vi "myRIO_BRig_RT_v0,70.vi"() -> ()   [LabVIEW 2014]
uses:
  <vilib>/Platform/TimedLoop/XDataNode/XDataNode.xnode
  <vilib>/Platform/TimedLoop/XDataNode/nitl_modes.ctl
  <vilib>/Platform/TimedLoop/XDataNode/XDNodeRunTimeDep.lvlib
  <vilib>/Platform/TimedLoop/XDataNode/wakeup.ctl
  <vilib>/Platform/TimedLoop/XDataNode/timing_clust.ctl
  <vilib>/rvi/interface/nirviReadWriteControl/nirviReadWriteControl.xnode
  <vilib>/rvi/interface/Simulation/niFpgaSimulationCallBeginRW.vi
  <vilib>/rvi/errors/niLvFpgaAdjustHostInterfaceError.vi
  <vilib>/rvi/interface/nirviCloseFPGA/nirviCloseFPGA.xnode
  <vilib>/myRIO/Instrument Drivers/Utilities/Utilities.lvlib
  <vilib>/rvi/interface/nirviOpenFPGA/nirviOpenFPGA.xnode
  myRIO_BRig_RT__Case_Exp_stateList.ctl
  <vilib>/WebDAVClient/Advanced/SessionHandle.ctl
  <vilib>/WebDAVClient/NI_WebDAV.lvlib
  myRIO_BRig_RT__Case_NonExp_stateList.ctl
  NiFpgaLv.dll
  <vilib>/Utility/error.llb/Error Cluster From Error Code.vi
  <vilib>/FPGAPlugInAG/Dynamic/niLvFpga_Close_Dynamic.vi
  myRIO_BRig_FPGA_v3,60__build.lvbitx
  myRIO_BRig_FPGA_v3,60.vi
  <vilib>/FPGAPlugInAG/myRIO-1900/niLvFpga_Open_myRIO-1900.vi
  <vilib>/rvi/interface/common/dynamic/niFpgaDynamicAddResources.vi
panel:
  out "tempAI0":u16
  out "error out 5":errorcluster
  in  "get_countPerMS":bool
  in  "count_warmup_R_reset":bool
  in  "count_warmup_L_reset":bool
  out "count_warmup_R":u16
  out "count_warmup_L":u16
  out "SolenoidReward":bool
  in  "SolenoidProbability_L":u16=50 caption="Reward Time [ms]" min=1 max=1000 step=1
  in  "SolenoidProbability_R":u16=50 caption="Reward Time [ms]" min=1 max=1000 step=1
  out "output_PortA":dbl caption="LaserPower"
  out "error out 4":errorcluster
  in  "laser_power_step":dbl
  in  "laser_power_max":dbl
  in  "Recording":bool
  out "error out 3":errorcluster
  out "error out 2":errorcluster
  in  "laser_power_min":dbl
  in  "f_millisec2count":dbl=159.0
  in  "laser_Tshutter":dbl=2.0
  in  "laser_Freq":dbl=10.0
  in  "laser_Tpeak":dbl=2.0
  in  "laser_duration":u16
  out "error out":errorcluster
  in  "LC_Cue1_All_Count":u16
  in  "LC_Cue1_First_Count":u16
  in  "LC_Cue1_All_delayOpt":bool
  in  "LC_ENL1_All_delayOpt":bool
  in  "LC_ENL1_All_Count":u16
  in  "LC_ENL1_First_Count":u16
  in  "LC_Cue1_First_delayOpt":bool
  in  "LC_ENL1_First_delayOpt":bool
  in  "Tcycle_Cue_max":u16=1000 caption="Max" min=5 max=5000 step=5
  in  "Tcycle_Cue_min":u16=1000 caption="Min" min=5 max=5000 step=5
  in  "SendData":bool
  out "cSpout":enum16{"Left", "Right"}(ring) caption="Left or Right Spout"
  out "A4":u32 caption="LickCounter_Right"
  out "A2":u32 caption="LickCounter_Left"
  in  "laserResponse_wrong_LED":bool
  out "error_initTrial":errorcluster
  out "error_Selection_pre":errorcluster
  out "error_Selection":errorcluster
  out "SelectWrong":bool
  out "SelectReward":bool
  in  "Left(F)_or_Right(T)":bool
  in  "ignoreWrong":bool
  in  "SelectionState":bool
  in  "laserResponse_wrong":bool
  in  "laserResponse_reward":bool
  in  "laserResponse_reward_LED":bool
  out "nRewards_Right":u16 caption="# Rewards Total (Right)"
  out "nRewards_Left":u16 caption="# Rewards Total (Left)"
  out "nRewards_cur":u16 caption="# Rewards in Current Block"
  out "TpB_target":u16 caption="Target Trials Per Block"
  out "cState_NonExp":T1 caption="WarmUp State"
  out "iBlock":u16 caption="Current Block"
  out "cState":T2 caption="Experimental State"
  out "iTrial":u16 caption="Current Trial"
  in  "warmupType":u8(slide) max=2 step=1 scale=0.0..2.0
  in  "TestConnection":bool
  in  "warmup":bool caption="WarmUp"
  in  "Data Set Prefix":string="Exp1_TM2"
  out "Connected To Host?":bool
  in  "Host Password":string="sabalab"
  in  "Host UserName":string="Test2"
  in  "sp_RightSpout":u16(slide)=2 max=2 step=1 scale=0.0..2.0
  in  "sp_LeftSpout":u16(slide)=2 max=2 step=1 scale=0.0..2.0
  in  "BUR_max":u16 caption="Count Reward Structure  (0 = off)"
  in  "LC_Wrong_Probability":u16
  in  "LC_Wrong_Trial":u16(slide) max=2 step=1 scale=0.0..2.0
  in  "LC_Wrong_Block":u16(slide) max=2 step=1 scale=0.0..2.0
  in  "LC_Wrong_OnOff":bool
  in  "LC_Reward_Probability":u16
  in  "LC_Reward_Trial":u16(slide) max=2 step=1 scale=0.0..2.0
  in  "LC_Reward_Block":u16(slide) max=2 step=1 scale=0.0..2.0
  in  "LC_Reward_OnOff":bool
  in  "LC_Cue1_All_Probability":u16
  in  "LC_Cue1_All_Block":u16(slide) max=2 step=1 scale=0.0..2.0
  in  "LC_Cue1_All_OnOff":bool
  in  "LC_Cue1_First_Probability":u16
  in  "LC_Cue1_First_Block":u16(slide) max=2 step=1 scale=0.0..2.0
  in  "LC_Cue1_First_OnOff":bool
  in  "LC_ENL1_All_Probability":u16 max=100 step=1
  in  "LC_ENL1_All_Block":u16(slide) max=2 step=1 scale=0.0..2.0
  in  "LC_ENL1_All_OnOff":bool
  in  "LC_ENL1_First_Probability":u16 max=100 step=1
  in  "LC_ENL1_First_Block":u16(slide) max=2 step=1 scale=0.0..2.0
  in  "Tcycle_Timeout":u16=1000 caption="Timeout Time [ms]" min=10 max=10000 step=1
  in  "Tcycle_Wrong":u16=1000 caption="Wrong Time [ms]" min=10 max=10000 step=1
  in  "Tcycle_Selection":u16=1000 caption="Answer Time [ms]" min=1 max=10000 step=1
  in  "Tcycle_RewardPost":u16=1000 caption="Consumption Time [ms]" min=250 max=10000 step=250
  in  "Tcycle_Reward_L":u16=500 caption="Reward Time [ms]" min=1 max=1000 step=1
  in  "Tcycle_Reward_R":u16=500 caption="Reward Time [ms]" min=1 max=1000 step=1
  in  "TpB_Max_R":u16=4 caption="Max TrialsPerBlock" min=1 max=12 step=1
  in  "TpB_Min_R":u16=4 caption="Min TrialsPerBlock" min=1 max=12 step=1
  in  "TpB_Max_L":u16=4 caption="Max TrialsPerBlock" min=1 max=12 step=1
  in  "TpB_Min_L":u16=4 caption="Min TrialsPerBlock" min=1 max=12 step=1
  in  "BUR_min":u16 caption="Count Reward Structure\n(0 = off)"
  in  "TrialUntilReward":bool caption="Ignore Wrong Selection"
  in  "CueCycles":u16=1 caption="Cue Structure" min=1 max=1 step=1
  in  "MTrig_Laser_Tcycle":u16=10 caption="Time [ms]"
  in  "MTrig_Laser_trig":bool
  in  "MTrig_Audio_trig__R":bool caption="Trigger Audio"
  in  "MTrig_Audio_trig__L":bool caption="Trigger Audio"
  in  "RewCalib_Trig_R":bool caption="Calibrate_R"
  in  "RewCalib_Trig_L":bool caption="Calibrate_L"
  in  "MTrig_Solenoid_Tcycle__R":u16=300 caption="Time [ms]"
  in  "MTrig_Solenoid_Tcycle__L":u16=300 caption="Time [ms]"
  in  "MTrig_Solenoid_trig__R":bool caption="Solenoid"
  in  "MTrig_Solenoid_trig__L":bool caption="Solenoid"
  in  "STOP_abort":bool caption="Stop LabView\n(Stops myRio and FPGA)"
  in  "STOP_endBlock":bool caption="Stop Experiment\n@ End of Block"
  in  "STOP_endTrial":bool caption="Stop Experiment\n@ End of Trial"
  in  "START":bool caption="Start Experiment"
  in  "Tcycle_CuePenalty":u16=1000 caption="Penalty" min=1 max=10000 step=1
  in  "Audio_Amp__R":u16=100 caption="Amp"
  in  "Audio_Freq__R":u8=5 caption="Freq [kHz]" max=14 step=1
  in  "Audio_Amp__L":u16=100 caption="Amp"
  in  "Audio_Freq__L":u8=5 caption="Freq [kHz]" max=14 step=1
  in  "LC_Wrong_Tdelay":u16
  in  "LC_Cue1_All_Tdelay":u16
  in  "LC_ENL1_All_Tdelay":u16
  in  "LC_Reward_Tdelay":u16
  in  "LC_Cue1_First_Tdelay":u16
  in  "LC_ENL1_First_Tdelay":u16
  in  "LC_ENL1_First_OnOff":bool
  in  "Tcycle_ENLPenalty":u16=100 caption="Penalty" min=10 max=10000 step=10
  in  "Tcycle_ENL_max":u16=1000 caption="Max" min=250 max=10000 step=250
  in  "Tcycle_ENL_min":u16=1000 caption="Min" min=250 max=10000 step=250
  # "Experimental Run"
  # "Experiment Task Structure"
  # "Current State"
  # "Timing [ms]"
  # "Global Parameters\n \n   WarmUp State                                            Lick Counter"
  # "Min            Max            Penalty"
  # "(1) = Switching\n(2) = Two Choice"
  # "Enforced\nNonLick"
  # "Left                    Right"
  # "Cue"
  # "Experimental State"
  # "Communication (Host PC)"
  # "WarmUp"
  # "Selection\n \n \nReward\n    Dispense\n    Time\n \n    Dispense\n    Probability\n \n    Consumption\n    Time\n \nWrong Choice\n \n \nTimeout Penalty"
  # "Trial Parameters\n \n   Left/Right        Give Reward?        Laser Power [V]"
  # "Left                  Right"
  # "Min"
  # "Max"
  # "Block                   Trial            Target Trials       # Rewards \n                                                            Per Block             Current"
  # "Trial Per Block Structure \n               Left                        Right"
  # "Min"
  # "# Rewards Total\n                                                                  Left                    Right"
  # "Recording Rig"
  # "FPGA Conv."
  # "Cue then reward (no lick)\n \nLeft                    Right"
  # "Max"
  # "FPGA count per ms"
  # "Laser Control\n\n                               On/Off      Block        Probability [%]   Delay [ms]                              Count"
  # "Manual Control"
  # "Enforced\nNonLick\n      1"
  # "Solenoid\n \nLeft              Right"
  # "Speaker\n \nLeft                    Right"
  # "Laser"
  # "from end"
  # "Switch\nTrial"
  # "from start"
  # "from end"
  # "NonSwitch\nTrials"
  # "Time\n[ms]"
  # "Time\n[ms]"
  # "from start"
  # "Time = Cue Min"
  # "Cue 1"
  # "Power = Min"
  # "from end"
  # "Switch\nTrial"
  # "from start"
  # "Speaker Parameters"
  # "Laser Parameters"
  # "Left                  Right"
  # "from end"
  # "Frequency\n[Hz]"
  # "NonSwitch\nTrials"
  # "Frequency\n[kHz]"
  # "from start"
  # "Timing [ms]\n Duration     Peak Width   Shutter"
  # "Selection Reward"
  # "Amp\n(0 - 32,000)"
  # "Laser Power [V]\nMin          Max              Step"
  # "Speaker\nPattern\nDuring Cue"
  # "Selection Wrong"
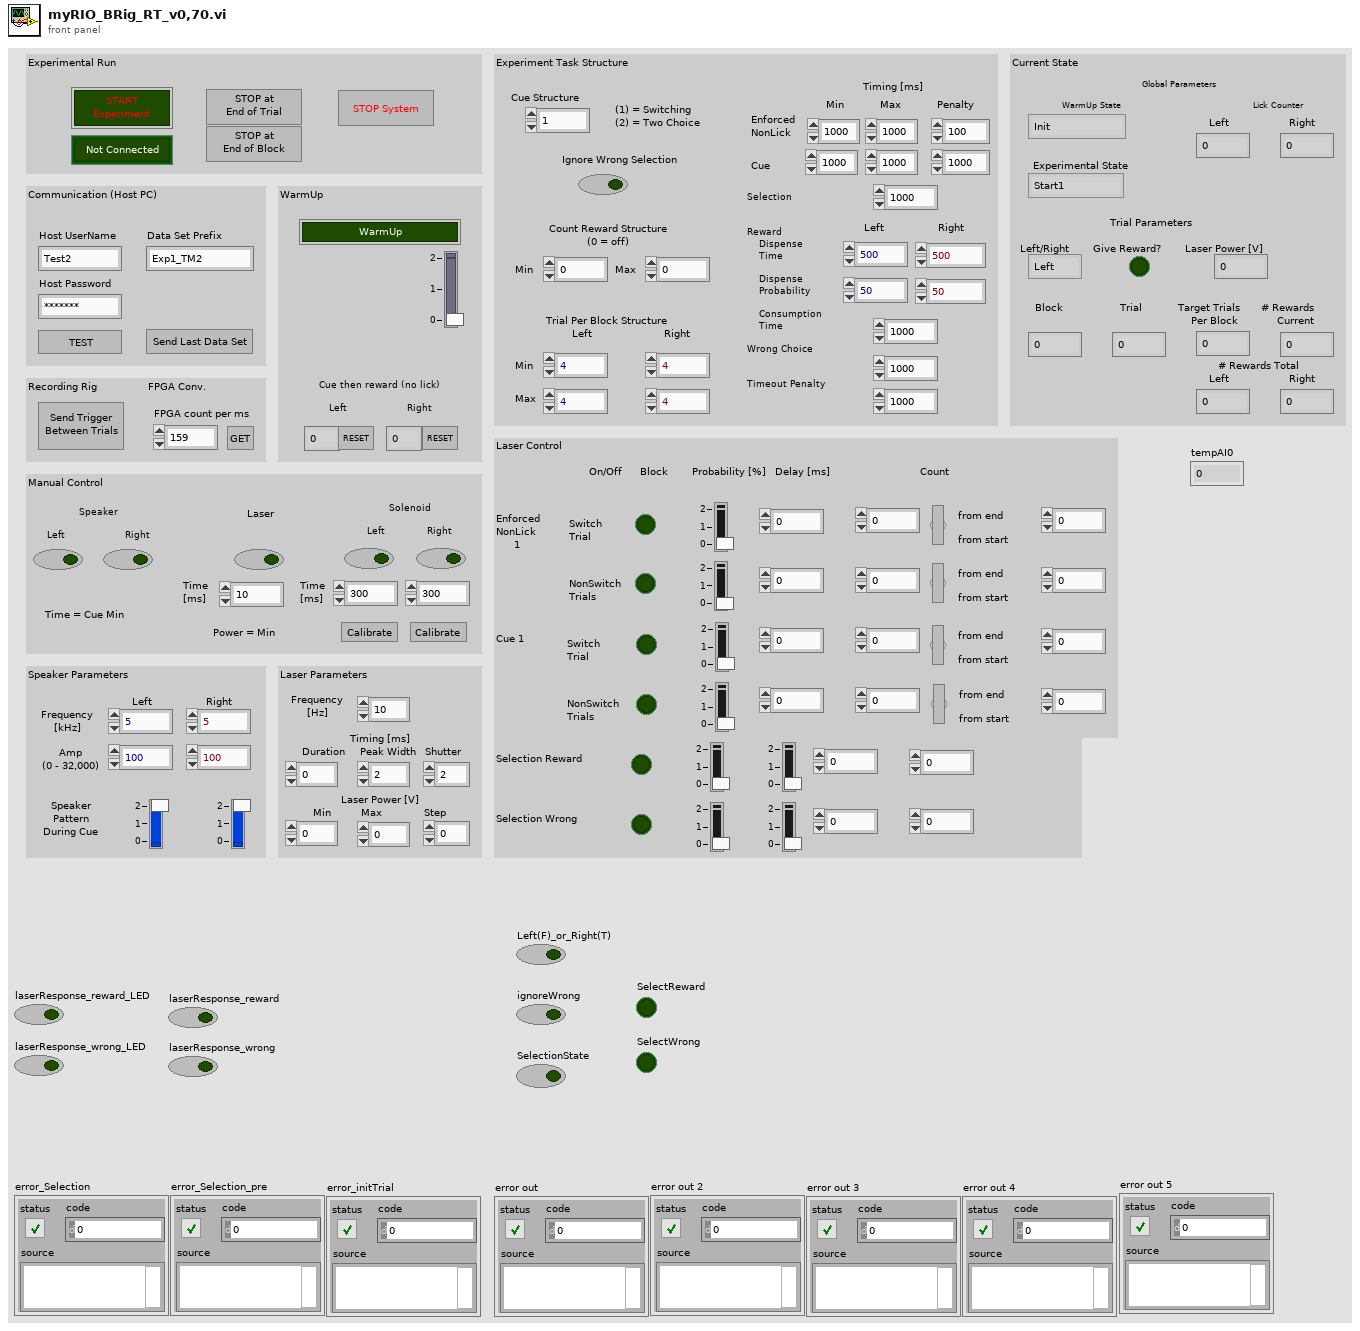
[diagram p1: front panel]
types:
  T1 = typedef "myRIO_BRig_RT__Case_NonExp_stateList.ctl" = enum16{"Init", "UploadSettings_pre", "UploadSettings_Read_dataExp", "UploadSettings_dataExp_1", "UploadSettings_Read_dataLC", "UploadSettings_dataLC_1", "UploadSettings_dataLC_2", "UploadSettings_Read_dataMTrig", "UploadSettings_dataMTrig_1", "UploadSettings_post", "Idle_pre", "IdleEmpty", "IdleEmpty2", "IdleEmpty3", "IdleEmpty4", "Idle", "Idle_2", "Idle_3", "Idle_4", "Idle_post", "Cue_pre__pre", "Cue_pre", "Cue", "Cue_post", "RewardCalibration_pre", "DispenseWater_pre__pre", "DispenseWater_pre", "DispenseWater", "DispenseWater_post", "TestConnection", "SendData", "Get_FPGA_count_per_ms", "End"}
  T2 = typedef "myRIO_BRig_RT__Case_Exp_stateList.ctl" = enum16{"Start1", "Start2", "Start3", "saveSettings1", "saveSettings2", "saveSettings3", "saveSettings4_LC_ENL", "saveSettings5_LC_Cue", "saveSettings6_LC_Other", "setSettings_Audio", "setSettings_Laser", "initBlock_pre", "initBlock", "initBlock2", "initBlock_post", "initTrial_pre", "initTrial", "initTrial2", "initTrial3", "initTrial4", "initTrial_LC_ENL1", "initTrial_LC_Cue1", "initTrial_LC_Sel", "initTrial_post", "ENL1_pre", "ENL1", "ENL1_post", "ENL1Penalty_pre", "ENL1Penalty", "ENL2_pre", "ENL2", "ENL2Penalty_pre", "ENL2Penalty", "Cue1_pre", "Cue1", "Cue1_post", "Cue1Penalty_pre", "Cue1Penalty", "Cue2_pre", "Cue2", "Cue2Penalty_pre", "Cue2Penalty", "Selection_pre", "Selection", "Select_post", "SelectReward_pre", "SelectReward", "SelectRewardPost_pre", "SelectRewardPost", "SelectWrong_pre", "SelectWrong", "SelectWrong_post", "SelectTimeout_pre", "SelectTimeout", "SelectTimeout_post", "endTrial_pre", "endTrial1", "endTrial2", "endTrial3", "endTrial_post", "endBlock_pre", "endBlock", "endBlock_post", "endExp", "commConnect", "commUpload_pre", "commUpload_dataBlock", "commUpload_dataCurrent", "commUpload_dataExp", "commUpload_dataLC", "commUpload_dataTrial", "commUpload_post", "saveData_pre", "saveData_dataBlock", "saveData_dataCurrent", "saveData_dataExp", "saveData_dataLC", "saveData_dataTrial", "saveData_post", "empty_endBlock1", "empty_endBlock2", "empty_endTrial1", "empty_endTrial2", "empty_endTrial3", "empty_endTrial4", "empty_endTrial5"}
  T3 = typedef "XDNodeRunTimeDep.lvlib/timing_clust.ctl" = cluster{"Expected End [f-1]":u64, "Actual End [f-1]":u64, "Finished Late? [f-1]":bool, "Expected End [i-1]":u64, "Actual End [i-1]":u64, "Finished Late? [i-1]":bool, "Expected Start [i]":u64, "Actual Start [i]":u64, "Expected Start [f]":u64, "Actual Start [f]":u64, "Source Name":string, "Structure Name":string, "Period":i64, "Deadline":i64, "Offset":i64, "Start":i64, "Priority":i32, "Timeout":i32, "Mode":T4, "Wakeup Reason":T5, "Error":errorcluster, "Source Type":string, "Secondary Source Type":string, "Global End Time":u64, "Global Start Time":u64, "Frame Duration":u64, "Iteration Duration":u64, "Assigned CPU":i32, "I/O Scan Engine Mode":u32}
  T4 = typedef "XDNodeRunTimeDep.lvlib/nitl_modes.ctl" = enum32{"No Change", "Process missed periods, maintain original phase", "Discard missed periods, maintain original phase", "Process missed periods, ignore original phase", "Discard missed periods, ignore original phase"}
  T5 = typedef "XDNodeRunTimeDep.lvlib/wakeup.ctl" = enum32{"Normal", "Aborted", "Asynchronous wakeup", "Timing source error", "Timed loop error", "Timeout"}
  T6 = typedef "NI_WebDAV.lvlib/SessionHandle.ctl" = refnum<k1>
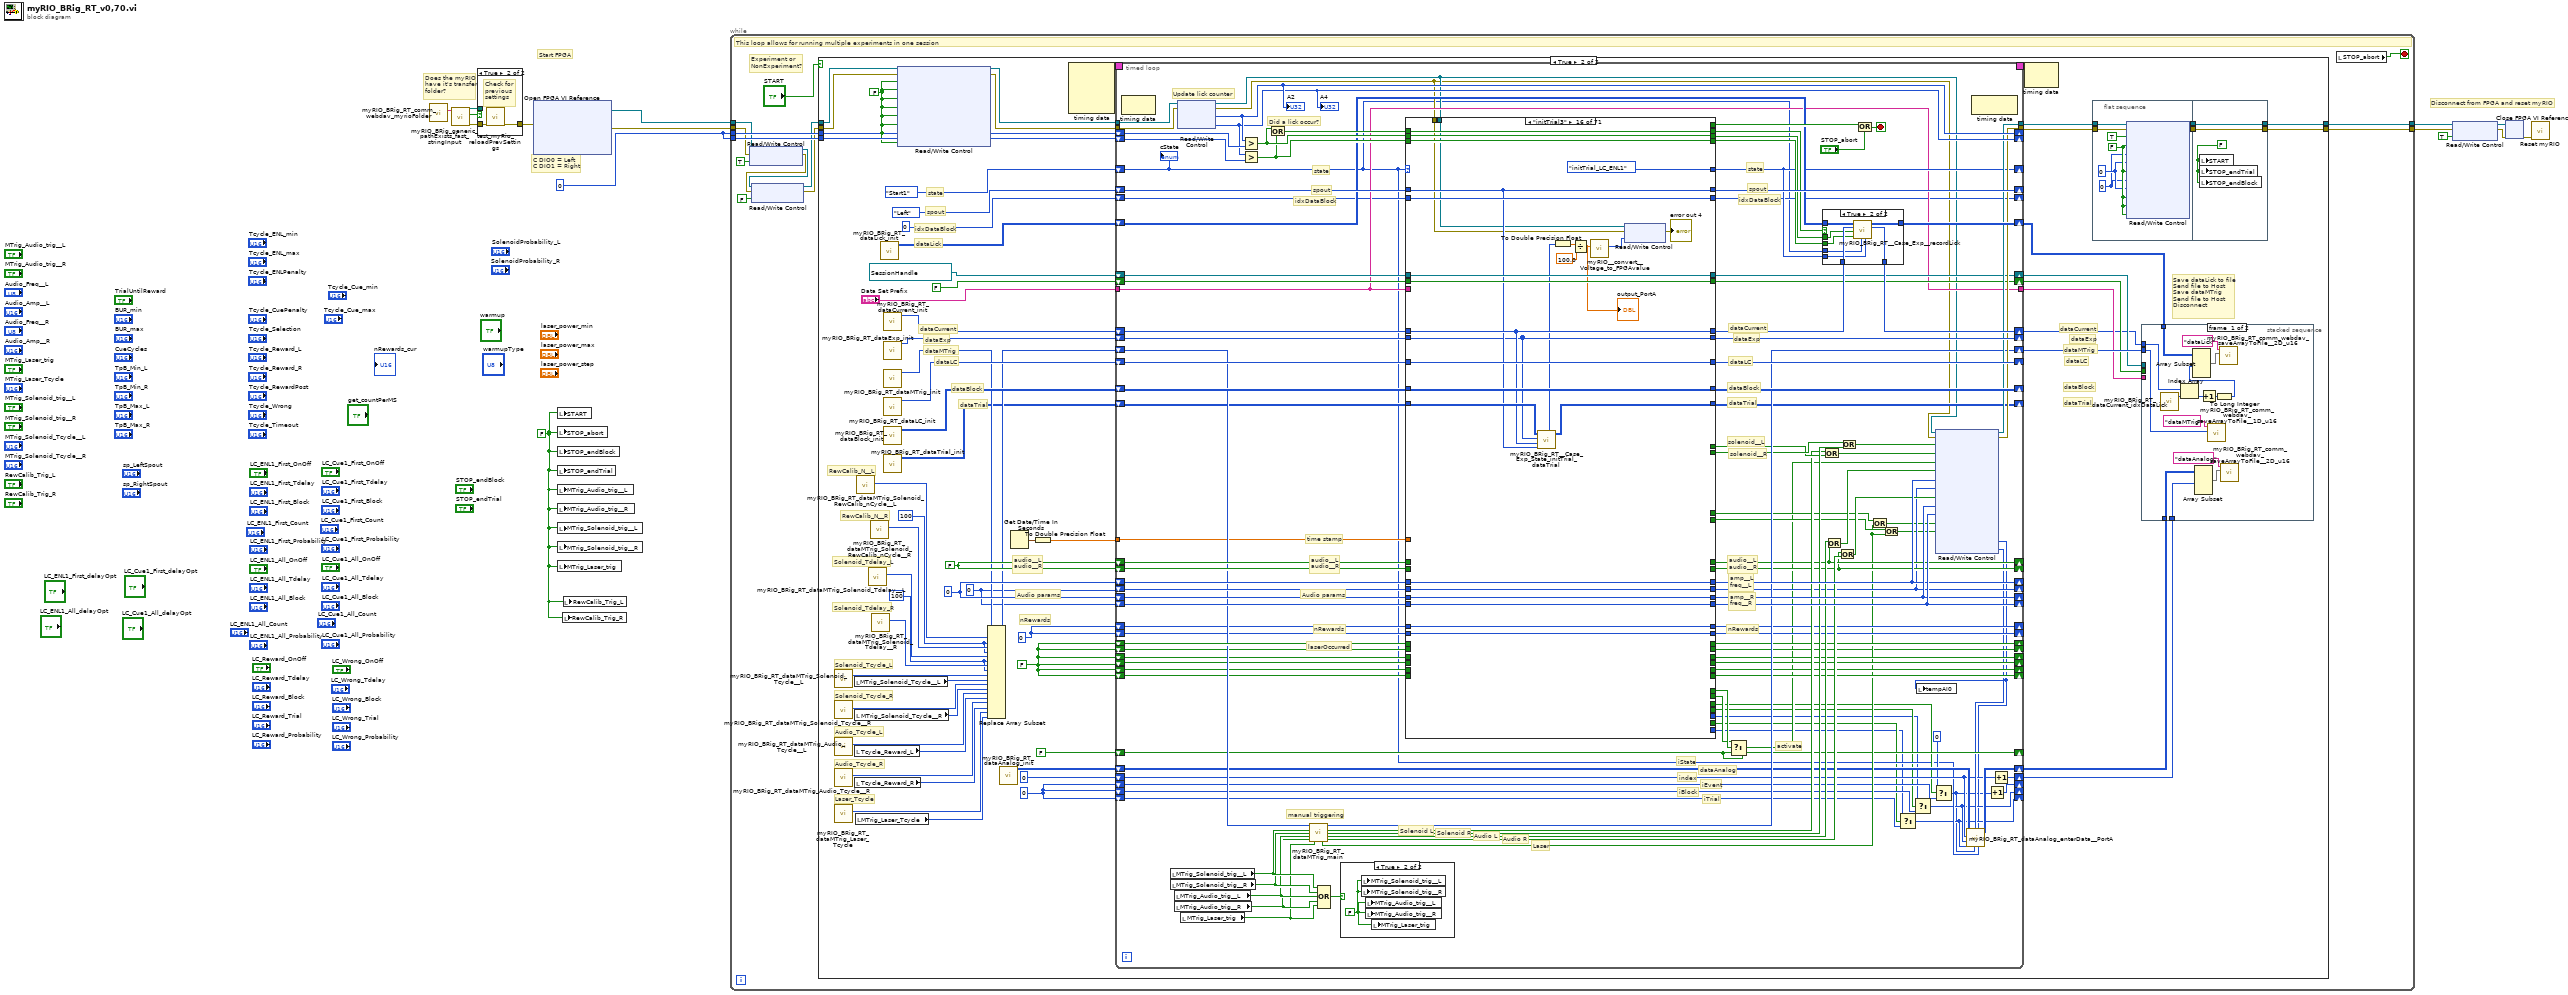
[diagram p0: block diagram]
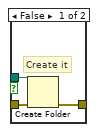
[diagram p2: hidden frame]
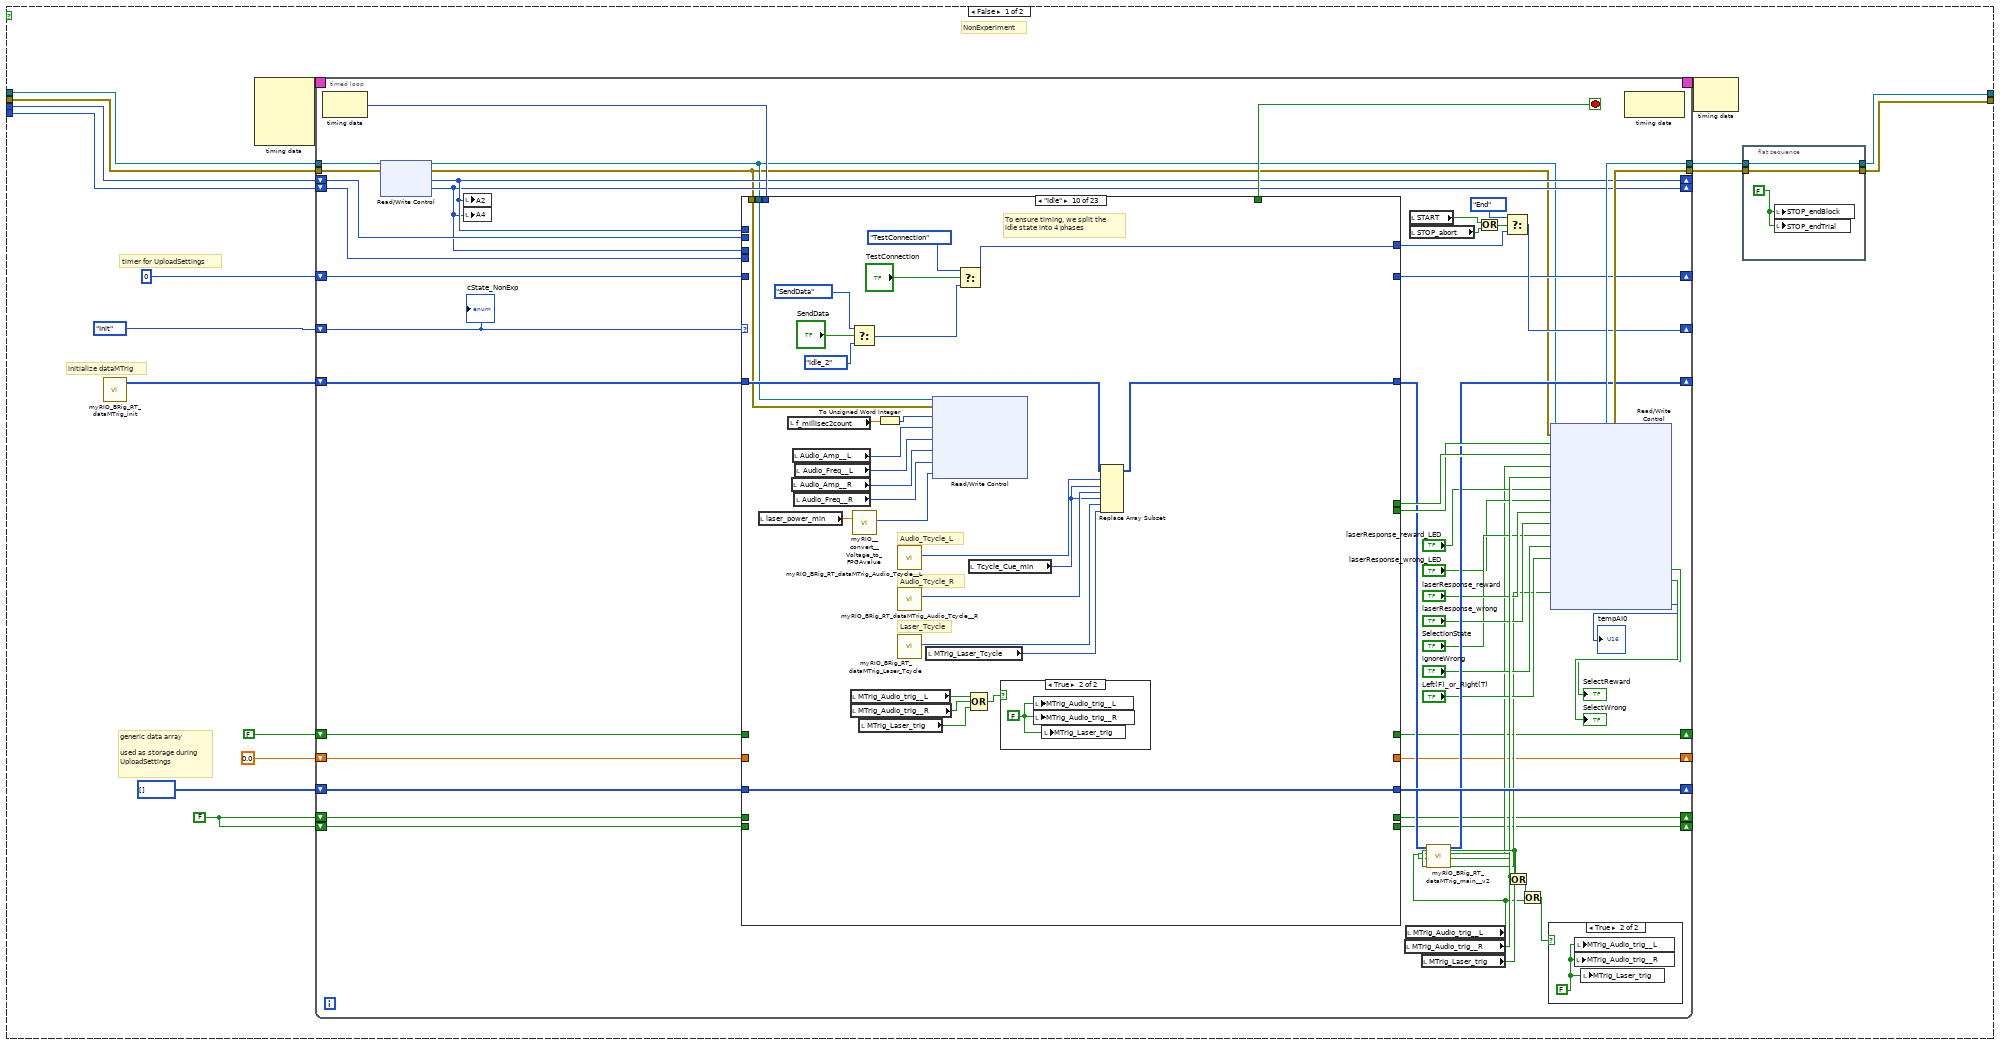
[diagram p3: hidden frame]
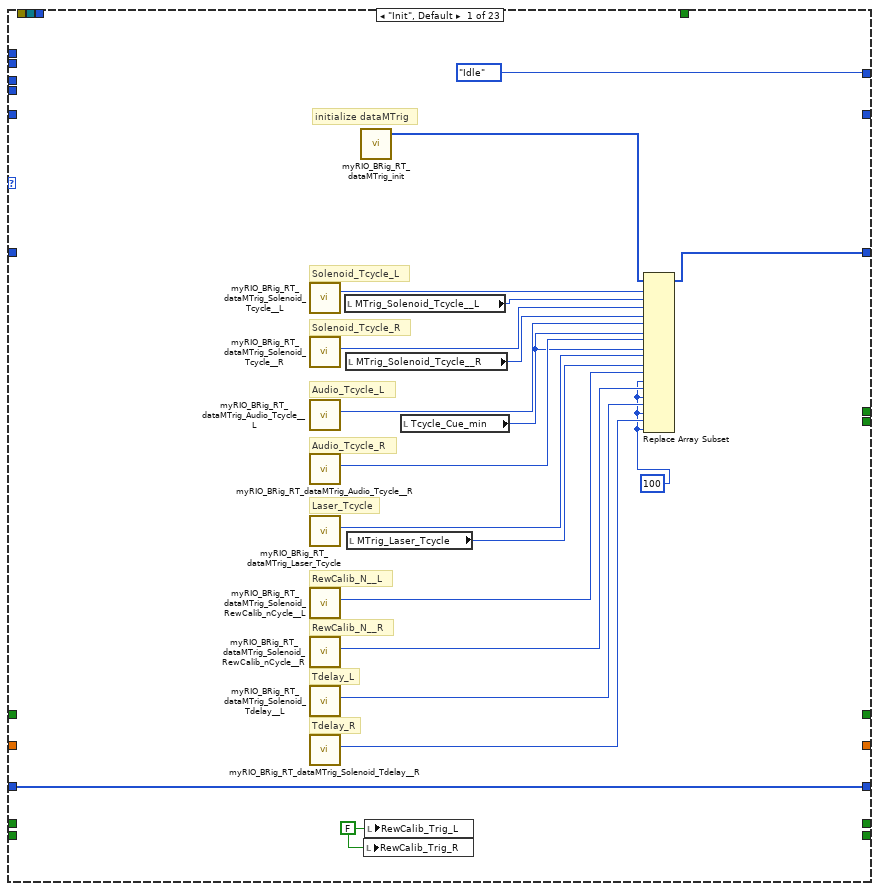
[diagram p5: hidden frame]
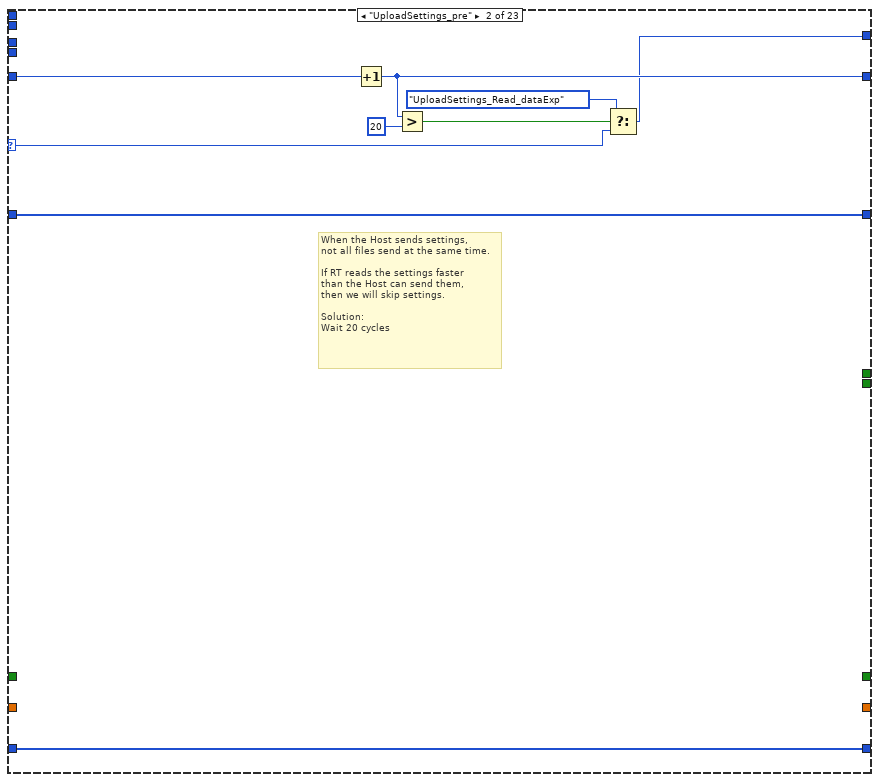
[diagram p6: hidden frame]
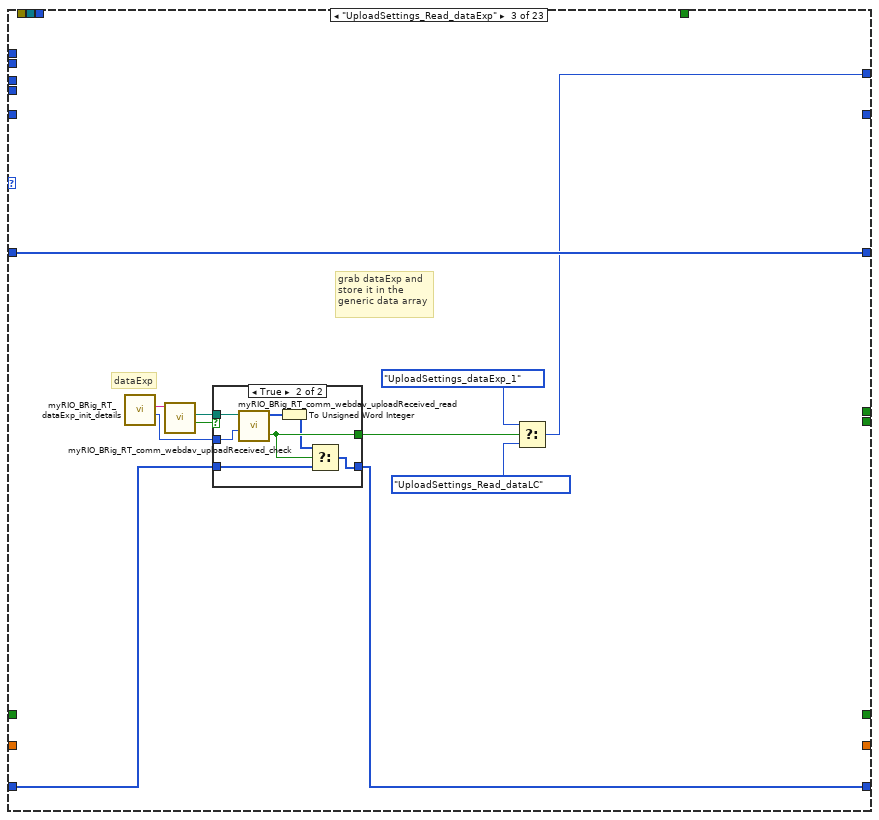
[diagram p7: hidden frame]
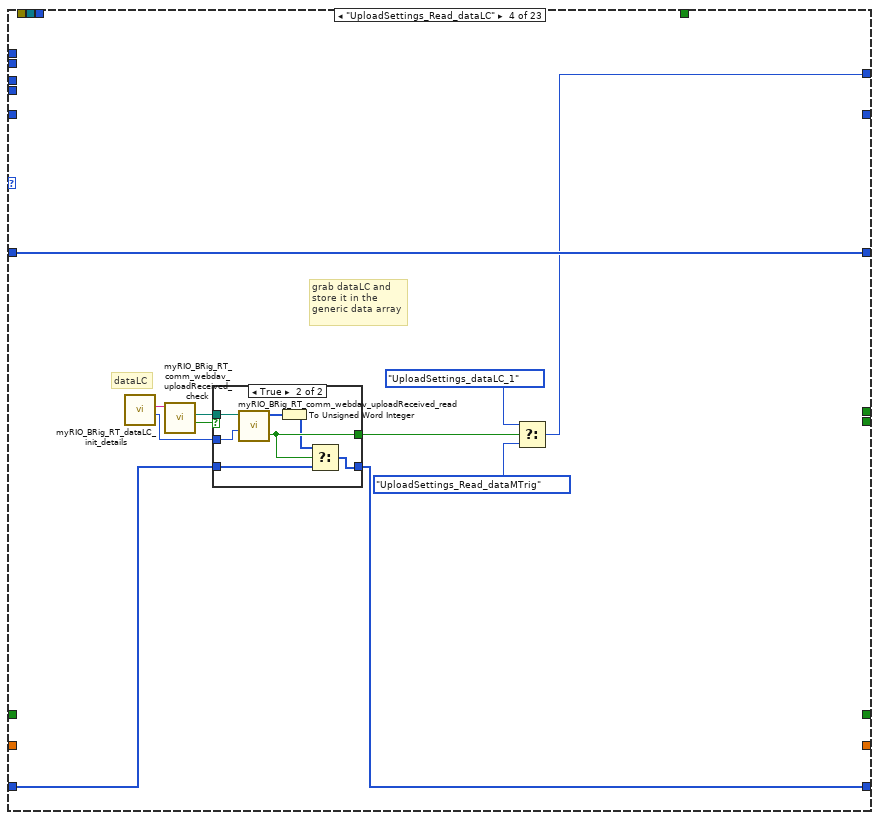
[diagram p9: hidden frame]
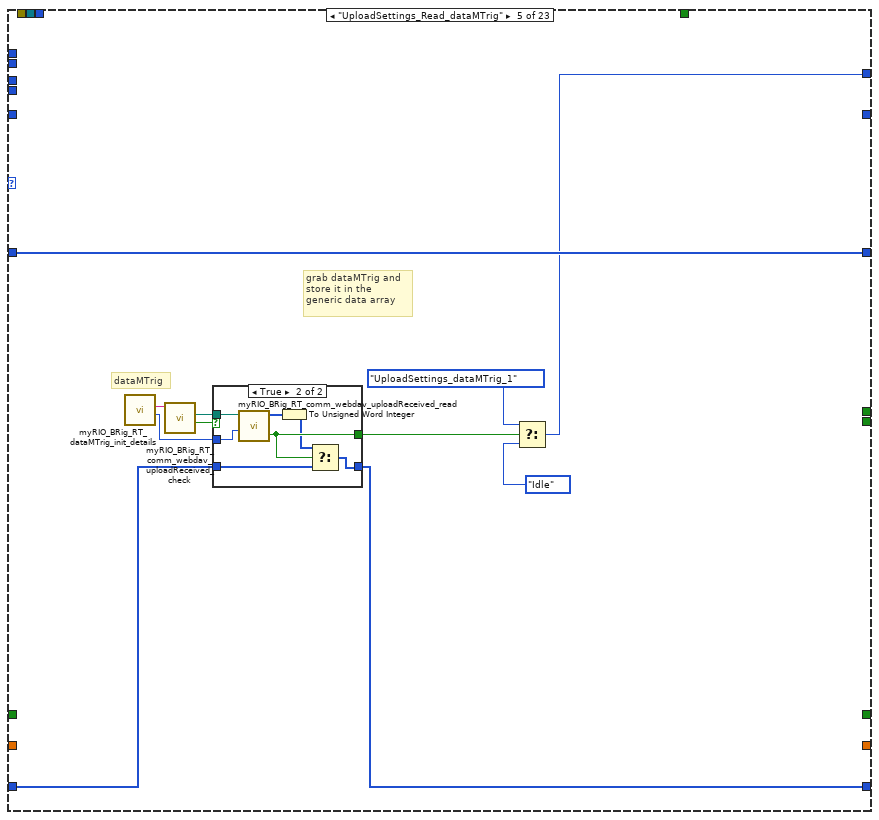
[diagram p11: hidden frame]
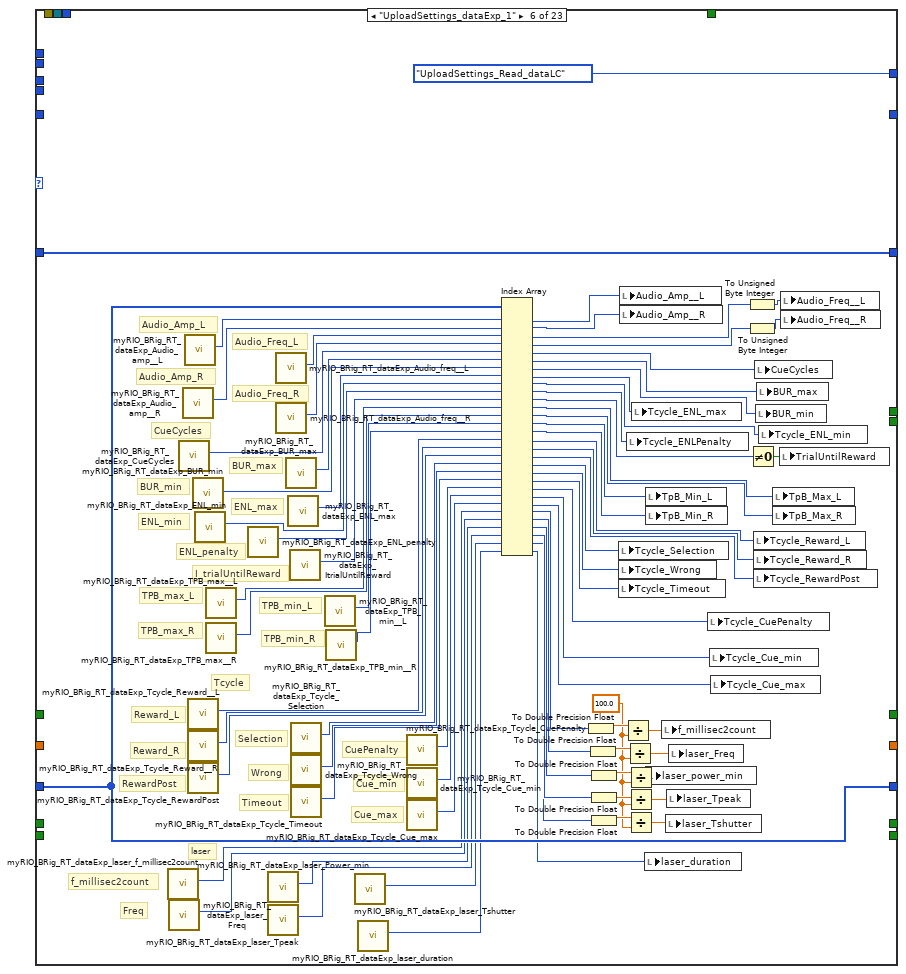
[diagram p13: hidden frame]
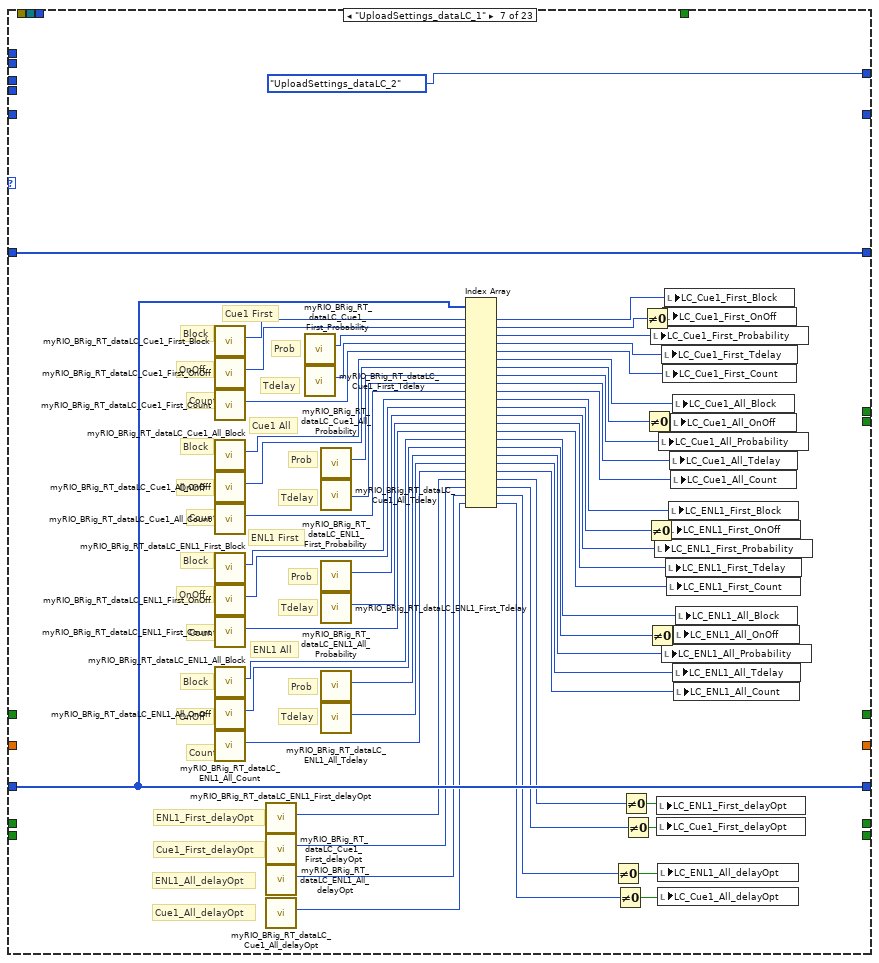
[diagram p14: hidden frame]
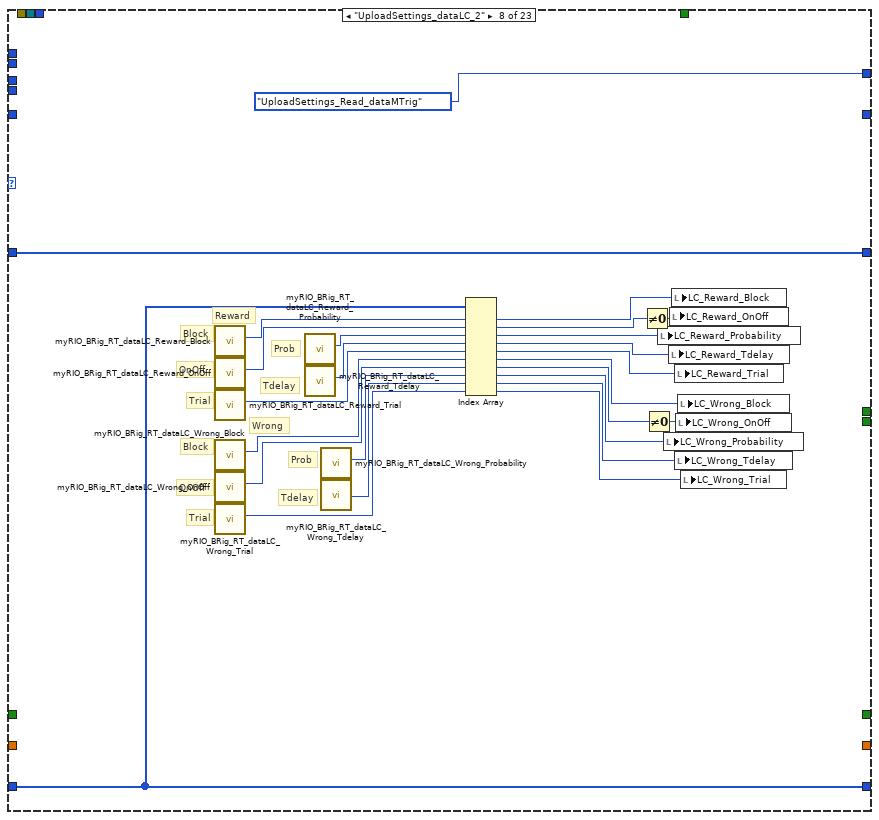
[diagram p15: hidden frame]
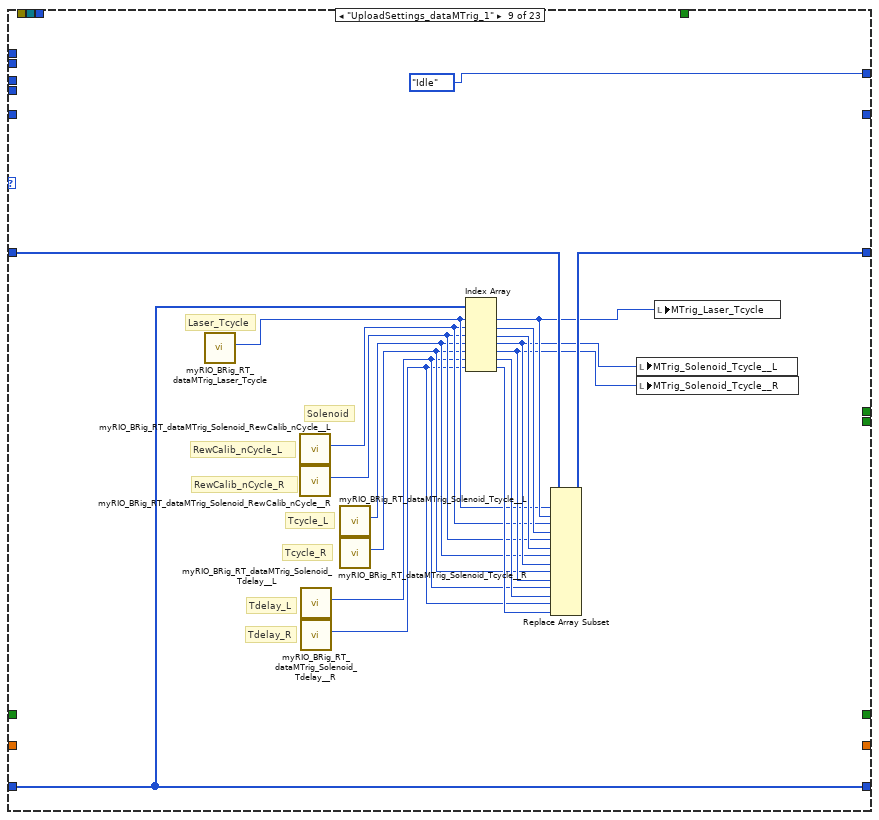
[diagram p16: hidden frame]
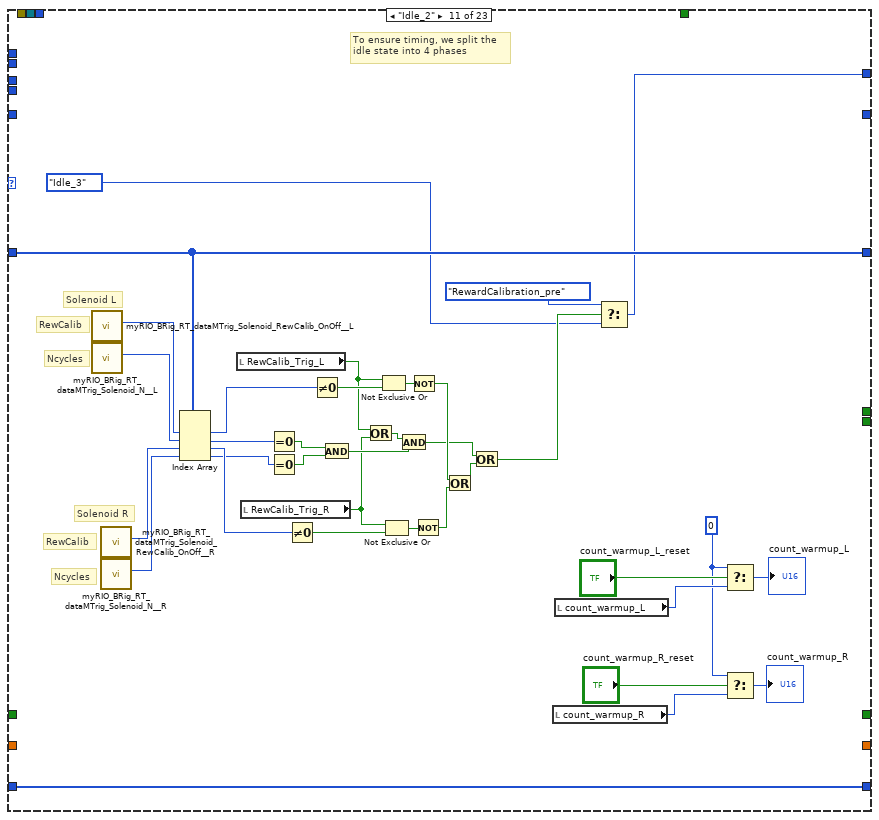
[diagram p18: hidden frame]
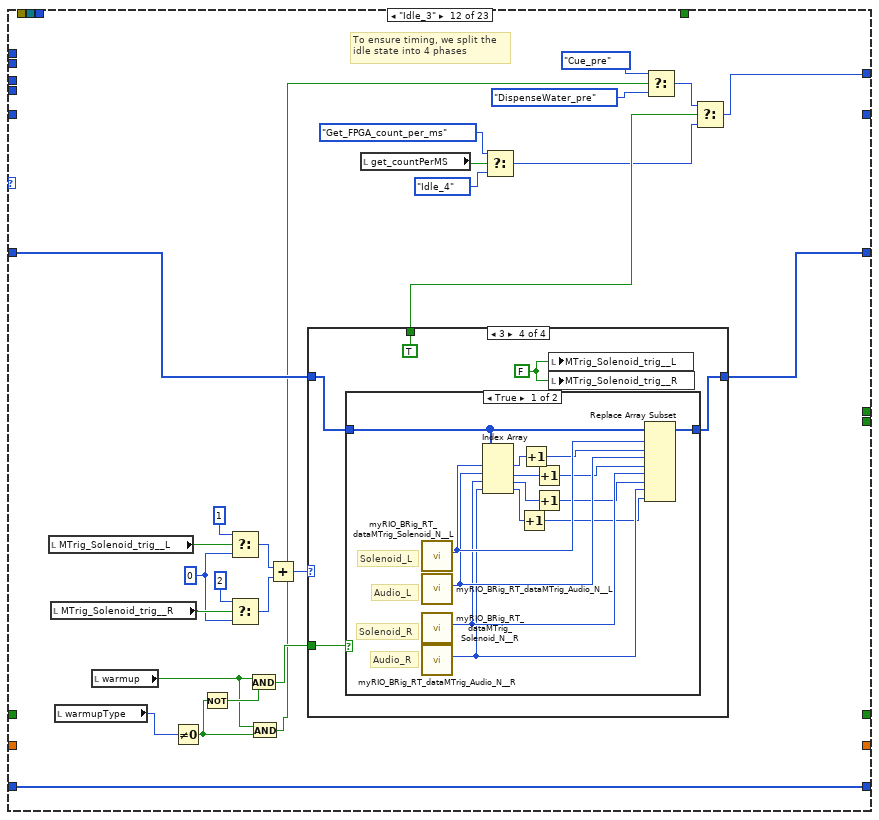
[diagram p19: hidden frame]
diagram:
  w9 = u32 0
  w6 = FALSE
  # "Does the myRIO\nhave it's transfer\nfolder?"
  # "C DIO0 = Left\nC DIO1 = Right"
  # "Start FPGA"
  # "Disconnect from FPGA and reset myRIO"
  n1 = call "myRIO_BRig_RT_comm_webdav_myrioFolder.vi"() -> ("output_myrioFolder"=w4:string)  [unwired: 11 in]
  n2 = call "myRIO_BRig_generic_pathExists_fast_stringInput.vi"("input_filePath"=w4) -> ("output_error"=w3:errorcluster, "output_Iexist"=w2:bool, "output_filePath"=w1:path)  [unwired: 8 in]
  n3 = case shown="True" w2 {
    tunnel: w1 -> [w18 _]
    tunnel: w3 -> [w17 w20]
    tunnel: [w16 w19] -> w5
    frame False {
      # "Create it"
      n4 = Create Folder(path (use dialog)=w18, error in=w17) -> (error out=w16:errorcluster)  [unwired: 1 in, 2 out]
    }
    frame True {
      # "Check for\nprevious\nsettings"
      n5 = call "test_myRio_reloadPrevSettings.vi"("input_error"=w20) -> ("output_error"=w19:errorcluster)  [unwired: 10 in]
    }
  }
  n6 = xnode "Open FPGA VI Reference"("error in"=w5) -> ("FPGA VI Reference Out"=w11:refnum<k20>, "error out"=w10:errorcluster)  [unwired: 1 in]
  n7 = local write "START"(w6) -> ()
  n8 = local write "STOP_abort"(w6) -> ()
  n9 = local write "STOP_endBlock"(w6) -> ()
  n10 = local write "STOP_endTrial"(w6) -> ()
  n11 = local write "MTrig_Audio_trig__L"(w6) -> ()
  n12 = local write "MTrig_Audio_trig__R"(w6) -> ()
  n13 = local write "MTrig_Solenoid_trig__L"(w6) -> ()
  n14 = local write "MTrig_Solenoid_trig__R"(w6) -> ()
  n15 = local write "MTrig_Laser_trig"(w6) -> ()
  n16 = local write "RewCalib_Trig_R"(w6) -> ()
  n17 = local write "RewCalib_Trig_L"(w6) -> ()
  n18 = while {
    tunnel: w11 -> [w24]
    tunnel: w10 -> [w29]
    tunnel: w9 -> [w32]
    tunnel: w9 -> [w31]
    tunnel: [w22] -> w8
    tunnel: [w21] -> w7
    stop <- w30 stop-if-true
    # "Experiment or\nNonExperiment?"
    # "This loop allows for running multiple experiments in one session"
    n19 = xnode "Read/Write Control"("FPGA VI Reference In"=w24, "error in"=w29, "Counts_Reset"=TRUE) -> ("FPGA VI Reference Out"=w26:refnum<k20>, "error out"=w27:errorcluster)
    n20 = xnode "Read/Write Control"("FPGA VI Reference In"=w26, "error in"=w27, "Counts_Reset"=FALSE) -> ("FPGA VI Reference Out"=w23:refnum<k20>, "error out"=w25:errorcluster)
    n21 = case shown="True" "START" {
      tunnel: w32 -> [w47 w957]
      tunnel: w31 -> [w46 w956]
      tunnel: w25 -> [w44 w907]
      tunnel: w23 -> [w45 w906]
      tunnel: [w42 w953] -> w22
      tunnel: [w40 w948] -> w21
      frame False {
        w37 = FALSE
        # "generic data array\n\nused as storage during\nUploadSettings"
        # "timer for UploadSettings"
        # "initialize dataMTrig"
        # "NonExperiment"
        n22 = call "myRIO_BRig_RT_dataMTrig_init.vi"() -> ("output_dataMTrig"=w48:u16[])  [unwired: 5 in]
        n23 = node-c288() -> (w51:T3)  [unwired: 4 in]
        n24 = timed-loop {
          timing: w51 -> [_]
          timing-out: [_] -> w50
          shift-right: [w95] -> _
          shift-left: w48 -> [w107]
          shift-right: [w84] -> _
          shift-left: myRIO_BRig_RT__Case_NonExp_stateList."Init" ("Enum") -> [w101]
          shift-right: [w68] -> _
          shift-left: w47 -> [w69]
          shift-right: [w66] -> _
          shift-left: w46 -> [w67]
          tunnel: [w103] -> w43
          tunnel: [w102] -> w41
          tunnel: w44 -> [w105]
          tunnel: w45 -> [w104]
          shift-right: [w100] -> _
          shift-left: u16[] [] ("output_data") -> [w99]
          shift-right: [w70] -> _
          shift-left: u16 0 ("Audio_Amp__L") -> [w71]
          shift-right: [w63] -> _
          shift-left: w37 -> [w65]
          shift-right: [w62] -> _
          shift-left: w37 -> [w64]
          shift-right: [w58] -> _
          shift-left: FALSE -> [w59]
          shift-right: [w56] -> _
          shift-left: 0.0 -> [w57]
          stop <- w108 stop-if-true
          n25 = node-c288() -> (w106:i64)  [unwired: 1 in]
          n26 = xnode "Read/Write Control"("FPGA VI Reference In"=w104, "error in"=w105) -> ("FPGA VI Reference Out"=w61:refnum<k20>, "error out"=w60:errorcluster, "A2_LickL"=w68:u32, "A4_LickR"=w66:u32)
          n27 = local write "A2"(w68) -> ()
          n28 = local write "A4"(w66) -> ()
          n29 = case shown="\"Idle\"" w101 {
            selector: w101 -> [_ w133 _ _ _ _ _ _ _ _ _ _ _ _ w564 _ _ w772 _ _ _ w847 w891]
            tunnel: [myRIO_BRig_RT__Case_NonExp_stateList."Idle" ("Enum") w131 w138 w157 w176 myRIO_BRig_RT__Case_NonExp_stateList."UploadSettings_Read_dataLC" ("Enum") myRIO_BRig_RT__Case_NonExp_stateList."UploadSettings_dataLC_2" ("Enum") myRIO_BRig_RT__Case_NonExp_stateList."UploadSettings_Read_dataMTrig" ("f") myRIO_BRig_RT__Case_NonExp_stateList."Idle" ("Enum") w395 w412 w451 w532 myRIO_BRig_RT__Case_NonExp_stateList."Cue" ("t") w559 myRIO_BRig_RT__Case_NonExp_stateList."DispenseWater_pre" ("Enum") w717 w770 w793 myRIO_BRig_RT__Case_NonExp_stateList."Idle" ("Enum") myRIO_BRig_RT__Case_NonExp_stateList."Idle" ("Enum") w846 w891] -> w85
            tunnel: [w120 w130 w148 w167 w186 w271 w330 w355 w371 w399 w427 w456 w530 w548 w565 w627 w754 w777 w804 w839 w845 w858 w889] -> w96
            tunnel: [_ _ _ _ _ _ _ _ _ _ _ _ _ _ _ _ _ _ _ _ _ _ TRUE] -> w108
            tunnel: w107 -> [_ w130 w148 w167 w186 w271 w330 w355 w372 w398 w427 w457 w530 w549 w566 w613 w750 w778 w805 w839 w845 w858 w889]
            tunnel: w106 -> [_ _ _ _ _ _ _ _ _ _ _ _ _ _ _ _ _ w782 _ _ _ _ _]
            tunnel: [w113 w129 w139 w158 w177 w220 w286 w331 w356 w390 w411 w445 w529 w538 w573 w608 w702 w755 w786 w831 w843 w857 w888] -> w100
            tunnel: w99 -> [w113 w129 w140 w159 w178 w220 w286 w331 w356 w390 w411 w445 w529 w538 w573 w608 w702 w755 w786 w831 w843 w857 w888]
            tunnel: [_ _ _ _ _ _ _ _ _ _ _ _ _ _ _ _ _ w779 _ _ _ _ _] -> w98
            tunnel: [_ _ _ _ _ _ _ _ _ _ _ _ _ _ _ _ _ w761 _ _ _ _ _] -> w97
            tunnel: w71 -> [_ w137 _ _ _ _ _ _ _ _ _ _ _ _ _ _ _ _ _ _ _ _ _]
            tunnel: [_ w136 _ _ _ _ _ _ _ _ _ _ _ _ _ _ _ _ _ _ _ _ _] -> w70
            tunnel: w69 -> [_ _ _ _ _ _ _ _ _ _ _ _ _ _ w570 _ _ _ _ _ _ _ _]
            tunnel: w68 -> [_ _ _ _ _ _ _ _ _ _ _ _ _ _ w571 _ _ _ _ _ _ _ _]
            tunnel: w67 -> [_ _ _ _ _ _ _ _ _ _ _ _ _ _ w568 _ _ _ _ _ _ _ _]
            tunnel: w66 -> [_ _ _ _ _ _ _ _ _ _ _ _ _ _ w569 _ _ _ _ _ _ _ _]
            tunnel: w65 -> [_ _ _ _ _ _ _ _ _ _ _ _ _ _ w556 _ _ _ _ _ _ _ _]
            tunnel: w64 -> [_ _ _ _ _ _ _ _ _ _ _ _ _ _ w555 _ _ _ _ _ _ _ _]
            tunnel: [_ _ _ _ _ _ _ _ _ _ _ _ _ w537 w556 _ _ _ _ _ _ _ _] -> w63
            tunnel: [_ _ _ _ _ _ _ _ _ _ _ _ _ w536 w555 _ _ _ _ _ _ _ _] -> w62
            tunnel: w61 -> [_ _ _ _ _ _ _ _ _ w381 _ _ _ _ _ _ _ _ _ _ _ w852 _]
            tunnel: w60 -> [_ _ _ _ _ _ _ _ _ w380 _ _ _ _ _ _ _ _ _ _ _ w851 _]
            tunnel: w59 -> [_ _ _ _ _ _ _ _ _ _ _ _ _ _ _ _ _ _ _ _ _ w856 _]
            tunnel: [_ _ _ _ _ _ _ _ _ _ _ _ _ _ _ _ _ _ _ _ _ TRUE _] -> w58
            tunnel: w57 -> [_ _ _ _ _ _ _ _ _ _ _ _ _ _ _ _ _ _ _ _ _ w854 _]
            tunnel: [_ _ _ _ _ _ _ _ _ _ _ _ _ _ _ _ _ _ _ _ _ w853 _] -> w56
            frame "Init", Default {
              w114 = FALSE ("RewCalib_Trig_L")
              w110 = u16 100 ("new element/subarray")
              # "Tdelay_R"
              # "Tdelay_L"
              # "RewCalib_N__R"
              # "RewCalib_N__L"
              # "Solenoid_Tcycle_R"
              # "Solenoid_Tcycle_L"
              # "Laser_Tcycle"
              # "Audio_Tcycle_R"
              # "Audio_Tcycle_L"
              # "initialize dataMTrig"
              n30 = call "myRIO_BRig_RT_dataMTrig_Solenoid_Tcycle__L.vi"() -> ("output_Solenoid_Tcycle__L"=w122:i32)  [unwired: 11 in]
              n31 = call "myRIO_BRig_RT_dataMTrig_Solenoid_Tcycle__R.vi"() -> ("output_Solenoid_Tcycle__R"=w123:i32)  [unwired: 11 in]
              n32 = call "myRIO_BRig_RT_dataMTrig_Audio_Tcycle__L.vi"() -> ("output_Audio_Tcycle__L"=w124:i32)  [unwired: 11 in]
              n33 = call "myRIO_BRig_RT_dataMTrig_Audio_Tcycle__R.vi"() -> ("output_Audio_Tcycle__R"=w125:i32)  [unwired: 11 in]
              n34 = call "myRIO_BRig_RT_dataMTrig_Laser_Tcycle.vi"() -> ("output_Laser_Tcycle"=w126:i32)  [unwired: 11 in]
              n35 = call "myRIO_BRig_RT_dataMTrig_Solenoid_RewCalib_nCycle__L.vi"() -> ("output_Solenoid_RewCalib_nCycle__L"=w118:i32)  [unwired: 11 in]
              n36 = call "myRIO_BRig_RT_dataMTrig_Solenoid_RewCalib_nCycle__R.vi"() -> ("output_Solenoid_RewCalib_nCycle__R"=w117:i32)  [unwired: 11 in]
              n37 = call "myRIO_BRig_RT_dataMTrig_Solenoid_Tdelay__L.vi"() -> ("output_Solenoid_Tdelay__L"=w116:i32)  [unwired: 11 in]
              n38 = call "myRIO_BRig_RT_dataMTrig_Solenoid_Tdelay__R.vi"() -> ("output_Solenoid_Tdelay__R"=w115:i32)  [unwired: 11 in]
              n39 = local read "MTrig_Solenoid_Tcycle__L"() -> (w127:u16)
              n40 = local read "MTrig_Solenoid_Tcycle__R"() -> (w128:u16)
              n41 = local read "MTrig_Laser_Tcycle"() -> (w111:u16)
              n42 = call "myRIO_BRig_RT_dataMTrig_init.vi"() -> ("output_dataMTrig"=w121:u16[])  [unwired: 5 in]
              n43 = local write "RewCalib_Trig_R"(w114) -> ()
              n44 = local write "RewCalib_Trig_L"(w114) -> ()
              n45 = local read "Tcycle_Cue_min"() -> (w112:u16)
              n46 = Replace Array Subset(array=w121, new element #1=w127, index #1=w122, new element #2=w128, index #2=w123, new element #3=w112, index #3=w124, new element #4=w112, index #4=w125, new element #5=w111, index #5=w126, new element #6=w110, index #6=w118, new element #7=w110, index #7=w117, new element #8=w110, index #8=w116, new element #9=w110, index #9=w115) -> (w120:u16[])
            }
            frame "UploadSettings_pre" {
              # "When the Host sends settings,\nnot all files send at the same time.\n\nIf RT reads the settings faster\nthan the Host can send them,\nthen we will skip settings.\n\nSolution:\nWait 20 cycles"
              n47 = Increment(x=w137) -> (x+1=w136:u16)
              n48 = Greater?(x=w136, y=u16 20) -> (0:w134:bool)
              n49 = Select(t=myRIO_BRig_RT__Case_NonExp_stateList."UploadSettings_Read_dataExp", s=w134, f=w133) -> (s? t:f=w131:T1)
            }
            frame "UploadSettings_Read_dataExp" {
              # "grab dataExp and\nstore it in the\ngeneric data array"
              # "dataExp"
              n50 = call "myRIO_BRig_RT_dataExp_init_details.vi"() -> ("output_dataSize"=w144:i32, "output_dataName"=w147:string)  [unwired: 10 in]
              n51 = call "myRIO_BRig_RT_comm_webdav_uploadReceived_check.vi"("input_dataName"=w147) -> ("output_Iexist"=w146:bool, "output_dataPath"=w145:path)  [unwired: 9 in]
              n52 = case shown="True" w146 {
                tunnel: w145 -> [_ w156]
                tunnel: w144 -> [_ w155]
                tunnel: [_ w154] -> w143
                tunnel: w140 -> [w149 w153]
                tunnel: [w149 w150] -> w139
                frame False {
                }
                frame True {
                  n53 = call "myRIO_BRig_RT_comm_webdav_uploadReceived_read.vi"("input_dataSize"=w155, "input_filePath"=w156) -> ("output_Ivalid"=w154:bool, "output_data"=w152:i64[])  [unwired: 8 in]
                  n54 = To Unsigned Word Integer(number=w152) -> (unsigned 16bit integer=w151:u16[])
                  n55 = Select(t=w151, s=w154, f=w153) -> (s? t:f=w150:u16[])
                }
              }
              n56 = Select(t=myRIO_BRig_RT__Case_NonExp_stateList."UploadSettings_dataExp_1", s=w143, f=myRIO_BRig_RT__Case_NonExp_stateList."UploadSettings_Read_dataLC" ("t")) -> (s? t:f=w138:T1)
            }
            frame "UploadSettings_Read_dataLC" {
              # "grab dataLC and\nstore it in the\ngeneric data array"
              # "dataLC"
              n57 = call "myRIO_BRig_RT_dataLC_init_details.vi"() -> ("output_dataSize"=w163:i32, "output_dataName"=w166:string)  [unwired: 10 in]
              n58 = call "myRIO_BRig_RT_comm_webdav_uploadReceived_check.vi"("input_dataName"=w166) -> ("output_Iexist"=w165:bool, "output_dataPath"=w164:path)  [unwired: 9 in]
              n59 = case shown="True" w165 {
                tunnel: w164 -> [_ w175]
                tunnel: w163 -> [_ w174]
                tunnel: [_ w173] -> w162
                tunnel: w159 -> [w168 w172]
                tunnel: [w168 w169] -> w158
                frame False {
                }
                frame True {
                  n60 = call "myRIO_BRig_RT_comm_webdav_uploadReceived_read.vi"("input_dataSize"=w174, "input_filePath"=w175) -> ("output_Ivalid"=w173:bool, "output_data"=w171:i64[])  [unwired: 8 in]
                  n61 = To Unsigned Word Integer(number=w171) -> (unsigned 16bit integer=w170:u16[])
                  n62 = Select(t=w170, s=w173, f=w172) -> (s? t:f=w169:u16[])
                }
              }
              n63 = Select(t=myRIO_BRig_RT__Case_NonExp_stateList."UploadSettings_dataLC_1", s=w162, f=myRIO_BRig_RT__Case_NonExp_stateList."UploadSettings_Read_dataMTrig" ("t")) -> (s? t:f=w157:T1)
            }
            frame "UploadSettings_Read_dataMTrig" {
              # "grab dataMTrig and\nstore it in the\ngeneric data array"
              # "dataMTrig"
              n64 = call "myRIO_BRig_RT_dataMTrig_init_details.vi"() -> ("output_dataSize"=w182:i32, "output_dataName"=w185:string)  [unwired: 10 in]
              n65 = call "myRIO_BRig_RT_comm_webdav_uploadReceived_check.vi"("input_dataName"=w185) -> ("output_Iexist"=w184:bool, "output_dataPath"=w183:path)  [unwired: 9 in]
              n66 = case shown="True" w184 {
                tunnel: w183 -> [_ w194]
                tunnel: w182 -> [_ w193]
                tunnel: [_ w192] -> w181
                tunnel: w178 -> [w187 w191]
                tunnel: [w187 w188] -> w177
                frame False {
                }
                frame True {
                  n67 = call "myRIO_BRig_RT_comm_webdav_uploadReceived_read.vi"("input_dataSize"=w193, "input_filePath"=w194) -> ("output_Ivalid"=w192:bool, "output_data"=w190:i64[])  [unwired: 8 in]
                  n68 = To Unsigned Word Integer(number=w190) -> (unsigned 16bit integer=w189:u16[])
                  n69 = Select(t=w189, s=w192, f=w191) -> (s? t:f=w188:u16[])
                }
              }
              n70 = Select(t=myRIO_BRig_RT__Case_NonExp_stateList."UploadSettings_dataMTrig_1", s=w181, f=myRIO_BRig_RT__Case_NonExp_stateList."Idle" ("t")) -> (s? t:f=w176:T1)
            }
            frame "UploadSettings_dataExp_1" {
              w203 = 100.0 ("y")
              # "Freq"
              # "f_millisec2count"
              # "laser"
              # "Cue_max"
              # "Cue_min"
              # "CuePenalty"
              # "Timeout"
              # "Wrong"
              # "Selection"
              # "RewardPost"
              # "Reward_R"
              # "Reward_L"
              # "Tcycle"
              # "TPB_min_R"
              # "TPB_min_L"
              # "TPB_max_R"
              # "TPB_max_L"
              # "I_trialUntilReward"
              # "ENL_penalty"
              # "ENL_min"
              # "ENL_max"
              # "BUR_max"
              # "BUR_min"
              # "CueCycles"
              # "Audio_Freq_R"
              # "Audio_Freq_L"
              # "Audio_Amp_R"
              # "Audio_Amp_L"
              n71 = call "myRIO_BRig_RT_dataExp_laser_f_millisec2count.vi"() -> ("output_laser_f_millisec2count"=w217:i32)  [unwired: 11 in]
              n72 = call "myRIO_BRig_RT_dataExp_laser_Freq.vi"() -> ("output_laser_Freq"=w216:i32)  [unwired: 11 in]
              n73 = call "myRIO_BRig_RT_dataExp_CueCycles.vi"() -> ("output_CueCycles"=w263:i32)  [unwired: 11 in]
              n74 = call "myRIO_BRig_RT_dataExp_Audio_amp__R.vi"() -> ("output_Audio_amp__R"=w267:i32)  [unwired: 11 in]
              n75 = call "myRIO_BRig_RT_dataExp_Audio_amp__L.vi"() -> ("output_Audio_amp__L"=w269:i32)  [unwired: 11 in]
              n76 = call "myRIO_BRig_RT_dataExp_Tcycle_Reward__L.vi"() -> ("output_Tcycle_Reward__L"=w240:i32)  [unwired: 11 in]
              n77 = call "myRIO_BRig_RT_dataExp_Tcycle_Reward__R.vi"() -> ("output_Tcycle_Reward__R"=w239:i32)  [unwired: 11 in]
              n78 = call "myRIO_BRig_RT_dataExp_Tcycle_RewardPost.vi"() -> ("output_Tcycle_RewardPost"=w238:i32)  [unwired: 11 in]
              n79 = call "myRIO_BRig_RT_dataExp_BUR_min.vi"() -> ("output_BUR_min"=w260:i32)  [unwired: 11 in]
              n80 = call "myRIO_BRig_RT_dataExp_ENL_min.vi"() -> ("output_ENL_min"=w256:i32)  [unwired: 11 in]
              n81 = call "myRIO_BRig_RT_dataExp_TPB_max__L.vi"() -> ("output_TPB_max__L"=w248:i32)  [unwired: 11 in]
              n82 = call "myRIO_BRig_RT_dataExp_TPB_max__R.vi"() -> ("output_TPB_max__R"=w247:i32)  [unwired: 11 in]
              n83 = call "myRIO_BRig_RT_dataExp_ENL_penalty.vi"() -> ("output_ENL_penalty"=w255:i32)  [unwired: 11 in]
              n84 = call "myRIO_BRig_RT_dataExp_laser_Power_min.vi"() -> ("output_laser_Power_min"=w215:i32)  [unwired: 11 in]
              n85 = call "myRIO_BRig_RT_dataExp_laser_Tpeak.vi"() -> ("output_laser_Tpeak"=w214:i32)  [unwired: 11 in]
              n86 = call "myRIO_BRig_RT_dataExp_Audio_freq__L.vi"() -> ("output_Audio_freq__L"=w265:i32)  [unwired: 11 in]
              n87 = call "myRIO_BRig_RT_dataExp_Audio_freq__R.vi"() -> ("output_Audio_freq__R"=w264:i32)  [unwired: 11 in]
              n88 = call "myRIO_BRig_RT_dataExp_BUR_max.vi"() -> ("output_BUR_max"=w261:i32)  [unwired: 11 in]
              n89 = call "myRIO_BRig_RT_dataExp_ENL_max.vi"() -> ("output_ENL_max"=w257:i32)  [unwired: 11 in]
              n90 = call "myRIO_BRig_RT_dataExp_ItrialUntilReward.vi"() -> ("output_I_trialUntilReward"=w251:i32)  [unwired: 11 in]
              n91 = call "myRIO_BRig_RT_dataExp_Tcycle_Selection.vi"() -> ("output_Tcycle_Selection"=w237:i32)  [unwired: 11 in]
              n92 = call "myRIO_BRig_RT_dataExp_Tcycle_Wrong.vi"() -> ("output_Tcycle_Wrong"=w236:i32)  [unwired: 11 in]
              n93 = call "myRIO_BRig_RT_dataExp_Tcycle_Timeout.vi"() -> ("output_Tcycle_Timeout"=w235:i32)  [unwired: 11 in]
              n94 = call "myRIO_BRig_RT_dataExp_TPB_min__L.vi"() -> ("output_TPB_min__L"=w246:i32)  [unwired: 11 in]
              n95 = call "myRIO_BRig_RT_dataExp_TPB_min__R.vi"() -> ("output_TPB_min__R"=w245:i32)  [unwired: 11 in]
              n96 = call "myRIO_BRig_RT_dataExp_laser_Tshutter.vi"() -> ("output_laser_Tshutter"=w213:i32)  [unwired: 11 in]
              n97 = call "myRIO_BRig_RT_dataExp_laser_duration.vi"() -> ("output_laser_duration"=w212:i32)  [unwired: 11 in]
              n98 = call "myRIO_BRig_RT_dataExp_Tcycle_CuePenalty.vi"() -> ("output_Tcycle_CuePenalty"=w228:i32)  [unwired: 11 in]
              n99 = call "myRIO_BRig_RT_dataExp_Tcycle_Cue_min.vi"() -> ("output_Tcycle_Cue_min"=w227:i32)  [unwired: 11 in]
              n100 = call "myRIO_BRig_RT_dataExp_Tcycle_Cue_max.vi"() -> ("output_Tcycle_Cue_max"=w226:i32)  [unwired: 11 in]
              n101 = Index Array(array=w220, index #1=w269, index #2=w267, index #3=w265, index #4=w264, index #5=w263, index #6=w261, index #7=w260, index #8=w257, index #9=w256, index #10=w255, index #11=w251, index #12=w248, index #13=w247, index #14=w246, index #15=w245, index #16=w240, index #17=w239, index #18=w238, index #19=w237, index #20=w236, index #21=w235, index #22=w228, index #23=w227, index #24=w226, index #25=w217, index #26=w216, index #27=w215, index #28=w214, index #29=w213, index #30=w212) -> (element #1=w268:u16, element #2=w266:u16, element #3=w223:u16, element #4=w222:u16, element #5=w262:u16, element #6=w259:u16, element #7=w258:u16, element #8=w254:u16, element #9=w253:u16, element #10=w252:u16, element #11=w249:u16, element #12=w244:u16, element #13=w243:u16, element #14=w242:u16, element #15=w241:u16, element #16=w234:u16, element #17=w233:u16, element #18=w232:u16, element #19=w231:u16, element #20=w230:u16, element #21=w229:u16, element #22=w225:u16, element #23=w219:u16, element #24=w218:u16, element #25=w211:u16, element #26=w202:u16, element #27=w201:u16, element #28=w200:u16, element #29=w199:u16, element #30=w195:u16)
              n102 = To Double Precision Float(number=w211) -> (double precision float=w210:dbl)
              n103 = To Double Precision Float(number=w202) -> (double precision float=w208:dbl)
              n104 = To Double Precision Float(number=w201) -> (double precision float=w206:dbl)
              n105 = To Double Precision Float(number=w200) -> (double precision float=w205:dbl)
              n106 = To Double Precision Float(number=w199) -> (double precision float=w204:dbl)
              n107 = local write "Tcycle_Selection"(w231) -> ()
              n108 = local write "Tcycle_Wrong"(w230) -> ()
              n109 = local write "Tcycle_Timeout"(w229) -> ()
              n110 = local write "Audio_Amp__L"(w268) -> ()
              n111 = local write "Audio_Amp__R"(w266) -> ()
              n112 = Divide(x=w210, y=w203) -> (x/y=w209:dbl)
              n113 = Divide(x=w208, y=w203) -> (x/y=w207:dbl)
              n114 = Divide(x=w206, y=w203) -> (x/y=w198:dbl)
              n115 = Divide(x=w205, y=w203) -> (x/y=w197:dbl)
              n116 = Divide(x=w204, y=w203) -> (x/y=w196:dbl)
              n117 = local write "Tcycle_ENLPenalty"(w252) -> ()
              n118 = local write "Tcycle_ENL_max"(w254) -> ()
              n119 = local write "laser_duration"(w195) -> ()
              n120 = local write "TpB_Min_L"(w242) -> ()
              n121 = local write "TpB_Min_R"(w241) -> ()
              n122 = local write "laser_power_min"(w198) -> ()
              n123 = local write "f_millisec2count"(w209) -> ()
              n124 = local write "laser_Tshutter"(w196) -> ()
              n125 = local write "laser_Tpeak"(w197) -> ()
              n126 = local write "laser_Freq"(w207) -> ()
              n127 = local write "Tcycle_CuePenalty"(w225) -> ()
              n128 = local write "Tcycle_Cue_min"(w219) -> ()
              n129 = local write "Tcycle_Cue_max"(w218) -> ()
              n130 = To Unsigned Byte Integer(number=w223) -> (unsigned 8bit integer=w224:u8)
              n131 = To Unsigned Byte Integer(number=w222) -> (unsigned 8bit integer=w221:u8)
              n132 = Not Equal To 0?(x=w249) -> (x != 0?=w250:bool)
              n133 = local write "Tcycle_Reward_L"(w234) -> ()
              n134 = local write "Tcycle_Reward_R"(w233) -> ()
              n135 = local write "Tcycle_RewardPost"(w232) -> ()
              n136 = local write "CueCycles"(w262) -> ()
              n137 = local write "BUR_min"(w258) -> ()
              n138 = local write "BUR_max"(w259) -> ()
              n139 = local write "Tcycle_ENL_min"(w253) -> ()
              n140 = local write "TpB_Max_L"(w244) -> ()
              n141 = local write "TpB_Max_R"(w243) -> ()
              n142 = local write "TrialUntilReward"(w250) -> ()
              n143 = local write "Audio_Freq__L"(w224) -> ()
              n144 = local write "Audio_Freq__R"(w221) -> ()
            }
            frame "UploadSettings_dataLC_1" {
              # "Cue1_All_delayOpt"
              # "ENL1_All_delayOpt"
              # "Cue1_First_delayOpt"
              # "ENL1_First_delayOpt"
              # "ENL1 First"
              # "Cue1 All"
              # "Cue1 First"
              # "Count"
              # "Tdelay"
              # "Prob"
              # "OnOff"
              # "Block"
              # "ENL1 All"
              # "Count"
              # "Tdelay"
              # "Prob"
              # "OnOff"
              # "Block"
              # "Count"
              # "Tdelay"
              # "Prob"
              # "Block"
              # "OnOff"
              # "Count"
              # "Tdelay"
              # "Prob"
              # "OnOff"
              # "Block"
              n145 = call "myRIO_BRig_RT_dataLC_Cue1_First_Block.vi"() -> ("output_Cue1_First_Block"=w328:i32)  [unwired: 11 in]
              n146 = call "myRIO_BRig_RT_dataLC_Cue1_First_OnOff.vi"() -> ("output_Cue1_First_OnOff"=w326:i32)  [unwired: 11 in]
              n147 = call "myRIO_BRig_RT_dataLC_Cue1_First_Count.vi"() -> ("output_Cue1_First_Count"=w323:i32)  [unwired: 11 in]
              n148 = call "myRIO_BRig_RT_dataLC_Cue1_All_Block.vi"() -> ("output_Cue1_All_Block"=w310:i32)  [unwired: 11 in]
              n149 = call "myRIO_BRig_RT_dataLC_Cue1_All_OnOff.vi"() -> ("output_Cue1_All_OnOff"=w309:i32)  [unwired: 11 in]
              n150 = call "myRIO_BRig_RT_dataLC_Cue1_All_Count.vi"() -> ("output_Cue1_All_Count"=w320:i32)  [unwired: 11 in]
              n151 = call "myRIO_BRig_RT_dataLC_ENL1_First_Block.vi"() -> ("output_ENL1_First_Block"=w308:i32)  [unwired: 11 in]
              n152 = call "myRIO_BRig_RT_dataLC_ENL1_First_OnOff.vi"() -> ("output_ENL1_First_OnOff"=w319:i32)  [unwired: 11 in]
              n153 = call "myRIO_BRig_RT_dataLC_ENL1_First_Count.vi"() -> ("output_ENL1_First_Count"=w316:i32)  [unwired: 11 in]
              n154 = call "myRIO_BRig_RT_dataLC_ENL1_All_Block.vi"() -> ("output_ENL1_All_Block"=w315:i32)  [unwired: 11 in]
              n155 = call "myRIO_BRig_RT_dataLC_ENL1_All_OnOff.vi"() -> ("output_ENL1_All_OnOff"=w314:i32)  [unwired: 11 in]
              n156 = call "myRIO_BRig_RT_dataLC_ENL1_All_Count.vi"() -> ("output_ENL1_All_Count"=w311:i32)  [unwired: 11 in]
              n157 = call "myRIO_BRig_RT_dataLC_ENL1_First_delayOpt.vi"() -> ("output_ENL1_First_delayOpt"=w285:i32)  [unwired: 11 in]
              n158 = call "myRIO_BRig_RT_dataLC_Cue1_First_delayOpt.vi"() -> ("output_Cue1_First_delayOpt"=w284:i32)  [unwired: 11 in]
              n159 = call "myRIO_BRig_RT_dataLC_ENL1_All_delayOpt.vi"() -> ("output_ENL1_All_delayOpt"=w277:i32)  [unwired: 11 in]
              n160 = call "myRIO_BRig_RT_dataLC_Cue1_All_delayOpt.vi"() -> ("output_Cue1_All_delayOpt"=w276:i32)  [unwired: 11 in]
              n161 = call "myRIO_BRig_RT_dataLC_Cue1_First_Probability.vi"() -> ("output_Cue1_First_Probability"=w325:i32)  [unwired: 11 in]
              n162 = call "myRIO_BRig_RT_dataLC_Cue1_First_Tdelay.vi"() -> ("output_Cue1_First_Tdelay"=w324:i32)  [unwired: 11 in]
              n163 = call "myRIO_BRig_RT_dataLC_Cue1_All_Probability.vi"() -> ("output_Cue1_All_Probability"=w322:i32)  [unwired: 11 in]
              n164 = call "myRIO_BRig_RT_dataLC_Cue1_All_Tdelay.vi"() -> ("output_Cue1_All_Tdelay"=w321:i32)  [unwired: 11 in]
              n165 = call "myRIO_BRig_RT_dataLC_ENL1_First_Probability.vi"() -> ("output_ENL1_First_Probability"=w318:i32)  [unwired: 11 in]
              n166 = call "myRIO_BRig_RT_dataLC_ENL1_First_Tdelay.vi"() -> ("output_ENL1_First_Tdelay"=w317:i32)  [unwired: 11 in]
              n167 = call "myRIO_BRig_RT_dataLC_ENL1_All_Probability.vi"() -> ("output_ENL1_All_Probability"=w313:i32)  [unwired: 11 in]
              n168 = call "myRIO_BRig_RT_dataLC_ENL1_All_Tdelay.vi"() -> ("output_ENL1_All_Tdelay"=w312:i32)  [unwired: 11 in]
              n169 = Index Array(array=w286, index #1=w328, index #2=w326, index #3=w325, index #4=w324, index #5=w323, index #6=w310, index #7=w309, index #8=w322, index #9=w321, index #10=w320, index #11=w308, index #12=w319, index #13=w318, index #14=w317, index #15=w316, index #16=w315, index #17=w314, index #18=w313, index #19=w312, index #20=w311, index #21=w285, index #22=w284, index #23=w277, index #24=w276) -> (element #1=w327:u16, element #2=w306:u16, element #3=w305:u16, element #4=w304:u16, element #5=w303:u16, element #6=w299:u16, element #7=w298:u16, element #8=w297:u16, element #9=w296:u16, element #10=w295:u16, element #11=w294:u16, element #12=w293:u16, element #13=w292:u16, element #14=w291:u16, element #15=w278:u16, element #16=w290:u16, element #17=w289:u16, element #18=w288:u16, element #19=w287:u16, element #20=w279:u16, element #21=w282:u16, element #22=w280:u16, element #23=w273:u16, element #24=w272:u16)
              n170 = Not Equal To 0?(x=w273) -> (x != 0?=w275:bool)
              n171 = Not Equal To 0?(x=w272) -> (x != 0?=w274:bool)
              n172 = Not Equal To 0?(x=w282) -> (x != 0?=w283:bool)
              n173 = Not Equal To 0?(x=w280) -> (x != 0?=w281:bool)
              n174 = Not Equal To 0?(x=w306) -> (x != 0?=w307:bool)
              n175 = Not Equal To 0?(x=w298) -> (x != 0?=w302:bool)
              n176 = Not Equal To 0?(x=w293) -> (x != 0?=w301:bool)
              n177 = Not Equal To 0?(x=w289) -> (x != 0?=w300:bool)
              n178 = local write "LC_Cue1_First_Probability"(w305) -> ()
              n179 = local write "LC_ENL1_First_Probability"(w292) -> ()
              n180 = local write "LC_ENL1_First_delayOpt"(w283) -> ()
              n181 = local write "LC_Cue1_First_delayOpt"(w281) -> ()
              n182 = local write "LC_ENL1_All_delayOpt"(w275) -> ()
              n183 = local write "LC_Cue1_All_delayOpt"(w274) -> ()
              n184 = local write "LC_Cue1_All_Probability"(w297) -> ()
              n185 = local write "LC_Cue1_First_Tdelay"(w304) -> ()
              n186 = local write "LC_ENL1_All_Probability"(w288) -> ()
              n187 = local write "LC_Cue1_First_OnOff"(w307) -> ()
              n188 = local write "LC_Cue1_First_Count"(w303) -> ()
              n189 = local write "LC_Cue1_First_Block"(w327) -> ()
              n190 = local write "LC_ENL1_First_Tdelay"(w291) -> ()
              n191 = local write "LC_ENL1_First_OnOff"(w301) -> ()
              n192 = local write "LC_ENL1_First_Count"(w278) -> ()
              n193 = local write "LC_ENL1_First_Block"(w294) -> ()
              n194 = local write "LC_Cue1_All_Tdelay"(w296) -> ()
              n195 = local write "LC_Cue1_All_OnOff"(w302) -> ()
              n196 = local write "LC_Cue1_All_Count"(w295) -> ()
              n197 = local write "LC_Cue1_All_Block"(w299) -> ()
              n198 = local write "LC_ENL1_All_Tdelay"(w287) -> ()
              n199 = local write "LC_ENL1_All_OnOff"(w300) -> ()
              n200 = local write "LC_ENL1_All_Count"(w279) -> ()
              n201 = local write "LC_ENL1_All_Block"(w290) -> ()
            }
            frame "UploadSettings_dataLC_2" {
              # "Wrong"
              # "Reward"
              # "Trial"
              # "Tdelay"
              # "Prob"
              # "Block"
              # "OnOff"
              # "Trial"
              # "Tdelay"
              # "Prob"
              # "OnOff"
              # "Block"
              n202 = call "myRIO_BRig_RT_dataLC_Reward_Block.vi"() -> ("output_Reward_Block"=w353:i32)  [unwired: 11 in]
              n203 = call "myRIO_BRig_RT_dataLC_Reward_OnOff.vi"() -> ("output_Reward_OnOff"=w351:i32)  [unwired: 11 in]
              n204 = call "myRIO_BRig_RT_dataLC_Reward_Trial.vi"() -> ("output_Reward_Trial"=w348:i32)  [unwired: 11 in]
              n205 = call "myRIO_BRig_RT_dataLC_Wrong_Block.vi"() -> ("output_Wrong_Block"=w344:i32)  [unwired: 11 in]
              n206 = call "myRIO_BRig_RT_dataLC_Wrong_OnOff.vi"() -> ("output_Wrong_OnOff"=w343:i32)  [unwired: 11 in]
              n207 = call "myRIO_BRig_RT_dataLC_Wrong_Trial.vi"() -> ("output_Wrong_Trial"=w345:i32)  [unwired: 11 in]
              n208 = call "myRIO_BRig_RT_dataLC_Reward_Probability.vi"() -> ("output_Reward_Probability"=w350:i32)  [unwired: 11 in]
              n209 = call "myRIO_BRig_RT_dataLC_Reward_Tdelay.vi"() -> ("output_Reward_Tdelay"=w349:i32)  [unwired: 11 in]
              n210 = call "myRIO_BRig_RT_dataLC_Wrong_Probability.vi"() -> ("output_Wrong_Probability"=w347:i32)  [unwired: 11 in]
              n211 = call "myRIO_BRig_RT_dataLC_Wrong_Tdelay.vi"() -> ("output_Wrong_Tdelay"=w346:i32)  [unwired: 11 in]
              n212 = Index Array(array=w331, index #1=w353, index #2=w351, index #3=w350, index #4=w349, index #5=w348, index #6=w344, index #7=w343, index #8=w347, index #9=w346, index #10=w345) -> (element #1=w352:u16, element #2=w341:u16, element #3=w340:u16, element #4=w339:u16, element #5=w338:u16, element #6=w336:u16, element #7=w335:u16, element #8=w334:u16, element #9=w333:u16, element #10=w332:u16)
              n213 = Not Equal To 0?(x=w341) -> (x != 0?=w342:bool)
              n214 = Not Equal To 0?(x=w335) -> (x != 0?=w337:bool)
              n215 = local write "LC_Reward_Probability"(w340) -> ()
              n216 = local write "LC_Wrong_Probability"(w334) -> ()
              n217 = local write "LC_Reward_Tdelay"(w339) -> ()
              n218 = local write "LC_Reward_OnOff"(w342) -> ()
              n219 = local write "LC_Reward_Block"(w352) -> ()
              n220 = local write "LC_Reward_Trial"(w338) -> ()
              n221 = local write "LC_Wrong_Tdelay"(w333) -> ()
              n222 = local write "LC_Wrong_OnOff"(w337) -> ()
              n223 = local write "LC_Wrong_Block"(w336) -> ()
              n224 = local write "LC_Wrong_Trial"(w332) -> ()
            }
            frame "UploadSettings_dataMTrig_1" {
              # "Tdelay_R"
              # "Tdelay_L"
              # "Tcycle_R"
              # "Tcycle_L"
              # "RewCalib_nCycle_R"
              # "RewCalib_nCycle_L"
              # "Solenoid"
              # "Laser_Tcycle"
              n225 = call "myRIO_BRig_RT_dataMTrig_Laser_Tcycle.vi"() -> ("output_Laser_Tcycle"=w363:i32)  [unwired: 11 in]
              n226 = call "myRIO_BRig_RT_dataMTrig_Solenoid_RewCalib_nCycle__L.vi"() -> ("output_Solenoid_RewCalib_nCycle__L"=w362:i32)  [unwired: 11 in]
              n227 = call "myRIO_BRig_RT_dataMTrig_Solenoid_RewCalib_nCycle__R.vi"() -> ("output_Solenoid_RewCalib_nCycle__R"=w361:i32)  [unwired: 11 in]
              n228 = call "myRIO_BRig_RT_dataMTrig_Solenoid_Tdelay__L.vi"() -> ("output_Solenoid_Tdelay__L"=w358:i32)  [unwired: 11 in]
              n229 = call "myRIO_BRig_RT_dataMTrig_Solenoid_Tdelay__R.vi"() -> ("output_Solenoid_Tdelay__R"=w357:i32)  [unwired: 11 in]
              n230 = call "myRIO_BRig_RT_dataMTrig_Solenoid_Tcycle__L.vi"() -> ("output_Solenoid_Tcycle__L"=w360:i32)  [unwired: 11 in]
              n231 = call "myRIO_BRig_RT_dataMTrig_Solenoid_Tcycle__R.vi"() -> ("output_Solenoid_Tcycle__R"=w359:i32)  [unwired: 11 in]
              n232 = Index Array(array=w356, index #1=w363, index #2=w362, index #3=w361, index #4=w360, index #5=w359, index #6=w358, index #7=w357) -> (element #1=w370:u16, element #2=w369:u16, element #3=w368:u16, element #4=w367:u16, element #5=w366:u16, element #6=w365:u16, element #7=w364:u16)
              n233 = Replace Array Subset(array=w372, new element #1=w370, index #1=w363, new element #2=w369, index #2=w362, new element #3=w368, index #3=w361, new element #4=w367, index #4=w360, new element #5=w366, index #5=w359, new element #6=w365, index #6=w358, new element #7=w364, index #7=w357) -> (w371:u16[])
              n234 = local write "MTrig_Solenoid_Tcycle__L"(w367) -> ()
              n235 = local write "MTrig_Solenoid_Tcycle__R"(w366) -> ()
              n236 = local write "MTrig_Laser_Tcycle"(w370) -> ()
            }
            frame "Idle" {
              # "To ensure timing, we split the\nidle state into 4 phases"
              # "Laser_Tcycle"
              # "Audio_Tcycle_R"
              # "Audio_Tcycle_L"
              n237 = local read "laser_power_min"() -> (w375:dbl)
              n238 = local read "f_millisec2count"() -> (w383:dbl)
              n239 = local read "Audio_Amp__R"() -> (w377:u16)
              n240 = local read "Audio_Amp__L"() -> (w379:u16)
              n241 = local read "Audio_Freq__R"() -> (w376:u8)
              n242 = local read "Audio_Freq__L"() -> (w378:u8)
              n243 = local read "MTrig_Audio_trig__L"() -> (w391:bool)
              n244 = local read "MTrig_Audio_trig__R"() -> (w393:bool)
              n245 = Select(t=myRIO_BRig_RT__Case_NonExp_stateList."SendData" ("Enum"), s="SendData", f=myRIO_BRig_RT__Case_NonExp_stateList."Idle_2" ("Enum")) -> (s? t:f=w386:T1)
              n246 = call "myRIO__convert__Voltage_to_FPGAvalue.vi"("input_voltage"=w375) -> ("output_PortA"=w374:u16)  [unwired: 9 in, 1 out]
              n247 = local read "MTrig_Laser_trig"() -> (w392:bool)
              n248 = To Unsigned Word Integer(number=w383) -> (unsigned 16bit integer=w382:u16)
              n249 = call "myRIO_BRig_RT_dataMTrig_Audio_Tcycle__L.vi"() -> ("output_Audio_Tcycle__L"=w402:i32)  [unwired: 11 in]
              n250 = call "myRIO_BRig_RT_dataMTrig_Audio_Tcycle__R.vi"() -> ("output_Audio_Tcycle__R"=w401:i32)  [unwired: 11 in]
              n251 = call "myRIO_BRig_RT_dataMTrig_Laser_Tcycle.vi"() -> ("output_Laser_Tcycle"=w400:i32)  [unwired: 11 in]
              n252 = local read "MTrig_Laser_Tcycle"() -> (w384:u16)
              n253 = xnode "Read/Write Control"("FPGA VI Reference In"=w381, "error in"=w380, "k1__counter_per_ms"=w382, "audioAmp_L"=w379, "audioFreq_L_kHz"=w378, "audioAmp_R"=w377, "audioFreq_R_kHz"=w376, "AnaOut_0"=w374) -> ()  [unwired: 2 out]
              n254 = Select(t=myRIO_BRig_RT__Case_NonExp_stateList."TestConnection" ("Enum"), s="TestConnection", f=w386) -> (s? t:f=w395:T1)
              n255 = local read "Tcycle_Cue_min"() -> (w385:u16)
              n256 = Compound Arithmetic op=OR(w391, w393, w392) -> (w394:bool)
              n257 = case shown="True" w394 {
                frame False {
                }
                frame True {
                  w403 = FALSE
                  n258 = local write "MTrig_Audio_trig__L"(w403) -> ()
                  n259 = local write "MTrig_Audio_trig__R"(w403) -> ()
                  n260 = local write "MTrig_Laser_trig"(w403) -> ()
                }
              }
              n261 = Replace Array Subset(array=w398, new element #1=w385, index #1=w402, new element #2=w385, index #2=w401, new element #3=w384, index #3=w400) -> (w399:u16[])
            }
            frame "Idle_2" {
              w405 = u16 0 ("t")
              # "To ensure timing, we split the\nidle state into 4 phases"
              # "Ncycles"
              # "Ncycles"
              # "RewCalib"
              # "RewCalib"
              # "Solenoid R"
              # "Solenoid L"
              n262 = call "myRIO_BRig_RT_dataMTrig_Solenoid_RewCalib_OnOff__L.vi"() -> ("output_Solenoid_RewCalib_OnOff__L"=w436:i32)  [unwired: 11 in]
              n263 = call "myRIO_BRig_RT_dataMTrig_Solenoid_N__L.vi"() -> ("output_Solenoid_N__L"=w424:i32)  [unwired: 11 in]
              n264 = call "myRIO_BRig_RT_dataMTrig_Solenoid_RewCalib_OnOff__R.vi"() -> ("output_Solenoid_RewCalib_OnOff__R"=w421:i32)  [unwired: 11 in]
              n265 = call "myRIO_BRig_RT_dataMTrig_Solenoid_N__R.vi"() -> ("output_Solenoid_N__R"=w420:i32)  [unwired: 11 in]
              n266 = Index Array(array=w427, index #1=w436, index #2=w424, index #3=w421, index #4=w420) -> (element #1=w423:u16, element #2=w418:u16, element #3=w419:u16, element #4=w417:u16)
              n267 = local read "RewCalib_Trig_L"() -> (w416:bool)
              n268 = local read "RewCalib_Trig_R"() -> (w415:bool)
              n269 = Equal To 0?(x=w418) -> (x = 0?=w426:bool)
              n270 = Equal To 0?(x=w417) -> (x = 0?=w425:bool)
              n271 = Not Equal To 0?(x=w419) -> (x != 0?=w437:bool)
              n272 = Not Equal To 0?(x=w423) -> (x != 0?=w438:bool)
              n273 = And(x=w426, y=w425) -> (x .and. y?=w430:bool)
              n274 = Or(x=w416, y=w415) -> (x .or. y?=w431:bool)
              n275 = Not Exclusive Or(1:w438, 2:w416) -> (0:w433:bool)
              n276 = Not Exclusive Or(1:w437, 2:w415) -> (0:w435:bool)
              n277 = And(x=w431, y=w430) -> (x .and. y?=w413:bool)
              n278 = Not(x=w433) -> (.not. x?=w432:bool)
              n279 = Not(x=w435) -> (.not. x?=w434:bool)
              n280 = Or(x=w432, y=w434) -> (x .or. y?=w414:bool)
              n281 = Or(x=w413, y=w414) -> (x .or. y?=w429:bool)
              n282 = local read "count_warmup_R"() -> (w404:u16)
              n283 = local read "count_warmup_L"() -> (w409:u16)
              n284 = Select(t=myRIO_BRig_RT__Case_NonExp_stateList."RewardCalibration_pre" ("Enum"), s=w429, f=myRIO_BRig_RT__Case_NonExp_stateList."Idle_3" ("Enum")) -> (s? t:f=w412:T1)
              n285 = Select(t=w405, s="count_warmup_L_reset", f=w409) -> (s? t:f=→"count_warmup_L":u16)
              n286 = Select(t=w405, s="count_warmup_R_reset", f=w404) -> (s? t:f=→"count_warmup_R":u16)
            }
            frame "Idle_3" {
              w461 = u8 0 ("f")
              # "To ensure timing, we split the\nidle state into 4 phases"
              n287 = local read "MTrig_Solenoid_trig__L"() -> (w452:bool)
              n288 = local read "MTrig_Solenoid_trig__R"() -> (w462:bool)
              n289 = local read "warmupType"() -> (w444:u8)
              n290 = local read "warmup"() -> (w454:bool)
              n291 = Not Equal To 0?(x=w444) -> (x != 0?=w443:bool)
              n292 = Not(x=w443) -> (.not. x?=w455:bool)
              n293 = Select(t=u8 1, s=w452, f=w461) -> (s? t:f=w460:u8)
              n294 = Select(t=u8 2, s=w462, f=w461) -> (s? t:f=w459:u8)
              n295 = And(x=w454, y=w455) -> (x .and. y?=w453:bool)
              n296 = And(x=w454, y=w443) -> (x .and. y?=w448:bool)
              n297 = Add(x=w460, y=w459) -> (x+y=w458:u8)
              n298 = case shown="3" w458 {
                tunnel: w457 -> [w465 w469 w487 w505]
                tunnel: [w465 w468 w486 w504] -> w456
                tunnel: w453 -> [_ w467 w485 w503]
                tunnel: [_ TRUE TRUE TRUE] -> w450
                frame 0, Default {
                }
                frame 1 {
                  n299 = case shown="True" w467 {
                    tunnel: w469 -> [w478 w483]
                    tunnel: [w477 w482] -> w468
                    frame True {
                      # "Audio_L"
                      # "Solenoid_L"
                      n300 = call "myRIO_BRig_RT_dataMTrig_Solenoid_N__L.vi"() -> ("output_Solenoid_N__L"=w474:i32)  [unwired: 11 in]
                      n301 = call "myRIO_BRig_RT_dataMTrig_Audio_N__L.vi"() -> ("output_Audio_N__L"=w472:i32)  [unwired: 11 in]
                      n302 = Index Array(array=w478, index #1=w474, index #2=w472) -> (element #1=w476:u16, element #2=w475:u16)
                      n303 = Increment(x=w476) -> (x+1=w473:u16)
                      n304 = Increment(x=w475) -> (x+1=w471:u16)
                      n305 = Replace Array Subset(array=w478, new element #1=w473, index #1=w474, new element #2=w471, index #2=w472) -> (w477:u16[])
                    }
                    frame False {
                      # "Solenoid_L"
                      n306 = call "myRIO_BRig_RT_dataMTrig_Solenoid_N__L.vi"() -> ("output_Solenoid_N__L"=w480:i32)  [unwired: 11 in]
                      n307 = Index Array(array=w483, index=w480) -> (element=w481:u16)
                      n308 = Increment(x=w481) -> (x+1=w479:u16)
                      n309 = Replace Array Subset(array=w483, new element=w479, index=w480) -> (w482:u16[])
                    }
                  }
                  n310 = local write "MTrig_Solenoid_trig__L"(FALSE) -> ()
                }
                frame 2 {
                  n311 = case shown="True" w485 {
                    tunnel: w487 -> [w496 w501]
                    tunnel: [w495 w500] -> w486
                    frame True {
                      # "Audio_R"
                      # "Solenoid_R"
                      n312 = call "myRIO_BRig_RT_dataMTrig_Solenoid_N__R.vi"() -> ("output_Solenoid_N__R"=w492:i32)  [unwired: 11 in]
                      n313 = call "myRIO_BRig_RT_dataMTrig_Audio_N__R.vi"() -> ("output_Audio_N__R"=w491:i32)  [unwired: 11 in]
                      n314 = Index Array(array=w496, index #1=w492, index #2=w491) -> (element #1=w494:u16, element #2=w493:u16)
                      n315 = Increment(x=w493) -> (x+1=w489:u16)
                      n316 = Increment(x=w494) -> (x+1=w490:u16)
                      n317 = Replace Array Subset(array=w496, new element #1=w490, index #1=w492, new element #2=w489, index #2=w491) -> (w495:u16[])
                    }
                    frame False {
                      # "Solenoid_R"
                      n318 = call "myRIO_BRig_RT_dataMTrig_Solenoid_N__R.vi"() -> ("output_Solenoid_N__R"=w497:i32)  [unwired: 11 in]
                      n319 = Index Array(array=w501, index=w497) -> (element=w499:u16)
                      n320 = Increment(x=w499) -> (x+1=w498:u16)
                      n321 = Replace Array Subset(array=w501, new element=w498, index=w497) -> (w500:u16[])
                    }
                  }
                  n322 = local write "MTrig_Solenoid_trig__R"(FALSE) -> ()
                }
                frame 3 {
                  w506 = FALSE
                  n323 = case shown="True" w503 {
                    tunnel: w505 -> [w520 w528]
                    tunnel: [w519 w527] -> w504
                    frame True {
                      # "Audio_R"
                      # "Solenoid_R"
                      # "Audio_L"
                      # "Solenoid_L"
                      n324 = call "myRIO_BRig_RT_dataMTrig_Solenoid_N__L.vi"() -> ("output_Solenoid_N__L"=w514:i32)  [unwired: 11 in]
                      n325 = call "myRIO_BRig_RT_dataMTrig_Audio_N__L.vi"() -> ("output_Audio_N__L"=w512:i32)  [unwired: 11 in]
                      n326 = call "myRIO_BRig_RT_dataMTrig_Solenoid_N__R.vi"() -> ("output_Solenoid_N__R"=w510:i32)  [unwired: 11 in]
                      n327 = call "myRIO_BRig_RT_dataMTrig_Audio_N__R.vi"() -> ("output_Audio_N__R"=w509:i32)  [unwired: 11 in]
                      n328 = Index Array(array=w520, index #1=w514, index #2=w512, index #3=w510, index #4=w509) -> (element #1=w518:u16, element #2=w517:u16, element #3=w516:u16, element #4=w515:u16)
                      n329 = Increment(x=w515) -> (x+1=w507:u16)
                      n330 = Increment(x=w518) -> (x+1=w513:u16)
                      n331 = Increment(x=w517) -> (x+1=w511:u16)
                      n332 = Increment(x=w516) -> (x+1=w508:u16)
                      n333 = Replace Array Subset(array=w520, new element #1=w513, index #1=w514, new element #2=w511, index #2=w512, new element #3=w508, index #3=w510, new element #4=w507, index #4=w509) -> (w519:u16[])
                    }
                    frame False {
                      # "Solenoid_R"
                      # "Solenoid_L"
                      n334 = call "myRIO_BRig_RT_dataMTrig_Solenoid_N__L.vi"() -> ("output_Solenoid_N__L"=w524:i32)  [unwired: 11 in]
                      n335 = call "myRIO_BRig_RT_dataMTrig_Solenoid_N__R.vi"() -> ("output_Solenoid_N__R"=w521:i32)  [unwired: 11 in]
                      n336 = Index Array(array=w528, index #1=w524, index #2=w521) -> (element #1=w526:u16, element #2=w525:u16)
                      n337 = Increment(x=w526) -> (x+1=w523:u16)
                      n338 = Increment(x=w525) -> (x+1=w522:u16)
                      n339 = Replace Array Subset(array=w528, new element #1=w523, index #1=w524, new element #2=w522, index #2=w521) -> (w527:u16[])
                    }
                  }
                  n340 = local write "MTrig_Solenoid_trig__L"(w506) -> ()
                  n341 = local write "MTrig_Solenoid_trig__R"(w506) -> ()
                }
              }
              n342 = local read "get_countPerMS"() -> (w442:bool)
              n343 = Select(t=myRIO_BRig_RT__Case_NonExp_stateList."Get_FPGA_count_per_ms" ("Enum"), s=w442, f=myRIO_BRig_RT__Case_NonExp_stateList."Idle_4" ("Enum")) -> (s? t:f=w440:T1)
              n344 = Select(t=myRIO_BRig_RT__Case_NonExp_stateList."Cue_pre", s=w448, f=myRIO_BRig_RT__Case_NonExp_stateList."DispenseWater_pre" ("Enum")) -> (s? t:f=w446:T1)
              n345 = Select(t=w446, s=w450, f=w440) -> (s? t:f=w451:T1)
            }
            frame "Idle_4" {
              # "use dataMTrig as it is one of the last to transfer"
              # "To ensure timing, we split the\nidle state into 4 phases"
              n346 = call "myRIO_BRig_RT_comm_webdav_uploadReceived_check_v2,0.vi"("input_dataName"="dataMTrig") -> ("output_Iexist"=w534:bool)  [unwired: 9 in, 1 out]
              n347 = Select(t=myRIO_BRig_RT__Case_NonExp_stateList."UploadSettings_pre" ("Enum"), s=w534, f=myRIO_BRig_RT__Case_NonExp_stateList."Idle") -> (s? t:f=w532:T1)
            }
            frame "Cue_pre" {
              w544 = u16 1 ("t")
              w543 = u16 0 ("new element/subarray")
              w540 = u16 0 ("new element/subarray")
              # "Ncycle"
              # "count"
              # "Audio_R"
              # "Solenoid_R"
              # "Solenoid_L"
              # "Ncycle"
              # "count"
              # "Audio_L"
              n348 = call "myRIO_BRig_RT_dataMTrig_Solenoid_N__L.vi"() -> ("output_Solenoid_N__L"=w553:i32)  [unwired: 11 in]
              n349 = call "myRIO_BRig_RT_dataMTrig_Solenoid_N__R.vi"() -> ("output_Solenoid_N__R"=w552:i32)  [unwired: 11 in]
              n350 = Index Array(array=w549, index #1=w553, index #2=w552) -> (element #1=w551:u16, element #2=w550:u16)
              n351 = Not Equal To 0?(x=w550) -> (x != 0?=w536:bool)
              n352 = Not Equal To 0?(x=w551) -> (x != 0?=w537:bool)
              n353 = Select(t=w544, s=w537, f=w543) -> (s? t:f=w545:u16)
              n354 = Select(t=w544, s=w536, f=w543) -> (s? t:f=w539:u16)
              n355 = call "myRIO_BRig_RT_dataMTrig_Audio_c__L.vi"() -> ("output_Audio_c__L"=w547:i32)  [unwired: 11 in]
              n356 = call "myRIO_BRig_RT_dataMTrig_Audio_N__L.vi"() -> ("output_Audio_N__L"=w546:i32)  [unwired: 11 in]
              n357 = call "myRIO_BRig_RT_dataMTrig_Audio_c__R.vi"() -> ("output_Audio_c__R"=w542:i32)  [unwired: 11 in]
              n358 = call "myRIO_BRig_RT_dataMTrig_Audio_N__R.vi"() -> ("output_Audio_N__R"=w541:i32)  [unwired: 11 in]
              n359 = Replace Array Subset(array=w549, new element #1=w540, index #1=w547, new element #2=w545, index #2=w546, new element #3=w540, index #3=w542, new element #4=w539, index #4=w541) -> (w548:u16[])
            }
            frame "Cue" {
              # "lick did not occur or warmupType==1"
              # "lick occurred?"
              # "Ncycle"
              # "Audio_R"
              # "Ncycle"
              # "Audio_L"
              n360 = local read "warmupType"() -> (w563:u8)
              n361 = Greater?(x=w569, y=w568) -> (0:w572:bool)
              n362 = Greater?(x=w571, y=w570) -> (0:w567:bool)
              n363 = Or(x=w567, y=w572) -> (x .or. y?=w561:bool)
              n364 = Equal?(x=w563, y=u8 1) -> (x = y?=w557:bool)
              n365 = Not(x=w561) -> (.not. x?=w560:bool)
              n366 = call "myRIO_BRig_RT_dataMTrig_Audio_N__L.vi"() -> ("output_Audio_N__L"=w575:i32)  [unwired: 11 in]
              n367 = call "myRIO_BRig_RT_dataMTrig_Audio_N__R.vi"() -> ("output_Audio_N__R"=w574:i32)  [unwired: 11 in]
              n368 = Or(x=w560, y=w557) -> (x .or. y?=w558:bool)
              n369 = case shown="True" w558 {
                tunnel: w575 -> [w581 w599]
                tunnel: w574 -> [w580 w598]
                tunnel: w566 -> [w583 w593]
                tunnel: [w582 w593] -> w565
                tunnel: w564 -> [_ w591]
                tunnel: [myRIO_BRig_RT__Case_NonExp_stateList."Idle" ("t") w590] -> w559
                tunnel: w557 -> [_ w589]
                tunnel: w556 -> [_ w585]
                tunnel: w555 -> [_ w584]
                frame False {
                  w576 = u16 0 ("new element/subarray")
                  # "lick occurred and warmupType==2"
                  n370 = call "myRIO_BRig_RT_dataMTrig_Solenoid_N__R.vi"() -> ("output_Solenoid_N__R"=w577:i32)  [unwired: 11 in]
                  n371 = call "myRIO_BRig_RT_dataMTrig_Solenoid_N__L.vi"() -> ("output_Solenoid_N__L"=w578:i32)  [unwired: 11 in]
                  n372 = Replace Array Subset(array=w583, new element #1=w576, index #1=w581, new element #2=w576, index #2=w580, new element #3=w576, index #3=w578, new element #4=w576, index #4=w577) -> (w582:u16[])
                }
                frame True {
                  n373 = Not(x=w589) -> (.not. x?=w588:bool)
                  n374 = Index Array(array=w593, index #1=w599, index #2=w598) -> (element #1=w597:u16, element #2=w596:u16)
                  n375 = Equal To 0?(x=w597) -> (x = 0?=w595:bool)
                  n376 = Equal To 0?(x=w596) -> (x = 0?=w594:bool)
                  n377 = And(x=w595, y=w594) -> (x .and. y?=w587:bool)
                  n378 = And(x=w587, y=w588) -> (x .and. y?=w586:bool)
                  n379 = case shown="True" w586 {
                    tunnel: w585 -> [_ w607]
                    tunnel: w584 -> [_ w602]
                    frame False {
                    }
                    frame True {
                      n380 = local read "count_warmup_R"() -> (w600:u16)
                      n381 = local read "count_warmup_L"() -> (w605:u16)
                      n382 = Increment(x=w600) -> (x+1=w603:u16)
                      n383 = Increment(x=w605) -> (x+1=w606:u16)
                      n384 = Select(t=w603, s=w602, f=w600) -> (s? t:f=w601:u16)
                      n385 = Select(t=w606, s=w607, f=w605) -> (s? t:f=w604:u16)
                      n386 = local write "count_warmup_R"(w601) -> ()
                      n387 = local write "count_warmup_L"(w604) -> ()
                    }
                  }
                  n388 = Select(t=myRIO_BRig_RT__Case_NonExp_stateList."DispenseWater_pre", s=w587, f=w591) -> (s? t:f=w590:T1)
                }
              }
            }
            frame "RewardCalibration_pre" {
              (unwired) FALSE
              w609 = FALSE
              w620 = u8 0
              w636 = u8 0
              # "Are we starting a RewardCalibration?\nOr are we stopping a RewardCalibration?\nOr is a RewardCalibration over?"
              # "RewCalib\nOnOff"
              # "N"
              # "Solenoid R"
              # "RewCalib\nOnOff"
              # "N"
              # "Solenoid L"
              n389 = local read "RewCalib_Trig_L"() -> (w643:bool)
              n390 = local read "RewCalib_Trig_R"() -> (w612:bool)
              n391 = call "myRIO_BRig_RT_dataMTrig_Solenoid_N__R.vi"() -> ("output_Solenoid_N__R"=w614:i32)  [unwired: 11 in]
              n392 = call "myRIO_BRig_RT_dataMTrig_Solenoid_RewCalib_OnOff__R.vi"() -> ("output_Solenoid_RewCalib_OnOff__R"=w611:i32)  [unwired: 11 in]
              n393 = call "myRIO_BRig_RT_dataMTrig_Solenoid_N__L.vi"() -> ("output_Solenoid_N__L"=w629:i32)  [unwired: 11 in]
              n394 = call "myRIO_BRig_RT_dataMTrig_Solenoid_RewCalib_OnOff__L.vi"() -> ("output_Solenoid_RewCalib_OnOff__L"=w630:i32)  [unwired: 11 in]
              n395 = Index Array(array=w613, index #1=w614, index #2=w611) -> (element #1=w624:u16, element #2=w619:u16)
              n396 = Index Array(array=w613, index #1=w629, index #2=w630) -> (element #1=w640:u16, element #2=w635:u16)
              n397 = Equal To 0?(x=w624) -> (x = 0?=w625:bool)
              n398 = Not Equal To 0?(x=w619) -> (x != 0?=w622:bool)
              n399 = Equal To 0?(x=w640) -> (x = 0?=w641:bool)
              n400 = Not Equal To 0?(x=w635) -> (x != 0?=w638:bool)
              n401 = local write "MTrig_Solenoid_trig__L"(w609) -> ()
              n402 = local write "MTrig_Solenoid_trig__R"(w609) -> ()
              n403 = Select(t=u8 1, s=w612, f=w620) -> (s? t:f=w616:u8)
              n404 = Select(t=u8 1, s=w643, f=w636) -> (s? t:f=w632:u8)
              n405 = Select(t=u8 2, s=w625, f=w620) -> (s? t:f=w617:u8)
              n406 = Select(t=u8 4, s=w622, f=w620) -> (s? t:f=w618:u8)
              n407 = Select(t=u8 2, s=w641, f=w636) -> (s? t:f=w633:u8)
              n408 = Select(t=u8 4, s=w638, f=w636) -> (s? t:f=w634:u8)
              n409 = Compound Arithmetic op=ADD(w616, w617, w618) -> (w615:u8)
              n410 = Compound Arithmetic op=ADD(w632, w633, w634) -> (w631:u8)
              n411 = case shown="7" w631 {
                tunnel: w613 -> [w673 w678 w680 w685 w690 w692 w695 w700]
                tunnel: [w673 w679 w680 w686 w691 w692 w696 w701] -> w628
                tunnel: w630 -> [_ w676 _ w683 w688 _ w694 w699]
                tunnel: w629 -> [_ w677 _ w684 w689 _ _ _]
                frame 0, Default {
                }
                frame 1 {
                  n412 = Replace Array Subset(array=w678, new element #1=u16 100 ("new element/subarray"), index #1=w677, new element #2=u16 1 ("new element/subarray"), index #2=w676) -> (w679:u16[])
                }
                frame 2 {
                }
                frame 3 {
                  n413 = Replace Array Subset(array=w685, new element #1=u16 100 ("new element/subarray"), index #1=w684, new element #2=u16 1 ("new element/subarray"), index #2=w683) -> (w686:u16[])
                }
                frame 4 {
                  w687 = u16 0 ("new element/subarray")
                  n414 = Replace Array Subset(array=w690, new element #1=w687, index #1=w689, new element #2=w687, index #2=w688) -> (w691:u16[])
                }
                frame 5 {
                }
                frame 6 {
                  n415 = Replace Array Subset(array=w695, new element=u16 0 ("new element/subarray"), index=w694) -> (w696:u16[])
                }
                frame 7 {
                  n416 = local write "RewCalib_Trig_L"(FALSE ("RewCalib_Trig_L")) -> ()
                  n417 = Replace Array Subset(array=w700, new element=u16 0 ("new element/subarray"), index=w699) -> (w701:u16[])
                }
              }
              n418 = case shown="7" w615 {
                tunnel: w628 -> [w644 w649 w651 w656 w661 w663 w666 w671]
                tunnel: [w644 w650 w651 w657 w662 w663 w667 w672] -> w627
                tunnel: w611 -> [_ w647 _ w654 w659 _ w665 w670]
                tunnel: w614 -> [_ w648 _ w655 w660 _ _ _]
                frame 0, Default {
                }
                frame 1 {
                  n419 = Replace Array Subset(array=w649, new element #1=u16 100 ("new element/subarray"), index #1=w648, new element #2=u16 1 ("new element/subarray"), index #2=w647) -> (w650:u16[])
                }
                frame 2 {
                }
                frame 3 {
                  n420 = Replace Array Subset(array=w656, new element #1=u16 100 ("new element/subarray"), index #1=w655, new element #2=u16 1 ("new element/subarray"), index #2=w654) -> (w657:u16[])
                }
                frame 4 {
                  w658 = u16 0 ("new element/subarray")
                  n421 = Replace Array Subset(array=w661, new element #1=w658, index #1=w660, new element #2=w658, index #2=w659) -> (w662:u16[])
                }
                frame 5 {
                }
                frame 6 {
                  n422 = Replace Array Subset(array=w666, new element=u16 0 ("new element/subarray"), index=w665) -> (w667:u16[])
                }
                frame 7 {
                  n423 = local write "RewCalib_Trig_R"(FALSE ("RewCalib_Trig_L")) -> ()
                  n424 = Replace Array Subset(array=w671, new element=u16 0 ("new element/subarray"), index=w670) -> (w672:u16[])
                }
              }
            }
            frame "DispenseWater_pre" {
              w708 = u16 0 ("t")
              w751 = u16 0 ("new element/subarray")
              # "just trust me on this one"
              # "RewCalib\nOnOff"
              # "RewCalib\nOnOff"
              # "nCycle"
              # "Solenoid__R"
              # "Tdelay"
              # "delay"
              # "nCycle"
              # "Solenoid__L"
              # "Tdelay"
              # "delay"
              # "Solenoid__R"
              # "count"
              # "Solenoid_Tcycle_R"
              # "Solenoid_Tcycle_L"
              # "Solenoid__L"
              # "count"
              n425 = call "myRIO_BRig_RT_dataMTrig_Solenoid_RewCalib_OnOff__L.vi"() -> ("output_Solenoid_RewCalib_OnOff__L"=w715:i32)  [unwired: 11 in]
              n426 = call "myRIO_BRig_RT_dataMTrig_Solenoid_N__L.vi"() -> ("output_Solenoid_N__L"=w706:i32)  [unwired: 11 in]
              n427 = call "myRIO_BRig_RT_dataMTrig_Solenoid_delay__L.vi"() -> ("output_Solenoid_delay__L"=w749:i32)  [unwired: 11 in]
              n428 = call "myRIO_BRig_RT_dataMTrig_Solenoid_Tdelay__L.vi"() -> ("output_Solenoid_Tdelay__L"=w748:i32)  [unwired: 11 in]
              n429 = call "myRIO_BRig_RT_dataMTrig_Solenoid_N__R.vi"() -> ("output_Solenoid_N__R"=w704:i32)  [unwired: 11 in]
              n430 = call "myRIO_BRig_RT_dataMTrig_Solenoid_delay__R.vi"() -> ("output_Solenoid_delay__R"=w738:i32)  [unwired: 11 in]
              n431 = call "myRIO_BRig_RT_dataMTrig_Solenoid_Tdelay__R.vi"() -> ("output_Solenoid_Tdelay__R"=w737:i32)  [unwired: 11 in]
              n432 = call "myRIO_BRig_RT_dataMTrig_Solenoid_RewCalib_OnOff__R.vi"() -> ("output_Solenoid_RewCalib_OnOff__R"=w711:i32)  [unwired: 11 in]
              n433 = Index Array(array=w750, index #1=w706, index #2=w749, index #3=w748, index #4=w704, index #5=w738, index #6=w737, index #7=w715, index #8=w711) -> (element #1=w707:u16, element #2=w747:u16, element #3=w742:u16, element #4=w710:u16, element #5=w732:u16, element #6=w731:u16, element #7=w716:u16, element #8=w713:u16)
              n434 = Equal To 0?(x=w747) -> (x = 0?=w746:bool)
              n435 = Equal To 0?(x=w732) -> (x = 0?=w736:bool)
              n436 = local read "RewCalib_Trig_L"() -> (w727:bool)
              n437 = local read "RewCalib_Trig_R"() -> (w722:bool)
              n438 = Not Equal To 0?(x=w707) -> (x != 0?=w745:bool)
              n439 = Not Equal To 0?(x=w710) -> (x != 0?=w735:bool)
              n440 = local read "MTrig_Solenoid_Tcycle__L"() -> (w744:u16)
              n441 = local read "MTrig_Solenoid_Tcycle__R"() -> (w730:u16)
              n442 = Not Equal To 0?(x=w716) -> (x != 0?=w726:bool)
              n443 = Not Equal To 0?(x=w713) -> (x != 0?=w724:bool)
              n444 = Not(x=w727) -> (.not. x?=w725:bool)
              n445 = Not(x=w722) -> (.not. x?=w723:bool)
              n446 = And(x=w726, y=w725) -> (x .and. y?=w721:bool)
              n447 = And(x=w724, y=w723) -> (x .and. y?=w720:bool)
              n448 = call "myRIO_BRig_RT_dataMTrig_Solenoid_c__L.vi"() -> ("output_Solenoid_c__L"=w753:i32)  [unwired: 11 in]
              n449 = call "myRIO_BRig_RT_dataMTrig_Solenoid_c__R.vi"() -> ("output_Solenoid_c__R"=w752:i32)  [unwired: 11 in]
              n450 = Select(t=w744, s=w745, f=u16 0) -> (s? t:f=w741:u16)
              n451 = Or(x=w721, y=w720) -> (x .or. y?=w709:bool)
              n452 = Select(t=w730, s=w735, f=u16 0) -> (s? t:f=w733:u16)
              n453 = Select(t=w741, s=w746, f=w742) -> (s? t:f=w739:u16)
              n454 = Select(t=w733, s=w736, f=w731) -> (s? t:f=w728:u16)
              n455 = call "myRIO_BRig_RT_dataMTrig_Solenoid_Tcycle__L.vi"() -> ("output_Solenoid_Tcycle__L"=w740:i32)  [unwired: 11 in]
              n456 = call "myRIO_BRig_RT_dataMTrig_Solenoid_Tcycle__R.vi"() -> ("output_Solenoid_Tcycle__R"=w729:i32)  [unwired: 11 in]
              n457 = Select(t=w708, s=w709, f=w707) -> (s? t:f=w705:u16)
              n458 = Select(t=w708, s=w709, f=w710) -> (s? t:f=w703:u16)
              n459 = Select(t=myRIO_BRig_RT__Case_NonExp_stateList."Idle" ("Enum"), s=w709, f=myRIO_BRig_RT__Case_NonExp_stateList."DispenseWater" ("Enum")) -> (s? t:f=w717:T1)
              n460 = Select(t=w708, s=w709, f=w716) -> (s? t:f=w714:u16)
              n461 = Select(t=w708, s=w709, f=w713) -> (s? t:f=w712:u16)
              n462 = Replace Array Subset(array=w750, new element #1=w751, index #1=w753, new element #2=w751, index #2=w752, new element #3=w739, index #3=w740, new element #4=w728, index #4=w729, new element #5=w714, index #5=w715, new element #6=w712, index #6=w711, new element #7=w705, index #7=w706, new element #8=w703, index #8=w704) -> (w754:u16[])
            }
            frame "DispenseWater" {
              # "D"
              # "C"
              # "B"
              # "A"
              # "(A) Add COUNT and INCREMENT\n(B) Is (A) smaller than Tcycle?\n(C) Are we dispensing water or in the delay phase?\n(D) If (A) is smaller than Tcycle   AND   if we are dispensing water\n      then send TRUE to solenoid"
              # "delay"
              # "Tcycle"
              # "Solenoid__R"
              # "count"
              # "delay"
              # "Tcycle"
              # "Solenoid__L"
              # "count"
              n463 = To Unsigned Word Integer(number=w782) -> (unsigned 16bit integer=w764:u16)
              n464 = call "myRIO_BRig_RT_dataMTrig_Solenoid_delay__R.vi"() -> ("output_Solenoid_delay__R"=w768:i32)  [unwired: 11 in]
              n465 = call "myRIO_BRig_RT_dataMTrig_Solenoid_c__R.vi"() -> ("output_Solenoid_c__R"=w767:i32)  [unwired: 11 in]
              n466 = call "myRIO_BRig_RT_dataMTrig_Solenoid_Tcycle__R.vi"() -> ("output_Solenoid_Tcycle__R"=w769:i32)  [unwired: 11 in]
              n467 = call "myRIO_BRig_RT_dataMTrig_Solenoid_delay__L.vi"() -> ("output_Solenoid_delay__L"=w784:i32)  [unwired: 11 in]
              n468 = call "myRIO_BRig_RT_dataMTrig_Solenoid_c__L.vi"() -> ("output_Solenoid_c__L"=w776:i32)  [unwired: 11 in]
              n469 = call "myRIO_BRig_RT_dataMTrig_Solenoid_Tcycle__L.vi"() -> ("output_Solenoid_Tcycle__L"=w785:i32)  [unwired: 11 in]
              n470 = Index Array(array=w778, index #1=w776, index #2=w785, index #3=w784, index #4=w767, index #5=w769, index #6=w768) -> (element #1=w783:u16, element #2=w773:u16, element #3=w781:u16, element #4=w763:u16, element #5=w760:u16, element #6=w759:u16)
              n471 = Add(x=w783, y=w764) -> (x+y=w774:u16)
              n472 = Add(x=w763, y=w764) -> (x+y=w765:u16)
              n473 = Less?(x=w774, y=w773) -> (x < y?=w757:bool)
              n474 = Equal To 0?(x=w781) -> (x = 0?=w780:bool)
              n475 = Less?(x=w765, y=w760) -> (x < y?=w758:bool)
              n476 = Equal To 0?(x=w759) -> (x = 0?=w766:bool)
              n477 = And(x=w757, y=w780) -> (x .and. y?=w779:bool)
              n478 = Or(x=w757, y=w758) -> (x .or. y?=w756:bool)
              n479 = And(x=w758, y=w766) -> (x .and. y?=w761:bool)
              n480 = Select(t=w774, s=w757, f=w773) -> (s? t:f=w775:u16)
              n481 = Select(t=w765, s=w758, f=w760) -> (s? t:f=w762:u16)
              n482 = Replace Array Subset(array=w778, new element #1=w775, index #1=w776, new element #2=w762, index #2=w767) -> (w777:u16[])
              n483 = Select(t=w772, s=w756, f=myRIO_BRig_RT__Case_NonExp_stateList."DispenseWater_post" ("Enum")) -> (s? t:f=w770:T1)
            }
            frame "DispenseWater_post" {
              # "nCycle"
              # "delay"
              # "Solenoid__R"
              # "nCycle"
              # "delay"
              # "Solenoid__L"
              n484 = call "myRIO_BRig_RT_dataMTrig_Solenoid_N__L.vi"() -> ("output_Solenoid_N__L"=w803:i32)  [unwired: 11 in]
              n485 = call "myRIO_BRig_RT_dataMTrig_Solenoid_delay__L.vi"() -> ("output_Solenoid_delay__L"=w802:i32)  [unwired: 11 in]
              n486 = call "myRIO_BRig_RT_dataMTrig_Solenoid_N__R.vi"() -> ("output_Solenoid_N__R"=w799:i32)  [unwired: 11 in]
              n487 = call "myRIO_BRig_RT_dataMTrig_Solenoid_delay__R.vi"() -> ("output_Solenoid_delay__R"=w798:i32)  [unwired: 11 in]
              n488 = Index Array(array=w805, index #1=w803, index #2=w802, index #3=w799, index #4=w798) -> (element #1=w807:u16, element #2=w806:u16, element #3=w790:u16, element #4=w792:u16)
              n489 = Not Equal To 0?(x=w807) -> (x != 0?=w808:bool)
              n490 = Not Equal To 0?(x=w790) -> (x != 0?=w791:bool)
              n491 = case shown="True" w791 {
                selector: w791 -> [_ w812]
                tunnel: w790 -> [w810 w818]
                tunnel: w792 -> [_ w819]
                tunnel: [w810 w816] -> w789
                tunnel: [u16 0 w815] -> w788
                tunnel: [_ w812] -> w787
                frame False {
                }
                frame True {
                  n492 = Equal To 0?(x=w819) -> (x = 0?=w811:bool)
                  n493 = Decrement(x=w818) -> (x-1=w817:u16)
                  n494 = Select(t=w817, s=w811, f=w818) -> (s? t:f=w816:u16)
                  n495 = Select(t=u16 1, s=w811, f=u16 0) -> (s? t:f=w815:u16)
                }
              }
              n496 = case shown="True" w808 {
                selector: w808 -> [_ w823]
                tunnel: w807 -> [w821 w829]
                tunnel: w806 -> [_ w830]
                tunnel: [w821 w827] -> w801
                tunnel: [u16 0 w826] -> w800
                tunnel: [_ w823] -> w797
                frame False {
                }
                frame True {
                  n497 = Equal To 0?(x=w830) -> (x = 0?=w822:bool)
                  n498 = Decrement(x=w829) -> (x-1=w828:u16)
                  n499 = Select(t=w828, s=w822, f=w829) -> (s? t:f=w827:u16)
                  n500 = Select(t=u16 1, s=w822, f=u16 0) -> (s? t:f=w826:u16)
                }
              }
              n501 = Or(x=w797, y=w787) -> (x .or. y?=w796:bool)
              n502 = Replace Array Subset(array=w805, new element #1=w801, index #1=w803, new element #2=w800, index #2=w802, new element #3=w789, index #3=w799, new element #4=w788, index #4=w798) -> (w804:u16[])
              n503 = Select(t=myRIO_BRig_RT__Case_NonExp_stateList."DispenseWater_pre" ("Enum"), s=w796, f=myRIO_BRig_RT__Case_NonExp_stateList."Idle" ("Enum")) -> (s? t:f=w793:T1)
            }
            frame "TestConnection" {
              n504 = local read "Host Password"() -> (w837:string)
              n505 = local read "Host UserName"() -> (w838:string)
              n506 = call "myRIO_BRig_RT_comm_webdav_testConnect.vi"("input_password"=w837, "input_username"=w838) -> ("output_Iconnected"=w835:bool)  [unwired: 9 in]
              n507 = Select(t="Connection accepted!" ("message"), s=w835, f="Error!") -> (s? t:f=w833:string)
              n508 = One Button Dialog(message=w833) -> ()  [unwired: 1 in, 1 out]
            }
            frame "SendData" {
              n509 = local read "Data Set Prefix"() -> (w840:string)
              n510 = local read "Host Password"() -> (w841:string)
              n511 = local read "Host UserName"() -> (w842:string)
              n512 = call "myRIO_BRig_RT_comm_webdav_sendData_all.vi"("Host Filename Prefix"=w840, "Host Password"=w841, "Host UserName"=w842) -> ()  [unwired: 9 in]
            }
            frame "Get_FPGA_count_per_ms" {
              n513 = case shown="False" w856 {
                selector: w856 -> [w859 _]
                tunnel: w854 -> [_ w872]
                tunnel: [w863 w872] -> w853
                tunnel: w852 -> [w862 w870]
                tunnel: w851 -> [w861 w869]
                tunnel: [w860 w867] -> w850
                tunnel: [w859 w866] -> w849
                frame False {
                  n514 = Get Date/Time In Seconds() -> (seconds since 1Jan1904=w864:timestamp)
                  n515 = xnode "Read/Write Control"("FPGA VI Reference In"=w862, "error in"=w861, "timeTrial"=TRUE) -> ("error out"=w860:errorcluster)  [unwired: 1 out]
                  n516 = To Double Precision Float(number=w864) -> (double precision float=w863:dbl)
                  n517 = local write "get_countPerMS"(w859) -> ()
                }
                frame True {
                  w868 = 1.0
                  n518 = Get Date/Time In Seconds() -> (seconds since 1Jan1904=w873:timestamp)
                  n519 = To Double Precision Float(number=w873) -> (double precision float=w874:dbl)
                  n520 = Subtract(x=w874, y=w872) -> (x-y=w871:dbl)
                  n521 = Less Or Equal?(x=w868, y=w871) -> (x <= y?=w866:bool)
                  n522 = case shown="True" w866 {
                    tunnel: w870 -> [_ w887]
                    tunnel: w869 -> [w875 w886]
                    tunnel: w868 -> [_ w877]
                    tunnel: [w875 w876] -> w867
                    frame False {
                    }
                    frame True {
                      n523 = xnode "Read/Write Control"("FPGA VI Reference In"=w887, "error in"=w886) -> ("FPGA VI Reference Out"=w884:refnum<k20>, "error out"=w883:errorcluster, "count_timeTrial"=w878:u32)
                      n524 = Multiply(x=w877, y=1000.0) -> (x*y=w881:dbl)
                      n525 = To Double Precision Float(number=w878) -> (double precision float=w880:dbl)
                      n526 = Divide(x=w880, y=w881) -> (x/y=w882:dbl)
                      n527 = local write "f_millisec2count"(w882) -> ()
                      n528 = xnode "Read/Write Control"("FPGA VI Reference In"=w884, "error in"=w883, "timeTrial"=FALSE) -> ("error out"=w876:errorcluster)  [unwired: 1 out]
                    }
                  }
                }
              }
              "error out 5" <- w850
              n529 = Select(t=myRIO_BRig_RT__Case_NonExp_stateList."Idle" ("Enum"), s=w849, f=w847) -> (s? t:f=w846:T1)
            }
            frame "End" {
            }
          }
          n530 = local read "MTrig_Audio_trig__R"() -> (w93:bool)
          n531 = local read "MTrig_Audio_trig__L"() -> (w92:bool)
          n532 = local read "START"() -> (w88:bool)
          n533 = local read "STOP_abort"() -> (w87:bool)
          n534 = local read "MTrig_Laser_trig"() -> (w94:bool)
          n535 = call "myRIO_BRig_RT_dataMTrig_main__v2.vi"("input_dataMTrig"=w96, "input_Audio_trig_L"=w92, "input_Audio_trig_R"=w93, "input_Laser_trig"=w94) -> ("output_dataMTrig"=w95:u16[], "output_Audio_L"=w72:bool, "output_Audio_R"=w83:bool, "output_Laser"=w75:bool)  [unwired: 12 in]
          n536 = Or(x=w88, y=w87) -> (x .or. y?=w86:bool)
          n537 = Select(t=myRIO_BRig_RT__Case_NonExp_stateList."End" ("Enum"), s=w86, f=w85) -> (s? t:f=w84:T1)
          n538 = Or(x=w93, y=w94) -> (x .or. y?=w91:bool)
          n539 = Or(x=w91, y=w92) -> (x .or. y?=w90:bool)
          n540 = case shown="True" w90 {
            frame False {
            }
            frame True {
              w109 = FALSE
              n541 = local write "MTrig_Audio_trig__R"(w109) -> ()
              n542 = local write "MTrig_Audio_trig__L"(w109) -> ()
              n543 = local write "MTrig_Laser_trig"(w109) -> ()
            }
          }
          n544 = xnode "Read/Write Control"("FPGA VI Reference In"=w61, "error in"=w60, "A1_SR"=w97, "A3_SL"=w98, "audioTrigger_L"=w72, "audioTrigger_R"=w83, "laserResponse_reward_LED"="laserResponse_reward_LED", "laserResponse_wrong_LED"="laserResponse_wrong_LED", "laserResponse_reward"="laserResponse_reward", "laserResponse_wrong"="laserResponse_wrong", "SelectionState"="SelectionState", "ignoreWrong"="ignoreWrong", "Left(F)_or_Right(T)"="Left(F)_or_Right(T)", "laserMTrig"=w75) -> ("FPGA VI Reference Out"=w103:refnum<k20>, "error out"=w102:errorcluster, "SelectReward"=→"SelectReward":bool, "SelectWrong"=→"SelectWrong":bool, "AnaIn_0"=→"tempAI0":u16)
          n545 = node-c288() -> ()  [unwired: 1 in, 1 out]
          "cState_NonExp" <- w101
        }
        n546 = node-c288(w50) -> ()  [unwired: 1 out]
        n547 = flat-sequence {
          tunnel: w43 -> [w54]
          tunnel: [w54] -> w42
          tunnel: w41 -> [w53]
          tunnel: [w53] -> w40
          frame #0 {
            w52 = FALSE
            n548 = local write "STOP_endBlock"(w52) -> ()
            n549 = local write "STOP_endTrial"(w52) -> ()
          }
        }
      }
      frame True {
        w900 = u16 0
        w903 = u8 0
        w905 = FALSE ("SelectionState")
        w910 = u16 0 ("idxDataBlock")
        w912 = u16 100 ("new element/subarray")
        w913 = u16 100 ("new element/subarray")
        w933 = T6 refnum items=["Session NI_WebDAV"] ("output_hSession")
        w942 = FALSE
        w943 = u16 0
        w904 = FALSE
        # "audio__L\naudio__R"
        # "Audio params"
        # "nRewards"
        # "idxDataBlock"
        # "Solenoid_Tdelay_R"
        # "Solenoid_Tdelay_L"
        # "RewCalib_N__R"
        # "RewCalib_N__L"
        # "Save dataLick to file\nSend file to Host\nSave dataMTrig\nSend file to Host\nDisconnect"
        # "dataTrial"
        # "dataTrial"
        # "Solenoid_Tcycle_R"
        # "Solenoid_Tcycle_L"
        # "Laser_Tcycle"
        # "Audio_Tcycle_R"
        # "Audio_Tcycle_L"
        # "dataLick"
        # "dataLC"
        # "dataLC"
        # "dataBlock"
        # "dataBlock"
        # "dataMTrig"
        # "dataMTrig"
        # "dataExp"
        # "dataCurrent"
        # "dataExp"
        # "dataCurrent"
        # "spout"
        # "state"
        n550 = call "myRIO_BRig_RT_dataMTrig_Solenoid_Tcycle__L.vi"() -> ("output_Solenoid_Tcycle__L"=w939:i32)  [unwired: 11 in]
        n551 = call "myRIO_BRig_RT_dataMTrig_Solenoid_Tcycle__R.vi"() -> ("output_Solenoid_Tcycle__R"=w938:i32)  [unwired: 11 in]
        n552 = call "myRIO_BRig_RT_dataMTrig_Audio_Tcycle__L.vi"() -> ("output_Audio_Tcycle__L"=w937:i32)  [unwired: 11 in]
        n553 = call "myRIO_BRig_RT_dataMTrig_Audio_Tcycle__R.vi"() -> ("output_Audio_Tcycle__R"=w936:i32)  [unwired: 11 in]
        n554 = call "myRIO_BRig_RT_dataMTrig_Laser_Tcycle.vi"() -> ("output_Laser_Tcycle"=w935:i32)  [unwired: 11 in]
        n555 = local read "MTrig_Solenoid_Tcycle__L"() -> (w918:u16)
        n556 = local read "MTrig_Solenoid_Tcycle__R"() -> (w917:u16)
        n557 = local read "Tcycle_Reward_L"() -> (w914:u16)
        n558 = local read "Tcycle_Reward_R"() -> (w915:u16)
        n559 = local read "MTrig_Laser_Tcycle"() -> (w916:u16)
        n560 = call "myRIO_BRig_RT_dataMTrig_Solenoid_RewCalib_nCycle__L.vi"() -> ("output_Solenoid_RewCalib_nCycle__L"=w921:i32)  [unwired: 11 in]
        n561 = call "myRIO_BRig_RT_dataMTrig_Solenoid_Tdelay__L.vi"() -> ("output_Solenoid_Tdelay__L"=w923:i32)  [unwired: 11 in]
        n562 = call "myRIO_BRig_RT_dataMTrig_Solenoid_RewCalib_nCycle__R.vi"() -> ("output_Solenoid_RewCalib_nCycle__R"=w922:i32)  [unwired: 11 in]
        n563 = call "myRIO_BRig_RT_dataMTrig_Solenoid_Tdelay__R.vi"() -> ("output_Solenoid_Tdelay__R"=w924:i32)  [unwired: 11 in]
        n564 = call "myRIO_BRig_RT_dataLick_init.vi"() -> ("output_dataLick"=w945:u16[][])  [unwired: 11 in]
        n565 = call "myRIO_BRig_RT_dataCurrent_init.vi"() -> ("output_dataCurrent"=w952:u16[])  [unwired: 11 in]
        n566 = call "myRIO_BRig_RT_dataExp_init.vi"() -> ("output_dataExp"=w951:u16[])  [unwired: 11 in]
        n567 = call "myRIO_BRig_RT_dataMTrig_init.vi"() -> ("output_dataMTrig"=w941:u16[])  [unwired: 5 in]
        n568 = call "myRIO_BRig_RT_dataLC_init.vi"() -> ("output_dataLC"=w949:u16[])  [unwired: 11 in]
        n569 = call "myRIO_BRig_RT_dataBlock_init.vi"() -> ("output_dataBlock"=w950:u16[][])  [unwired: 11 in]
        n570 = call "myRIO_BRig_RT_dataTrial_init.vi"() -> ("output_dataTrial"=w934:u16[][])  [unwired: 11 in]
        n571 = xnode "Read/Write Control"("FPGA VI Reference In"=w906, "error in"=w907, "SelectionState"=w905, "laserResponse_reward"=w905, "laserResponse_wrong"=w905, "laserResponse_reward_LED"=w905, "laserResponse_wrong_LED"=w905, "Left(F)_or_Right(T)"=w905, "ignoreWrong"=w905, "SelectionState"=w905) -> ("FPGA VI Reference Out"=w908:refnum<k20>, "error out"=w909:errorcluster)
        n572 = Replace Array Subset(array=w941, new element #1=w913, index #1=w921, new element #2=w913, index #2=w922, new element #3=w912, index #3=w923, new element #4=w912, index #4=w924, new element #5=w918, index #5=w939, new element #6=w917, index #6=w938, new element #7=w914, index #7=w937, new element #8=w915, index #8=w936, new element #9=w916, index #9=w935) -> (w940:u16[])
        n573 = call "myRIO_BRig_RT_dataAnalog_init.vi"() -> ("output_dataAnalog"=w899:u16[][])  [unwired: 11 in]
        n574 = Get Date/Time In Seconds() -> (seconds since 1Jan1904=w920:timestamp)
        n575 = To Double Precision Float(number=w920) -> (double precision float=w919:dbl)
        n576 = node-c288() -> (w960:T3)  [unwired: 4 in]
        n577 = timed-loop {
          timing: w960 -> [_]
          timing-out: [_] -> w959
          shift-right: [w1066] -> _
          shift-left: myRIO_BRig_RT__Case_Exp_stateList."Start1" ("Enum") -> [w1013]
          shift-right: [w1117] -> _
          shift-left: enum16{"Left", "Right"}."Left" -> [w1119]
          tunnel: w908 -> [w1116]
          tunnel: w909 -> [w1115]
          shift-right: [w1110] -> _
          shift-left: w957 -> [w1114]
          shift-right: [w1109] -> _
          shift-left: w956 -> [w1113]
          tunnel: [w1091] -> w954
          tunnel: [w1092] -> w955
          shift-right: [w1093] -> w925
          shift-left: w952 -> [w1058]
          shift-right: [w1108] -> _
          shift-left: w951 -> [w1053]
          shift-right: [w1080] -> w929
          shift-left: w940 -> [w1081]
          shift-right: [w1106] -> _
          shift-left: w950 -> [w1107]
          shift-right: [w1104] -> _
          shift-left: w949 -> [w1105]
          shift-right: [w1039] -> _
          shift-left: w904 -> [w1103]
          shift-right: [w1095] -> w931
          shift-left: w945 -> [w1096]
          shift-right: [w1082] -> _
          shift-left: w943 -> [w1090]
          shift-right: [w1050] -> _
          shift-left: w903 -> [w1089]
          shift-right: [w1083] -> _
          shift-left: w943 -> [w1088]
          shift-right: [w1084] -> _
          shift-left: w903 -> [w1087]
          shift-right: [w1051] -> _
          shift-left: w942 -> [w1085]
          shift-right: [w1052] -> _
          shift-left: w942 -> [w1086]
          shift-right: [w1064] -> _
          shift-left: w934 -> [w1065]
          shift-right: [w1063] -> w927
          shift-left: w933 -> [w1061]
          shift-right: [w1062] -> w928
          shift-left: FALSE ("output_Iconnected") -> [w1060]
          tunnel: "Data Set Prefix" -> [w1059]
          tunnel: [w1059] -> w926
          shift-right: [w1034] -> _
          shift-left: w904 -> [w1057]
          tunnel: w919 -> [w1054]
          shift-right: [w1048] -> _
          shift-left: 0 ("idxDataBlock") -> [w1049]
          shift-right: [w1045] -> _
          shift-left: w910 -> [w1047]
          shift-right: [w1044] -> _
          shift-left: w910 -> [w1046]
          shift-right: [w1033] -> _
          shift-left: w904 -> [w1040]
          shift-right: [w1036] -> _
          shift-left: w904 -> [w1038]
          shift-right: [w1035] -> _
          shift-left: w904 -> [w1037]
          shift-right: [w1026] -> _
          shift-left: w904 -> [w1027]
          shift-right: [w1018] -> w897
          shift-left: 0 -> [w1017]
          shift-right: [w1006] -> _
          shift-left: w900 -> [w1011]
          shift-right: [w1005] -> _
          shift-left: w900 -> [w1007]
          shift-right: [w1023] -> _
          shift-left: FALSE -> [w1023]
          shift-right: [w1002] -> _
          shift-left: w900 -> [w1015]
          shift-right: [w1020] -> w898
          shift-left: w899 -> [w1021]
          stop <- w1102 stop-if-true
          # "iState"
          # "dataAnalog"
          # "index"
          # "iEvent"
          # "iBlock"
          # "iTrial"
          # "Laser"
          # "Audio R"
          # "Audio L"
          # "Solenoid R"
          # "Solenoid L"
          # "manual triggering"
          # "dataTrial"
          # "dataBlock"
          # "nRewards"
          # "laserOccurred"
          # "dataExp"
          # "dataCurrent"
          # "audio__L\naudio__R"
          # "time stamp"
          # "Audio params"
          # "nRewards"
          # "idxDataBlock"
          # "idxDataBlock"
          # "activate"
          # "audio__L\naudio__R"
          # "amp__R\nfreq__R"
          # "amp__L\nfreq__L"
          # "dataLC"
          # "solenoid__R"
          # "solenoid__L"
          # "Did a lick occur?"
          # "Update lick counter"
          # "spout"
          # "spout"
          # "state"
          # "state"
          n578 = node-c288() -> ()  [unwired: 1 in, 1 out]
          n579 = local read "MTrig_Solenoid_trig__L"() -> (w1078:bool)
          n580 = local read "MTrig_Solenoid_trig__R"() -> (w1077:bool)
          n581 = local read "MTrig_Audio_trig__L"() -> (w1076:bool)
          n582 = local read "MTrig_Audio_trig__R"() -> (w1075:bool)
          n583 = xnode "Read/Write Control"("FPGA VI Reference In"=w1116, "error in"=w1115) -> ("FPGA VI Reference Out"=w1043:refnum<k20>, "error out"=w1042:errorcluster, "A2_LickL"=w1110:u32, "A4_LickR"=w1109:u32)
          "A2" <- w1110
          "A4" <- w1109
          n584 = local read "MTrig_Laser_trig"() -> (w1074:bool)
          n585 = Greater?(x=w1110, y=w1114) -> (0:w1112:bool)
          n586 = Greater?(x=w1109, y=w1113) -> (0:w1111:bool)
          n587 = Or(x=w1112, y=w1111) -> (x .or. y?=w1118:bool)
          n588 = call "myRIO_BRig_RT_dataMTrig_main.vi"("input_dataMTrig"=w1081, "input_Solenoid_trig_L"=w1078, "input_Solenoid_trig_R"=w1077, "input_Audio_trig_L"=w1076, "input_Audio_trig_R"=w1075, "input_Laser_trig"=w1074) -> ("output_Laser"=w1031:bool, "output_dataMTrig"=w1080:u16[], "output_Solenoid_L"=w1068:bool, "output_Solenoid_R"=w1070:bool, "output_Audio_L"=w1072:bool, "output_Audio_R"=w1073:bool)  [unwired: 8 in]
          n589 = Compound Arithmetic op=OR(w1078, w1077, w1076, w1075, w1074) -> (w1079:bool)
          n590 = case shown="True" w1079 {
            frame False {
            }
            frame True {
              w1120 = FALSE
              n591 = local write "MTrig_Solenoid_trig__L"(w1120) -> ()
              n592 = local write "MTrig_Solenoid_trig__R"(w1120) -> ()
              n593 = local write "MTrig_Audio_trig__L"(w1120) -> ()
              n594 = local write "MTrig_Audio_trig__R"(w1120) -> ()
              n595 = local write "MTrig_Laser_trig"(w1120) -> ()
            }
          }
          n596 = case shown="\"initTrial3\"" w1013 {
            selector: w1013 -> [_ _ _ _ _ _ _ _ _ _ _ _ _ _ _ _ _ _ _ _ w1861 _ w1926 _ _ _ _ _ w2068 _ w2143 _ _ _ _ _ w2272 _ w2348 _ w2412 _ w2456 _ _ w2526 _ _ _ _ _ w2698 _ _ _ _ _ _ _ _ _ _ _ _ _ _ _ _ _ _ _]
            tunnel: [myRIO_BRig_RT__Case_Exp_stateList."Start2" ("Enum") myRIO_BRig_RT__Case_Exp_stateList."Start3" ("Enum") myRIO_BRig_RT__Case_Exp_stateList."saveSettings1" ("Enum") myRIO_BRig_RT__Case_Exp_stateList."saveSettings2" ("Enum") myRIO_BRig_RT__Case_Exp_stateList."saveSettings3" ("Enum") myRIO_BRig_RT__Case_Exp_stateList."saveSettings4_LC_ENL" ("Enum") myRIO_BRig_RT__Case_Exp_stateList."saveSettings5_LC_Cue" ("Enum") myRIO_BRig_RT__Case_Exp_stateList."saveSettings6_LC_Other" ("Enum") myRIO_BRig_RT__Case_Exp_stateList."setSettings_Audio" ("Enum") myRIO_BRig_RT__Case_Exp_stateList."setSettings_Laser" ("Enum") myRIO_BRig_RT__Case_Exp_stateList."commConnect" ("Enum") w1619 myRIO_BRig_RT__Case_Exp_stateList."initTrial" ("Enum") w1664 myRIO_BRig_RT__Case_Exp_stateList."initTrial3" ("Enum") myRIO_BRig_RT__Case_Exp_stateList."initTrial_LC_ENL1" ("Enum") myRIO_BRig_RT__Case_Exp_stateList."ENL1_pre" ("Enum") myRIO_BRig_RT__Case_Exp_stateList."initTrial_LC_Cue1" ("Enum") myRIO_BRig_RT__Case_Exp_stateList."initTrial4" ("Enum") w1820 w1858 myRIO_BRig_RT__Case_Exp_stateList."ENL1Penalty" ("Enum") w1927 myRIO_BRig_RT__Case_Exp_stateList."endExp" ("Enum") myRIO_BRig_RT__Case_Exp_stateList."endExp" ("Enum") myRIO_BRig_RT__Case_Exp_stateList."endExp" ("Enum") myRIO_BRig_RT__Case_Exp_stateList."endExp" ("Enum") w2022 w2067 myRIO_BRig_RT__Case_Exp_stateList."Cue1Penalty" ("Enum") w2141 myRIO_BRig_RT__Case_Exp_stateList."endExp" ("Enum") myRIO_BRig_RT__Case_Exp_stateList."endExp" ("Enum") myRIO_BRig_RT__Case_Exp_stateList."endExp" ("Enum") myRIO_BRig_RT__Case_Exp_stateList."endExp" ("Enum") w2229 w2280 myRIO_BRig_RT__Case_Exp_stateList."SelectReward" ("Enum") w2349 myRIO_BRig_RT__Case_Exp_stateList."SelectRewardPost" ("Enum") w2413 myRIO_BRig_RT__Case_Exp_stateList."SelectWrong" ("Enum") w2452 myRIO_BRig_RT__Case_Exp_stateList."endTrial1" ("Enum") myRIO_BRig_RT__Case_Exp_stateList."SelectTimeout" ("Enum") w2528 myRIO_BRig_RT__Case_Exp_stateList."endTrial1" ("Enum") myRIO_BRig_RT__Case_Exp_stateList."endTrial2" ("Enum") myRIO_BRig_RT__Case_Exp_stateList."saveData_dataBlock" ("Enum") w2611 w2681 w2698 myRIO_BRig_RT__Case_Exp_stateList."initBlock" ("Enum") w2725 myRIO_BRig_RT__Case_Exp_stateList."commUpload_dataCurrent" ("Enum") myRIO_BRig_RT__Case_Exp_stateList."commUpload_dataExp" ("Enum") myRIO_BRig_RT__Case_Exp_stateList."commUpload_dataLC" ("Enum") myRIO_BRig_RT__Case_Exp_stateList."commUpload_dataTrial" ("Enum") myRIO_BRig_RT__Case_Exp_stateList."endTrial3" ("Enum") myRIO_BRig_RT__Case_Exp_stateList."saveData_dataCurrent" ("Enum") myRIO_BRig_RT__Case_Exp_stateList."saveData_dataExp" ("Enum") myRIO_BRig_RT__Case_Exp_stateList."saveData_dataLC" ("Enum") myRIO_BRig_RT__Case_Exp_stateList."saveData_dataTrial" ("Enum") myRIO_BRig_RT__Case_Exp_stateList."commUpload_pre" ("Enum") myRIO_BRig_RT__Case_Exp_stateList."empty_endBlock2" ("Enum") myRIO_BRig_RT__Case_Exp_stateList."initBlock" ("Enum") myRIO_BRig_RT__Case_Exp_stateList."empty_endTrial2" ("Enum") myRIO_BRig_RT__Case_Exp_stateList."empty_endTrial3" ("Enum") myRIO_BRig_RT__Case_Exp_stateList."empty_endTrial4" ("Enum") myRIO_BRig_RT__Case_Exp_stateList."empty_endTrial5" ("Enum") myRIO_BRig_RT__Case_Exp_stateList."initTrial" ("Enum")] -> w1066
            tunnel: [w1146 w1165 w1187 w1242 w1290 w1357 w1409 w1461 w1505 w1531 w1590 w1596 w1627 w1646 w1680 w1710 w1743 w1768 w1795 w1836 w1874 w1904 w1931 w1947 w1969 w1988 w2007 w2041 w2089 w2114 w2140 w2161 w2182 w2201 w2220 w2240 w2298 w2323 w2346 w2360 w2410 w2434 w2466 w2487 w2507 w2539 w2562 w2574 w2593 w2635 w2654 w2697 w2714 w2728 w2762 w2783 w2804 w2825 w2846 w2874 w2894 w2921 w2941 w2966 w2985 w3004 w3023 w3042 w3061 w3080 w3099] -> w1117
            tunnel: w1119 -> [w1146 w1165 w1187 w1242 w1290 w1357 w1409 w1461 w1505 w1531 w1590 w1618 w1627 w1646 w1680 w1710 w1743 w1768 w1795 w1836 w1874 w1904 w1931 w1947 w1969 w1988 w2007 w2041 w2089 w2114 w2140 w2161 w2182 w2201 w2220 w2240 w2298 w2323 w2346 w2360 w2410 w2434 w2466 w2487 w2507 w2539 w2562 w2574 w2593 w2635 w2654 w2697 w2714 w2728 w2762 w2783 w2804 w2825 w2846 w2874 w2894 w2921 w2941 w2966 w2985 w3004 w3023 w3042 w3061 w3080 w3099]
            tunnel: w1118 -> [w1149 w1168 w1184 w1245 w1293 w1360 w1412 w1464 w1508 w1534 w1593 w1612 w1638 w1665 w1698 w1726 w1757 w1781 w1808 w1823 w1855 w1907 w1934 w1953 w1972 w1991 w2010 w2021 w2066 w2122 w2147 w2166 w2185 w2204 w2223 w2238 w2296 w2333 w2356 w2391 w2418 w2445 w2469 w2486 w2519 w2544 w2559 w2582 w2592 w2646 w2680 w2701 w2711 w2737 w2765 w2786 w2807 w2828 w2849 w2877 w2897 w2924 w2944 w2969 w2988 w3007 w3026 w3045 w3064 w3083 w3102]
            tunnel: w1112 -> [w1148 w1167 w1185 w1244 w1292 w1359 w1411 w1463 w1507 w1533 w1592 w1611 w1637 w1666 w1697 w1727 w1758 w1782 w1809 w1846 w1876 w1906 w1933 w1952 w1971 w1990 w2009 w2055 w2090 w2121 w2146 w2165 w2184 w2203 w2222 w2239 w2295 w2332 w2355 w2390 w2417 w2444 w2468 w2485 w2518 w2543 w2560 w2583 w2591 w2645 w2679 w2700 w2712 w2738 w2764 w2785 w2806 w2827 w2848 w2876 w2896 w2923 w2943 w2968 w2987 w3006 w3025 w3044 w3063 w3082 w3101]
            tunnel: w1111 -> [w1147 w1166 w1186 w1243 w1291 w1358 w1410 w1462 w1506 w1532 w1591 w1610 w1636 w1667 w1696 w1728 w1759 w1783 w1810 w1845 w1875 w1905 w1932 w1951 w1970 w1989 w2008 w2054 w2091 w2120 w2145 w2164 w2183 w2202 w2221 w2258 w2299 w2331 w2354 w2389 w2416 w2443 w2467 w2484 w2517 w2542 w2561 w2584 w2590 w2644 w2678 w2699 w2713 w2739 w2763 w2784 w2805 w2826 w2847 w2875 w2895 w2922 w2942 w2967 w2986 w3005 w3024 w3043 w3062 w3081 w3100]
            tunnel: [w1149 w1168 w1184 w1245 w1293 w1360 w1412 w1464 w1508 w1534 w1593 w1612 w1638 w1665 w1698 w1726 w1757 w1781 w1808 w1823 w1855 w1907 w1934 w1953 w1972 w1991 w2010 w2021 w2066 w2122 w2147 w2166 w2185 w2204 w2223 w2238 w2296 w2333 w2356 w2391 w2418 w2445 w2469 w2486 w2519 w2544 w2559 w2582 w2592 w2646 w2680 w2701 w2711 w2737 w2765 w2786 w2807 w2828 w2849 w2877 w2897 w2924 w2944 w2969 w2988 w3007 w3026 w3045 w3064 w3083 w3102] -> w1099
            tunnel: [w1148 w1167 w1185 w1244 w1292 w1359 w1411 w1463 w1507 w1533 w1592 w1611 w1637 w1666 w1697 w1727 w1758 w1782 w1809 w1846 w1876 w1906 w1933 w1952 w1971 w1990 w2009 w2055 w2090 w2121 w2146 w2165 w2184 w2203 w2222 w2239 w2295 w2332 w2355 w2390 w2417 w2444 w2468 w2485 w2518 w2543 w2560 w2583 w2591 w2645 w2679 w2700 w2712 w2738 w2764 w2785 w2806 w2827 w2848 w2876 w2896 w2923 w2943 w2968 w2987 w3006 w3025 w3044 w3063 w3082 w3101] -> w1098
            tunnel: [w1147 w1166 w1186 w1243 w1291 w1358 w1410 w1462 w1506 w1532 w1591 w1610 w1636 w1667 w1696 w1728 w1759 w1783 w1810 w1845 w1875 w1905 w1932 w1951 w1970 w1989 w2008 w2054 w2091 w2120 w2145 w2164 w2183 w2202 w2221 w2258 w2299 w2331 w2354 w2389 w2416 w2443 w2467 w2484 w2517 w2542 w2561 w2584 w2590 w2644 w2678 w2699 w2713 w2739 w2763 w2784 w2805 w2826 w2847 w2875 w2895 w2922 w2942 w2967 w2986 w3005 w3024 w3043 w3062 w3081 w3100] -> w1097
            tunnel: w1058 -> [w1145 w1164 w1183 w1209 w1266 w1334 w1408 w1460 w1504 w1529 w1550 w1617 w1626 w1663 w1669 w1711 w1738 w1765 w1794 w1835 w1860 w1898 w1930 w1948 w1968 w1987 w2006 w2025 w2086 w2113 w2144 w2162 w2181 w2200 w2219 w2249 w2276 w2315 w2351 w2362 w2415 w2435 w2465 w2483 w2508 w2541 w2558 w2571 w2595 w2615 w2652 w2696 w2715 w2740 w2759 w2780 w2801 w2822 w2833 w2863 w2882 w2906 w2938 w2955 w2975 w2994 w3013 w3032 w3051 w3070 w3089]
            tunnel: w1053 -> [w1144 w1163 w1182 w1240 w1288 w1354 w1406 w1458 w1502 w1522 w1586 w1616 w1635 w1662 w1677 w1709 w1745 w1771 w1798 w1838 w1873 w1897 w1928 w1950 w1967 w1986 w2005 w2043 w2088 w2111 w2139 w2163 w2180 w2199 w2218 w2251 w2297 w2329 w2353 w2383 w2411 w2436 w2463 w2482 w2510 w2538 w2557 w2581 w2598 w2614 w2671 w2695 w2716 w2741 w2758 w2779 w2800 w2821 w2834 w2871 w2891 w2902 w2937 w2963 w2982 w3001 w3020 w3039 w3058 w3077 w3096]
            tunnel: [w1145 w1164 w1183 w1209 w1266 w1333 w1408 w1460 w1504 w1529 w1572 w1601 w1626 w1651 w1669 w1711 w1738 w1764 w1793 w1839 w1859 w1899 w1929 w1948 w1968 w1987 w2006 w2050 w2085 w2112 w2142 w2162 w2181 w2200 w2219 w2252 w2271 w2330 w2350 w2384 w2414 w2437 w2464 w2483 w2511 w2540 w2558 w2570 w2594 w2615 w2650 w2696 w2715 w2740 w2759 w2780 w2801 w2822 w2833 w2863 w2882 w2906 w2938 w2955 w2975 w2994 w3013 w3032 w3051 w3070 w3089] -> w1094
            tunnel: [w1144 w1163 w1182 w1239 w1287 w1349 w1406 w1458 w1502 w1522 w1586 w1615 w1635 w1661 w1677 w1709 w1745 w1771 w1798 w1838 w1873 w1897 w1928 w1950 w1967 w1986 w2005 w2043 w2088 w2111 w2139 w2163 w2180 w2199 w2218 w2251 w2297 w2329 w2353 w2383 w2411 w2436 w2463 w2482 w2510 w2538 w2557 w2581 w2598 w2614 w2671 w2695 w2716 w2741 w2758 w2779 w2800 w2821 w2834 w2871 w2891 w2905 w2937 w2963 w2982 w3001 w3020 w3039 w3058 w3077 w3096] -> w1108
            tunnel: [_ _ _ _ _ _ _ _ _ _ _ _ _ _ _ _ _ _ _ _ _ _ _ _ _ _ _ _ _ _ _ _ _ _ _ _ _ _ w2344 _ _ _ _ _ _ _ _ _ _ _ _ _ _ _ _ _ _ _ _ _ _ _ _ _ _ _ _ _ _ _ _] -> w1069
            tunnel: [_ _ _ _ _ _ _ _ _ _ _ _ _ _ _ _ _ _ _ _ _ _ _ _ _ _ _ _ _ _ _ _ _ _ _ _ _ _ w2345 _ _ _ _ _ _ _ _ _ _ _ _ _ _ _ _ _ _ _ _ _ _ _ _ _ _ _ _ _ _ _ _] -> w1071
            tunnel: w1107 -> [w1142 w1161 w1180 w1211 w1268 w1355 w1407 w1459 w1503 w1527 w1587 w1613 w1628 w1659 w1689 w1724 w1755 w1761 w1790 w1837 w1872 w1894 w1924 w1949 w1965 w1984 w2003 w2049 w2087 w2110 w2137 w2159 w2178 w2197 w2216 w2250 w2293 w2321 w2352 w2364 w2408 w2433 w2461 w2480 w2509 w2537 w2555 w2573 w2600 w2642 w2663 w2693 w2718 w2743 w2756 w2777 w2798 w2819 w2843 w2857 w2884 w2912 w2931 w2957 w2976 w2995 w3014 w3033 w3052 w3071 w3090]
            tunnel: [w1142 w1161 w1180 w1211 w1268 w1355 w1407 w1459 w1503 w1527 w1587 w1613 w1625 w1659 w1689 w1724 w1755 w1761 w1790 w1837 w1872 w1894 w1924 w1949 w1965 w1984 w2003 w2049 w2087 w2110 w2137 w2159 w2178 w2197 w2216 w2250 w2293 w2321 w2352 w2363 w2408 w2433 w2461 w2480 w2509 w2537 w2555 w2572 w2600 w2642 w2663 w2693 w2718 w2743 w2756 w2777 w2798 w2819 w2843 w2857 w2884 w2912 w2931 w2957 w2976 w2995 w3014 w3033 w3052 w3071 w3090] -> w1106
            tunnel: w1105 -> [w1143 w1162 w1181 w1210 w1267 w1356 w1404 w1456 w1500 w1528 w1588 w1614 w1634 w1660 w1668 w1725 w1756 w1769 w1796 w1834 w1854 w1895 w1925 w1946 w1966 w1985 w2004 w2048 w2065 w2109 w2138 w2160 w2179 w2198 w2217 w2248 w2294 w2322 w2347 w2381 w2409 w2432 w2462 w2481 w2506 w2535 w2556 w2580 w2599 w2643 w2670 w2694 w2717 w2742 w2757 w2778 w2799 w2820 w2844 w2870 w2890 w2918 w2929 w2962 w2981 w3000 w3019 w3038 w3057 w3076 w3095]
            tunnel: [w1143 w1162 w1181 w1210 w1267 w1356 w1405 w1457 w1501 w1528 w1588 w1614 w1634 w1660 w1668 w1725 w1756 w1769 w1796 w1834 w1854 w1895 w1925 w1946 w1966 w1985 w2004 w2048 w2065 w2109 w2138 w2160 w2179 w2198 w2217 w2248 w2294 w2322 w2347 w2381 w2409 w2432 w2462 w2481 w2506 w2535 w2556 w2580 w2599 w2643 w2670 w2694 w2717 w2742 w2757 w2778 w2799 w2820 w2844 w2870 w2890 w2918 w2929 w2962 w2981 w3000 w3019 w3038 w3057 w3076 w3095] -> w1104
            tunnel: w1103 -> [_ _ _ _ _ _ _ _ _ _ _ _ _ _ _ _ _ _ _ w1819 w1847 w1880 w1913 _ _ _ _ _ w2059 w2096 _ _ _ _ _ _ _ _ _ _ _ _ _ _ _ w2536 _ _ _ _ _ _ _ _ _ _ _ _ _ _ _ _ _ _ _ _ _ _ _ _ _]
            tunnel: [_ _ _ _ _ _ _ _ _ _ _ _ _ _ _ _ _ _ _ _ _ _ _ _ _ _ _ _ _ _ _ _ _ _ _ _ _ _ _ _ _ _ _ _ _ _ _ _ _ _ _ TRUE _ _ _ _ _ _ _ _ _ _ _ _ _ _ _ _ _ _ _] -> w1100
            tunnel: w1090 -> [w1140 w1159 w1178 w1201 w1261 w1344 w1391 w1443 w1472 _ w1578 w1609 w1633 w1658 w1688 w1723 w1754 w1780 w1807 w1833 w1871 w1892 w1923 w1944 w1963 w1982 w2001 w2047 w2082 w2107 w2136 w2157 w2176 w2195 w2214 w2247 w2292 w2311 w2343 w2379 w2407 w2430 w2460 w2479 w2504 w2534 w2554 w2578 w2604 w2641 w2667 w2691 w2709 w2736 w2754 w2775 w2796 w2817 w2841 w2868 w2888 w2916 w2935 w2961 w2980 w2999 w3018 w3037 w3056 w3075 w3094]
            tunnel: w1089 -> [w1139 w1158 w1177 w1200 w1260 w1343 w1390 w1442 w1473 _ w1577 w1608 w1632 w1657 w1687 w1722 w1753 w1779 w1806 w1832 w1870 w1891 w1922 w1943 w1962 w1981 w2000 w2046 w2081 w2106 w2135 w2156 w2175 w2194 w2213 w2246 w2291 w2310 w2342 w2378 w2406 w2429 w2459 w2478 w2503 w2533 w2553 w2577 w2603 w2640 w2666 w2690 w2708 w2735 w2753 w2774 w2795 w2816 w2840 w2867 w2887 w2915 w2934 w2960 w2979 w2998 w3017 w3036 w3055 w3074 w3093]
            tunnel: w1088 -> [w1138 w1157 w1176 w1199 w1259 w1342 w1389 w1441 w1474 _ w1576 w1607 w1631 w1656 w1686 w1721 w1752 w1778 w1805 w1831 w1869 w1890 w1921 w1942 w1961 w1980 w1999 w2045 w2080 w2105 w2134 w2155 w2174 w2193 w2212 w2245 w2290 w2309 w2341 w2377 w2405 w2428 w2458 w2477 w2502 w2532 w2552 w2576 w2602 w2639 w2665 w2689 w2707 w2734 w2752 w2773 w2794 w2815 w2839 w2866 w2886 w2914 w2933 w2959 w2978 w2997 w3016 w3035 w3054 w3073 w3092]
            tunnel: w1087 -> [w1137 w1156 w1175 w1198 w1258 w1341 w1388 w1440 w1475 _ w1575 w1606 w1630 w1655 w1685 w1720 w1751 w1777 w1804 w1830 w1868 w1889 w1920 w1941 w1960 w1979 w1998 w2044 w2079 w2104 w2133 w2154 w2173 w2192 w2211 w2244 w2289 w2308 w2340 w2376 w2404 w2427 w2457 w2476 w2501 w2531 w2551 w2575 w2601 w2638 w2664 w2688 w2706 w2733 w2751 w2772 w2793 w2814 w2838 w2865 w2885 w2913 w2932 w2958 w2977 w2996 w3015 w3034 w3053 w3072 w3091]
            tunnel: w1086 -> [_ _ _ _ _ _ _ _ _ _ _ _ _ _ _ _ _ _ _ _ _ _ _ _ _ _ _ _ w2084 _ _ _ _ _ _ _ _ _ _ _ _ _ _ _ _ _ _ _ _ _ _ _ _ _ _ _ _ _ _ _ _ _ _ _ _ _ _ _ _ _ _]
            tunnel: w1085 -> [_ _ _ _ _ _ _ _ _ _ _ _ _ _ _ _ _ _ _ _ _ _ _ _ _ _ _ _ w2083 _ _ _ _ _ _ _ _ _ _ _ _ _ _ _ _ _ _ _ _ _ _ _ _ _ _ _ _ _ _ _ _ _ _ _ _ _ _ _ _ _ _]
            tunnel: [w1140 w1159 w1178 w1201 w1261 w1344 w1391 w1443 w1472 w1521 w1578 w1609 w1633 w1658 w1688 w1723 w1754 w1780 w1807 w1833 w1871 w1892 w1923 w1944 w1963 w1982 w2001 w2047 w2082 w2107 w2136 w2157 w2176 w2195 w2214 w2247 w2292 w2311 w2343 w2379 w2407 w2430 w2460 w2479 w2504 w2534 w2554 w2578 w2604 w2641 w2667 w2691 w2709 w2736 w2754 w2775 w2796 w2817 w2841 w2868 w2888 w2916 w2935 w2961 w2980 w2999 w3018 w3037 w3056 w3075 w3094] -> w1082
            tunnel: [w1139 w1158 w1177 w1200 w1260 w1343 w1390 w1442 w1473 w1512 w1577 w1608 w1632 w1657 w1687 w1722 w1753 w1779 w1806 w1832 w1870 w1891 w1922 w1943 w1962 w1981 w2000 w2046 w2081 w2106 w2135 w2156 w2175 w2194 w2213 w2246 w2291 w2310 w2342 w2378 w2406 w2429 w2459 w2478 w2503 w2533 w2553 w2577 w2603 w2640 w2666 w2690 w2708 w2735 w2753 w2774 w2795 w2816 w2840 w2867 w2887 w2915 w2934 w2960 w2979 w2998 w3017 w3036 w3055 w3074 w3093] -> w1050
            tunnel: [w1138 w1157 w1176 w1199 w1259 w1342 w1389 w1441 w1474 w1520 w1576 w1607 w1631 w1656 w1686 w1721 w1752 w1778 w1805 w1831 w1869 w1890 w1921 w1942 w1961 w1980 w1999 w2045 w2080 w2105 w2134 w2155 w2174 w2193 w2212 w2245 w2290 w2309 w2341 w2377 w2405 w2428 w2458 w2477 w2502 w2532 w2552 w2576 w2602 w2639 w2665 w2689 w2707 w2734 w2752 w2773 w2794 w2815 w2839 w2866 w2886 w2914 w2933 w2959 w2978 w2997 w3016 w3035 w3054 w3073 w3092] -> w1083
            tunnel: [w1137 w1156 w1175 w1198 w1258 w1341 w1388 w1440 w1475 w1510 w1575 w1606 w1630 w1655 w1685 w1720 w1751 w1777 w1804 w1830 w1868 w1889 w1920 w1941 w1960 w1979 w1998 w2044 w2079 w2104 w2133 w2154 w2173 w2192 w2211 w2244 w2289 w2308 w2340 w2376 w2404 w2427 w2457 w2476 w2501 w2531 w2551 w2575 w2601 w2638 w2664 w2688 w2706 w2733 w2751 w2772 w2793 w2814 w2838 w2865 w2885 w2913 w2932 w2958 w2977 w2996 w3015 w3034 w3053 w3072 w3091] -> w1084
            tunnel: [_ _ _ _ _ _ _ _ _ _ _ _ _ _ _ _ _ _ _ _ _ _ _ _ _ _ _ w2034 w2084 _ _ _ _ _ _ _ _ _ _ _ _ _ _ _ _ _ _ _ _ _ _ _ _ _ _ _ _ _ _ _ _ _ _ _ _ _ _ _ _ _ _] -> w1052
            tunnel: [_ _ _ _ _ _ _ _ _ _ _ _ _ _ _ _ _ _ _ _ _ _ _ _ _ _ _ w2033 w2083 _ _ _ _ _ _ _ _ _ _ _ _ _ _ _ _ _ _ _ _ _ _ _ _ _ _ _ _ _ _ _ _ _ _ _ _ _ _ _ _ _ _] -> w1051
            tunnel: w1065 -> [w1136 w1155 w1174 w1197 w1257 w1340 w1387 w1439 w1471 w1519 w1585 w1605 w1629 w1654 w1671 w1713 w1737 w1763 w1792 w1829 w1867 w1888 w1919 w1940 w1959 w1978 w1997 w2032 w2078 w2103 w2132 w2153 w2172 w2191 w2210 w2243 w2288 w2305 w2339 w2375 w2403 w2424 w2451 w2475 w2498 w2525 w2550 w2569 w2597 w2631 w2662 w2687 w2719 w2744 w2755 w2776 w2797 w2818 w2842 w2869 w2889 w2917 w2936 w2952 w2974 w2993 w3012 w3031 w3050 w3069 w3088]
            tunnel: [w1136 w1155 w1174 w1197 w1257 w1340 w1387 w1439 w1471 w1519 w1585 w1605 w1629 w1654 w1670 w1712 w1730 w1762 w1791 w1829 w1867 w1888 w1919 w1940 w1959 w1978 w1997 w2032 w2078 w2103 w2132 w2153 w2172 w2191 w2210 w2243 w2288 w2305 w2339 w2375 w2403 w2424 w2451 w2475 w2498 w2525 w2550 w2569 w2596 w2631 w2662 w2687 w2719 w2744 w2755 w2776 w2797 w2818 w2842 w2869 w2889 w2917 w2936 w2952 w2974 w2993 w3012 w3031 w3050 w3069 w3088] -> w1064
            tunnel: [w1135 w1154 w1173 w1196 w1256 w1339 w1386 w1438 w1470 w1518 w1584 w1604 w1640 w1653 w1691 w1719 w1750 w1776 w1803 w1828 w1866 w1887 w1918 w1939 w1958 w1977 w1996 w2031 w2077 w2102 w2131 w2152 w2171 w2190 w2209 w2242 w2287 w2304 w2338 w2374 w2402 w2423 w2450 w2474 w2497 w2524 w2549 w2568 w2589 w2637 w2661 w2685 w2720 w2730 w2750 w2771 w2792 w2813 w2837 w2873 w2893 w2920 w2940 w2965 w2984 w3003 w3022 w3041 w3060 w3079 w3098] -> w1063
            tunnel: [w1134 w1153 w1172 w1195 w1255 w1338 w1385 w1437 w1469 w1517 w1583 w1603 w1639 w1652 w1690 w1718 w1749 w1775 w1802 w1827 w1865 w1886 w1917 w1938 w1957 w1976 w1995 w2030 w2076 w2101 w2130 w2151 w2170 w2189 w2208 w2241 w2286 w2303 w2337 w2373 w2401 w2422 w2449 w2473 w2496 w2523 w2548 w2567 w2588 w2636 w2660 w2686 w2702 w2727 w2760 w2781 w2802 w2823 w2845 w2872 w2892 w2919 w2939 w2964 w2983 w3002 w3021 w3040 w3059 w3078 w3097] -> w1062
            tunnel: w1061 -> [w1135 w1154 w1173 w1196 w1256 w1339 w1386 w1438 w1470 w1518 w1584 w1604 w1640 w1653 w1691 w1719 w1750 w1776 w1803 w1828 w1866 w1887 w1918 w1939 w1958 w1977 w1996 w2031 w2077 w2102 w2131 w2152 w2171 w2190 w2209 w2242 w2287 w2304 w2338 w2374 w2402 w2423 w2450 w2474 w2497 w2524 w2549 w2568 w2589 w2637 w2661 w2685 _ w2730 w2750 w2771 w2792 w2813 w2837 w2873 w2893 w2920 w2940 w2965 w2984 w3003 w3022 w3041 w3060 w3079 w3098]
            tunnel: w1060 -> [w1134 w1153 w1172 w1195 w1255 w1338 w1385 w1437 w1469 w1517 w1583 w1603 w1639 w1652 w1690 w1718 w1749 w1775 w1802 w1827 w1865 w1886 w1917 w1938 w1957 w1976 w1995 w2030 w2076 w2101 w2130 w2151 w2170 w2189 w2208 w2241 w2286 w2303 w2337 w2373 w2401 w2422 w2449 w2473 w2496 w2523 w2548 w2567 w2588 w2636 w2660 w2686 _ w2727 w2760 w2781 w2802 w2823 w2845 w2872 w2892 w2919 w2939 w2964 w2983 w3002 w3021 w3040 w3059 w3078 w3097]
            tunnel: w1059 -> [_ _ _ _ _ _ _ _ _ _ _ _ _ _ _ _ _ _ _ _ _ _ _ _ _ _ _ _ _ _ _ _ _ _ _ _ _ _ _ _ _ _ _ _ _ _ _ _ _ _ _ _ _ _ w2748 w2769 w2790 w2811 w2835 _ _ _ _ _ _ _ _ _ _ _ _]
            tunnel: w1057 -> [_ _ _ _ _ _ _ _ _ _ _ _ _ _ _ _ w1742 _ w1787 w1816 w1852 w1878 w1909 _ _ _ _ w2012 w2057 w2095 w2124 _ _ _ _ _ _ _ _ _ _ _ _ _ _ _ _ _ _ _ _ _ _ _ _ _ _ _ _ _ _ _ _ _ _ _ _ _ _ _ _]
            tunnel: w1054 -> [_ _ _ _ _ _ _ _ _ _ _ _ _ _ _ _ _ _ _ _ _ _ _ _ _ _ _ _ _ _ _ _ _ _ _ _ _ _ _ _ _ _ _ _ _ _ _ _ _ _ _ _ _ _ _ _ _ _ _ _ _ w2907 _ _ _ _ _ _ _ _ _]
            tunnel: [w1133 w1152 w1171 w1194 w1254 w1337 w1384 w1436 w1468 w1516 w1582 w1599 w1623 w1649 w1692 w1717 w1748 w1774 w1801 w1826 w1864 w1885 w1916 w1937 w1956 w1975 w1994 w2029 w2075 w2100 w2129 w2150 w2169 w2188 w2207 w2237 w2285 w2302 w2336 w2358 w2400 w2421 w2448 w2472 w2495 w2522 w2547 w2566 w2587 w2634 w2647 w2684 w2705 w2729 w2747 w2768 w2789 w2810 w2832 w2852 w2881 w2901 w2928 w2948 w2973 w2992 w3011 w3030 w3049 w3068 w3087] -> w1048
            tunnel: w1049 -> [w1133 w1152 w1171 w1194 w1254 w1337 w1384 w1436 w1468 w1516 w1582 w1599 _ w1649 w1692 w1717 w1748 w1774 w1801 w1826 w1864 w1885 w1916 w1937 w1956 w1975 w1994 w2029 w2075 w2100 w2129 w2150 w2169 w2188 w2207 w2237 w2285 w2302 w2336 w2358 w2400 w2421 w2448 w2472 w2495 w2522 w2547 w2566 w2587 w2634 w2648 w2684 w2705 w2729 w2747 w2768 w2789 w2810 w2832 w2852 w2881 w2901 w2928 w2948 w2973 w2992 w3011 w3030 w3049 w3068 w3087]
            tunnel: w1047 -> [w1132 w1151 w1170 w1193 w1253 w1336 w1383 w1435 w1467 w1515 w1581 w1598 w1622 w1648 w1684 w1716 w1747 w1773 w1800 w1825 w1863 w1884 w1915 w1936 w1955 w1974 w1993 w2028 w2074 w2099 w2128 w2149 w2168 w2187 w2206 w2236 w2284 w2301 w2335 w2372 w2399 w2420 w2447 w2471 w2494 w2521 w2546 w2565 w2586 w2633 w2659 w2683 w2704 w2732 w2746 w2767 w2788 w2809 w2831 w2851 w2880 w2900 w2927 w2947 w2972 w2991 w3010 w3029 w3048 w3067 w3086]
            tunnel: w1046 -> [w1131 w1150 w1169 w1192 w1252 w1335 w1382 w1434 w1466 w1514 w1580 w1597 w1621 w1647 w1683 w1715 w1746 w1772 w1799 w1824 w1862 w1883 w1914 w1935 w1954 w1973 w1992 w2027 w2073 w2098 w2127 w2148 w2167 w2186 w2205 w2235 w2283 w2300 w2334 w2369 w2398 w2419 w2446 w2470 w2493 w2520 w2545 w2564 w2585 w2632 w2658 w2682 w2703 w2731 w2745 w2766 w2787 w2808 w2830 w2850 w2879 w2899 w2926 w2946 w2971 w2990 w3009 w3028 w3047 w3066 w3085]
            tunnel: [w1132 w1151 w1170 w1193 w1253 w1336 w1383 w1435 w1467 w1515 w1581 w1598 w1622 w1648 w1684 w1716 w1747 w1773 w1800 w1825 w1863 w1884 w1915 w1936 w1955 w1974 w1993 w2028 w2074 w2099 w2128 w2149 w2168 w2187 w2206 w2236 w2284 w2301 w2335 w2371 w2399 w2420 w2447 w2471 w2494 w2521 w2546 w2565 w2586 w2633 w2659 w2683 w2704 w2732 w2746 w2767 w2788 w2809 w2831 w2851 w2880 w2900 w2927 w2947 w2972 w2991 w3010 w3029 w3048 w3067 w3086] -> w1045
            tunnel: [w1131 w1150 w1169 w1192 w1252 w1335 w1382 w1434 w1466 w1514 w1580 w1597 w1621 w1647 w1683 w1715 w1746 w1772 w1799 w1824 w1862 w1883 w1914 w1935 w1954 w1973 w1992 w2027 w2073 w2098 w2127 w2148 w2167 w2186 w2205 w2235 w2283 w2300 w2334 w2370 w2398 w2419 w2446 w2470 w2493 w2520 w2545 w2564 w2585 w2632 w2658 w2682 w2703 w2731 w2745 w2766 w2787 w2808 w2830 w2850 w2879 w2899 w2926 w2946 w2971 w2990 w3009 w3028 w3047 w3066 w3085] -> w1044
            tunnel: w1043 -> [_ _ _ _ _ _ _ _ _ _ w1573 _ _ _ w1695 w1705 _ _ _ _ _ _ _ _ _ _ _ _ w2070 _ _ _ _ _ _ w2233 w2282 _ _ _ _ _ _ _ w2492 _ _ _ _ w2609 _ _ _ _ _ _ _ _ _ _ _ _ _ _ _ _ _ _ _ _ _]
            tunnel: w1042 -> [_ _ _ _ _ _ _ _ _ _ w1574 _ _ _ w1694 w1704 _ _ _ _ _ _ _ _ _ _ _ _ w2069 _ _ _ _ _ _ w2234 w2281 _ _ _ _ _ _ _ w2491 _ _ _ _ w2608 _ _ _ _ _ _ _ _ _ _ _ _ _ _ _ _ _ _ _ _ _]
            tunnel: w1040 -> [_ _ _ _ _ _ _ _ _ _ _ _ _ _ _ _ w1741 _ w1786 w1815 w1851 w1877 w1910 _ _ _ _ w2011 w2056 w2094 w2123 _ _ _ _ _ _ _ _ _ _ _ _ _ _ _ _ _ _ _ _ _ _ _ _ _ _ _ _ _ _ _ _ _ _ _ _ _ _ _ _]
            tunnel: [_ _ _ _ _ _ _ _ _ _ _ _ _ _ _ _ _ _ _ w1819 w1853 w1880 w1913 _ _ _ _ TRUE w2059 w2096 _ _ _ _ _ _ _ _ _ _ _ _ _ _ _ _ _ _ _ _ _ _ _ _ _ _ _ _ _ _ _ _ _ _ _ _ _ _ _ _ _] -> w1039
            tunnel: w1038 -> [_ _ _ _ _ _ _ _ _ _ _ _ _ _ _ _ w1740 _ _ w1818 w1857 w1882 w1911 _ _ _ _ w2019 w2064 w2093 w2126 _ _ _ _ _ _ _ _ _ _ _ _ _ _ _ _ _ _ _ _ _ _ _ _ _ _ _ _ _ _ _ _ _ _ _ _ _ _ _ _]
            tunnel: w1037 -> [_ _ _ _ _ _ _ _ _ _ _ _ _ _ _ _ w1739 _ _ w1817 w1856 w1881 w1912 _ _ _ _ w2018 w2063 w2092 w2125 _ _ _ _ _ _ _ _ _ _ _ _ _ _ _ _ _ _ _ _ _ _ _ _ _ _ _ _ _ _ _ _ _ _ _ _ _ _ _ _]
            tunnel: [_ _ _ _ _ _ _ _ _ _ _ _ _ _ _ _ w1740 _ w1789 w1818 w1857 w1882 w1911 _ _ _ _ w2019 w2064 w2093 w2126 _ _ _ _ _ _ _ _ _ _ _ _ _ _ _ _ _ _ _ _ _ _ _ _ _ _ _ _ _ _ _ _ _ _ _ _ _ _ _ _] -> w1036
            tunnel: [_ _ _ _ _ _ _ _ _ _ _ _ _ _ _ _ w1739 _ w1788 w1817 w1856 w1881 w1912 _ _ _ _ w2018 w2063 w2092 w2125 _ _ _ _ _ _ _ _ _ _ _ _ _ _ _ _ _ _ _ _ _ _ _ _ _ _ _ _ _ _ _ _ _ _ _ _ _ _ _ _] -> w1035
            tunnel: [_ _ _ _ _ _ _ _ _ _ _ _ _ _ _ _ w1742 w1766 w1787 w1816 w1852 w1878 w1909 _ _ _ _ w2012 w2057 w2095 w2124 _ _ _ _ _ _ _ _ _ _ _ _ _ _ _ _ _ _ _ _ _ _ _ _ _ _ _ _ _ _ _ _ _ _ _ _ _ _ _ _] -> w1034
            tunnel: [_ _ _ _ _ _ _ _ _ _ _ _ _ _ _ _ w1741 w1767 w1786 w1815 w1851 w1877 w1910 _ _ _ _ w2011 w2056 w2094 w2123 _ _ _ _ _ _ _ _ _ _ _ _ _ _ _ _ _ _ _ _ _ _ _ _ _ _ _ _ _ _ _ _ _ _ _ _ _ _ _ _] -> w1033
            tunnel: [_ _ _ _ _ _ _ _ _ _ _ _ _ _ _ _ _ _ _ _ w1850 _ _ _ _ _ _ _ w2061 _ _ _ _ _ _ _ _ _ _ _ _ _ _ _ _ _ _ _ _ _ _ _ _ _ _ _ _ _ _ _ _ _ _ _ _ _ _ _ _ _ _] -> w1030
            tunnel: [_ _ _ _ _ _ _ _ _ _ _ _ _ _ _ _ _ _ _ _ w1849 _ _ _ _ _ _ _ w2062 _ _ _ _ _ _ _ _ _ _ _ _ _ _ _ _ _ _ _ _ _ _ _ _ _ _ _ _ _ _ _ _ _ _ _ _ _ _ _ _ _ _] -> w1032
            tunnel: w1027 -> [_ _ _ _ _ _ _ _ _ _ _ _ _ _ _ _ _ _ _ w1814 w1848 w1879 w1908 _ _ _ _ w2014 w2058 w2097 _ _ _ _ _ _ _ _ _ _ _ _ _ _ _ _ _ _ _ _ _ _ _ _ _ _ _ _ _ _ _ _ _ _ _ _ _ _ _ _ _]
            tunnel: [_ _ _ _ _ _ _ _ _ _ _ _ _ _ _ _ _ _ _ w1814 w1848 w1879 w1908 _ _ _ _ w2014 w2060 w2097 _ _ _ _ _ _ _ _ _ _ _ _ _ _ _ _ _ _ _ _ _ _ _ _ _ _ _ _ _ _ _ _ _ _ _ _ _ _ _ _ _] -> w1026
            tunnel: [_ _ _ _ _ _ _ _ _ _ _ _ _ _ _ _ _ w1760 w1785 _ _ _ _ _ _ _ _ _ _ _ _ _ _ _ _ _ _ _ _ _ _ _ _ _ _ _ _ _ _ _ _ _ _ _ _ _ _ _ _ _ _ _ _ _ _ _ _ _ _ _ _] -> w1025
            tunnel: [_ _ _ _ _ _ _ _ _ _ _ _ _ _ _ _ _ _ TRUE ("Recording") _ _ _ _ _ _ _ _ _ _ _ _ _ _ _ _ _ _ _ _ _ _ _ _ _ _ _ _ _ _ _ _ _ _ _ _ _ _ _ _ _ _ _ _ _ _ _ _ _ _ _ _] -> w1022
            tunnel: [_ _ _ _ _ _ _ _ _ _ _ _ _ _ _ _ _ w1760 _ _ _ _ _ _ _ _ _ _ _ _ _ _ _ _ _ _ _ _ _ _ _ _ _ _ _ _ _ _ _ _ _ _ _ _ _ _ _ _ _ _ _ _ _ _ _ _ _ _ _ _ _] -> w1016
            tunnel: [_ _ _ _ _ _ _ _ _ _ _ TRUE _ _ _ _ _ _ _ _ _ _ _ _ _ _ _ _ _ _ _ _ _ _ _ _ _ _ _ _ _ _ _ _ _ _ _ _ _ _ _ _ _ _ _ _ _ _ _ _ _ _ _ _ _ _ _ _ _ _ _] -> w1012
            tunnel: [_ _ _ _ _ _ _ _ _ _ _ w1594 _ _ _ _ _ _ _ _ _ _ _ _ _ _ _ _ _ _ _ _ _ _ _ _ _ _ _ _ _ _ _ _ _ _ _ _ _ _ _ _ _ _ _ _ _ _ _ _ _ _ _ _ _ _ _ _ _ _ _] -> w1010
            tunnel: [_ _ _ _ _ _ _ _ _ _ _ _ _ TRUE _ _ _ _ _ _ _ _ _ _ _ _ _ _ _ _ _ _ _ _ _ _ _ _ _ _ _ _ _ _ _ _ _ _ _ _ _ _ _ _ _ _ _ _ _ _ _ _ _ _ _ _ _ _ _ _ _] -> w1009
            tunnel: [_ _ _ _ _ _ _ _ _ _ _ _ _ w1641 _ _ _ _ _ _ _ _ _ _ _ _ _ _ _ _ _ _ _ _ _ _ _ _ _ _ _ _ _ _ _ _ _ _ _ _ _ _ _ _ _ _ _ _ _ _ _ _ _ _ _ _ _ _ _ _ _] -> w1008
            frame "Start1", Default {
            }
            frame "Start2" {
            }
            frame "Start3" {
            }
            frame "saveSettings1" {
              n597 = call "myRIO_BRig_RT_dataExp_Audio_freq__L.vi"() -> ("output_Audio_freq__L"=w1217:i32)  [unwired: 11 in]
              n598 = call "myRIO_BRig_RT_dataExp_Audio_freq__R.vi"() -> ("output_Audio_freq__R"=w1216:i32)  [unwired: 11 in]
              n599 = call "myRIO_BRig_RT_dataExp_Audio_amp__L.vi"() -> ("output_Audio_amp__L"=w1215:i32)  [unwired: 11 in]
              n600 = call "myRIO_BRig_RT_dataExp_Audio_amp__R.vi"() -> ("output_Audio_amp__R"=w1213:i32)  [unwired: 11 in]
              n601 = call "myRIO_BRig_RT_dataExp_TPB_min__L.vi"() -> ("output_TPB_min__L"=w1225:i32)  [unwired: 11 in]
              n602 = call "myRIO_BRig_RT_dataExp_TPB_min__R.vi"() -> ("output_TPB_min__R"=w1223:i32)  [unwired: 11 in]
              n603 = call "myRIO_BRig_RT_dataExp_TPB_max__L.vi"() -> ("output_TPB_max__L"=w1221:i32)  [unwired: 11 in]
              n604 = call "myRIO_BRig_RT_dataExp_TPB_max__R.vi"() -> ("output_TPB_max__R"=w1219:i32)  [unwired: 11 in]
              n605 = call "myRIO_BRig_RT_dataExp_ItrialUntilReward.vi"() -> ("output_I_trialUntilReward"=w1238:i32)  [unwired: 11 in]
              n606 = call "myRIO_BRig_RT_dataExp_IblockUntilReward.vi"() -> ("output_I_blockUntilReward"=w1234:i32)  [unwired: 11 in]
              n607 = call "myRIO_BRig_RT_dataExp_CueCycles.vi"() -> ("output_CueCycles"=w1233:i32)  [unwired: 11 in]
              n608 = call "myRIO_BRig_RT_dataExp_ENL_min.vi"() -> ("output_ENL_min"=w1231:i32)  [unwired: 11 in]
              n609 = call "myRIO_BRig_RT_dataExp_ENL_max.vi"() -> ("output_ENL_max"=w1229:i32)  [unwired: 11 in]
              n610 = call "myRIO_BRig_RT_dataExp_ENL_penalty.vi"() -> ("output_ENL_penalty"=w1227:i32)  [unwired: 11 in]
              n611 = local read "Audio_Freq__L"() -> (w1191:u8)
              n612 = local read "Audio_Freq__R"() -> (w1189:u8)
              n613 = local read "Audio_Amp__L"() -> (w1214:u16)
              n614 = local read "TpB_Min_L"() -> (w1224:u16)
              n615 = local read "TpB_Min_R"() -> (w1222:u16)
              n616 = local read "TpB_Max_L"() -> (w1220:u16)
              n617 = local read "TpB_Max_R"() -> (w1218:u16)
              n618 = local read "Audio_Amp__R"() -> (w1212:u16)
              n619 = local read "TrialUntilReward"() -> (w1237:bool)
              n620 = local read "CueCycles"() -> (w1232:u16)
              n621 = local read "Tcycle_ENL_min"() -> (w1230:u16)
              n622 = local read "Tcycle_ENL_max"() -> (w1228:u16)
              n623 = local read "Tcycle_ENLPenalty"() -> (w1226:u16)
              n624 = To Unsigned Word Integer(number=w1189) -> (unsigned 16bit integer=w1188:u16)
              n625 = To Unsigned Word Integer(number=w1191) -> (unsigned 16bit integer=w1190:u16)
              n626 = Boolean To (0,1)(Boolean=w1237) -> (0, 1=w1236:i16)
              n627 = To Unsigned Word Integer(number=w1236) -> (unsigned 16bit integer=w1235:u16)
              n628 = local read "BUR_min"() -> (w1206:u16)
              n629 = local read "BUR_max"() -> (w1207:u16)
              n630 = Not Equal To 0?(x=w1206) -> (x != 0?=w1205:bool)
              n631 = Not Equal To 0?(x=w1207) -> (x != 0?=w1204:bool)
              n632 = And(x=w1205, y=w1204) -> (x .and. y?=w1203:bool)
              n633 = Boolean To (0,1)(Boolean=w1203) -> (0, 1=w1208:i16)
              n634 = To Unsigned Word Integer(number=w1208) -> (unsigned 16bit integer=w1202:u16)
              n635 = Replace Array Subset(array=w1240, new element #1=w1235, index #1=w1238, new element #2=w1202, index #2=w1234, new element #3=w1232, index #3=w1233, new element #4=w1230, index #4=w1231, new element #5=w1228, index #5=w1229, new element #6=w1226, index #6=w1227, new element #7=w1224, index #7=w1225, new element #8=w1222, index #8=w1223, new element #9=w1220, index #9=w1221, new element #10=w1218, index #10=w1219, new element #11=w1190, index #11=w1217, new element #12=w1188, index #12=w1216, new element #13=w1214, index #13=w1215, new element #14=w1212, index #14=w1213) -> (w1239:u16[])
            }
            frame "saveSettings2" {
              n636 = call "myRIO_BRig_RT_dataExp_Tcycle_RewardPost.vi"() -> ("output_Tcycle_RewardPost"=w1277:i32)  [unwired: 11 in]
              n637 = call "myRIO_BRig_RT_dataExp_Tcycle_Wrong.vi"() -> ("output_Tcycle_Wrong"=w1275:i32)  [unwired: 11 in]
              n638 = call "myRIO_BRig_RT_dataExp_Tcycle_Timeout.vi"() -> ("output_Tcycle_Timeout"=w1273:i32)  [unwired: 11 in]
              n639 = call "myRIO_BRig_RT_dataExp_Tcycle_Cue_min.vi"() -> ("output_Tcycle_Cue_min"=w1271:i32)  [unwired: 11 in]
              n640 = call "myRIO_BRig_RT_dataExp_Tcycle_Cue_max.vi"() -> ("output_Tcycle_Cue_max"=w1270:i32)  [unwired: 11 in]
              n641 = call "myRIO_BRig_RT_dataExp_Tcycle_CuePenalty.vi"() -> ("output_Tcycle_CuePenalty"=w1269:i32)  [unwired: 11 in]
              n642 = call "myRIO_BRig_RT_dataExp_SolenoidProbability_L.vi"() -> ("output_SolenoidProbability_L"=w1249:i32)  [unwired: 11 in]
              n643 = call "myRIO_BRig_RT_dataExp_SolenoidProbability_R.vi"() -> ("output_SolenoidProbability_R"=w1248:i32)  [unwired: 11 in]
              n644 = call "myRIO_BRig_RT_dataExp_nBlock.vi"() -> ("output_nBlock"=w1286:i32)  [unwired: 11 in]
              n645 = call "myRIO_BRig_RT_dataExp_nTrial.vi"() -> ("output_nTrial"=w1285:i32)  [unwired: 11 in]
              n646 = call "myRIO_BRig_RT_dataExp_runTime_seconds.vi"() -> ("output_RunTime_minutes"=w1284:i32)  [unwired: 11 in]
              n647 = call "myRIO_BRig_RT_dataExp_Tcycle_Selection.vi"() -> ("output_Tcycle_Selection"=w1283:i32)  [unwired: 11 in]
              n648 = call "myRIO_BRig_RT_dataExp_Tcycle_Reward__L.vi"() -> ("output_Tcycle_Reward__L"=w1281:i32)  [unwired: 11 in]
              n649 = call "myRIO_BRig_RT_dataExp_Tcycle_Reward__R.vi"() -> ("output_Tcycle_Reward__R"=w1279:i32)  [unwired: 11 in]
              n650 = local read "Tcycle_RewardPost"() -> (w1276:u16)
              n651 = local read "Tcycle_Wrong"() -> (w1274:u16)
              n652 = local read "Tcycle_Timeout"() -> (w1272:u16)
              n653 = local read "Tcycle_CuePenalty"() -> (w1262:u16)
              n654 = local read "Tcycle_Cue_max"() -> (w1250:u16)
              n655 = local read "Tcycle_Cue_min"() -> (w1251:u16)
              n656 = local read "Tcycle_Selection"() -> (w1282:u16)
              n657 = local read "Tcycle_Reward_L"() -> (w1280:u16)
              n658 = local read "Tcycle_Reward_R"() -> (w1278:u16)
              n659 = local read "SolenoidProbability_R"() -> (w1246:u16)
              n660 = local read "SolenoidProbability_L"() -> (w1247:u16)
              n661 = Replace Array Subset(array=w1288, new element #1=u16 0, index #1=w1286, new element #2=u16 0, index #2=w1285, new element #3=u16 0, index #3=w1284, new element #4=w1282, index #4=w1283, new element #5=w1280, index #5=w1281, new element #6=w1278, index #6=w1279, new element #7=w1276, index #7=w1277, new element #8=w1274, index #8=w1275, new element #9=w1272, index #9=w1273, new element #10=w1251, index #10=w1271, new element #11=w1250, index #11=w1270, new element #12=w1262, index #12=w1269, new element #13=w1247, index #13=w1249, new element #14=w1246, index #14=w1248) -> (w1287:u16[])
            }
            frame "saveSettings3" {
              w1298 = 100.0 ("y")
              n662 = call "myRIO_BRig_RT_dataExp_laser_Freq.vi"() -> ("output_laser_Freq"=w1331:i32)  [unwired: 11 in]
              n663 = call "myRIO_BRig_RT_dataExp_laser_Tpeak.vi"() -> ("output_laser_Tpeak"=w1326:i32)  [unwired: 11 in]
              n664 = call "myRIO_BRig_RT_dataExp_laser_Tshutter.vi"() -> ("output_laser_Tshutter"=w1321:i32)  [unwired: 11 in]
              n665 = call "myRIO_BRig_RT_dataExp_laser_f_millisec2count.vi"() -> ("output_laser_f_millisec2count"=w1316:i32)  [unwired: 11 in]
              n666 = call "myRIO_BRig_RT_dataExp_laser_Power_min.vi"() -> ("output_laser_Power_min"=w1311:i32)  [unwired: 11 in]
              n667 = call "myRIO_BRig_RT_dataExp_laser_Power_max.vi"() -> ("output_laser_Power_max"=w1304:i32)  [unwired: 11 in]
              n668 = call "myRIO_BRig_RT_dataExp_laser_Power_step.vi"() -> ("output_laser_Power_step"=w1303:i32)  [unwired: 11 in]
              n669 = call "myRIO_BRig_RT_dataExp_laser_duration.vi"() -> ("output_laser_duration"=w1306:i32)  [unwired: 11 in]
              n670 = call "myRIO_BRig_RT_dataExp_BUR_min.vi"() -> ("output_BUR_min"=w1353:i32)  [unwired: 11 in]
              n671 = call "myRIO_BRig_RT_dataExp_BUR_max.vi"() -> ("output_BUR_max"=w1351:i32)  [unwired: 11 in]
              n672 = call "myRIO_BRig_RT_dataExp_Audio_sp__L.vi"() -> ("output_Audio_sp__L"=w1348:i32)  [unwired: 11 in]
              n673 = call "myRIO_BRig_RT_dataExp_Audio_sp__R.vi"() -> ("output_Audio_sp__R"=w1347:i32)  [unwired: 11 in]
              n674 = local read "laser_Tshutter"() -> (w1318:dbl)
              n675 = local read "f_millisec2count"() -> (w1313:dbl)
              n676 = local read "laser_Tpeak"() -> (w1323:dbl)
              n677 = local read "laser_power_min"() -> (w1308:dbl)
              n678 = local read "laser_power_max"() -> (w1297:dbl)
              n679 = local read "laser_power_step"() -> (w1296:dbl)
              n680 = local read "laser_Freq"() -> (w1330:dbl)
              n681 = local read "sp_LeftSpout"() -> (w1346:u16)
              n682 = local read "BUR_max"() -> (w1350:u16)
              n683 = local read "sp_RightSpout"() -> (w1345:u16)
              n684 = local read "BUR_min"() -> (w1352:u16)
              n685 = Multiply(x=w1330, y=w1298) -> (x*y=w1329:dbl)
              n686 = Multiply(x=w1323, y=w1298) -> (x*y=w1325:dbl)
              n687 = Multiply(x=w1318, y=w1298) -> (x*y=w1320:dbl)
              n688 = Multiply(x=w1313, y=w1298) -> (x*y=w1315:dbl)
              n689 = Multiply(x=w1308, y=w1298) -> (x*y=w1310:dbl)
              n690 = Multiply(x=w1297, y=w1298) -> (x*y=w1302:dbl)
              n691 = Multiply(x=w1296, y=w1298) -> (x*y=w1300:dbl)
              n692 = Round To Nearest(number=w1329) -> (nearest integer value=w1328:dbl)
              n693 = Round To Nearest(number=w1325) -> (nearest integer value=w1324:dbl)
              n694 = Round To Nearest(number=w1320) -> (nearest integer value=w1319:dbl)
              n695 = Round To Nearest(number=w1315) -> (nearest integer value=w1314:dbl)
              n696 = Round To Nearest(number=w1310) -> (nearest integer value=w1309:dbl)
              n697 = Round To Nearest(number=w1302) -> (nearest integer value=w1301:dbl)
              n698 = Round To Nearest(number=w1300) -> (nearest integer value=w1299:dbl)
              n699 = To Unsigned Word Integer(number=w1328) -> (unsigned 16bit integer=w1327:u16)
              n700 = To Unsigned Word Integer(number=w1324) -> (unsigned 16bit integer=w1322:u16)
              n701 = To Unsigned Word Integer(number=w1319) -> (unsigned 16bit integer=w1317:u16)
              n702 = To Unsigned Word Integer(number=w1314) -> (unsigned 16bit integer=w1312:u16)
              n703 = To Unsigned Word Integer(number=w1309) -> (unsigned 16bit integer=w1307:u16)
              n704 = To Unsigned Word Integer(number=w1301) -> (unsigned 16bit integer=w1295:u16)
              n705 = To Unsigned Word Integer(number=w1299) -> (unsigned 16bit integer=w1294:u16)
              n706 = local read "laser_duration"() -> (w1305:u16)
              n707 = call "myRIO_BRig_RT_dataCurrent_LaserPulse_duration.vi"() -> ("output_LaserPulse_duration"=w1332:i32)  [unwired: 11 in]
              n708 = Replace Array Subset(array=w1354, new element #1=w1352, index #1=w1353, new element #2=w1350, index #2=w1351, new element #3=w1346, index #3=w1348, new element #4=w1345, index #4=w1347, new element #5=w1327, index #5=w1331, new element #6=w1322, index #6=w1326, new element #7=w1317, index #7=w1321, new element #8=w1312, index #8=w1316, new element #9=w1307, index #9=w1311, new element #10=w1295, index #10=w1304, new element #11=w1294, index #11=w1303, new element #12=w1305, index #12=w1306) -> (w1349:u16[])
              n709 = Replace Array Subset(array=w1334, new element=w1305, index=w1332) -> (w1333:u16[])
            }
            frame "saveSettings4_LC_ENL" {
              # "delayOpt"
              # "Count"
              # "Tdelay"
              # "Probability"
              # "OnOff"
              # "Block"
              # "ENL1 All"
              # "delayOpt"
              # "Count"
              # "Tdelay"
              # "Probability"
              # "OnOff"
              # "Block"
              # "ENL1 First"
              n710 = call "myRIO_BRig_RT_dataLC_ENL1_All_Block.vi"() -> ("output_ENL1_All_Block"=w1377:i32)  [unwired: 11 in]
              n711 = call "myRIO_BRig_RT_dataLC_ENL1_All_OnOff.vi"() -> ("output_ENL1_All_OnOff"=w1366:i32)  [unwired: 11 in]
              n712 = call "myRIO_BRig_RT_dataLC_ENL1_All_Probability.vi"() -> ("output_ENL1_All_Probability"=w1365:i32)  [unwired: 11 in]
              n713 = call "myRIO_BRig_RT_dataLC_ENL1_All_Tdelay.vi"() -> ("output_ENL1_All_Tdelay"=w1364:i32)  [unwired: 11 in]
              n714 = call "myRIO_BRig_RT_dataLC_ENL1_All_Count.vi"() -> ("output_ENL1_All_Count"=w1363:i32)  [unwired: 11 in]
              n715 = call "myRIO_BRig_RT_dataLC_ENL1_All_delayOpt.vi"() -> ("output_ENL1_All_delayOpt"=w1362:i32)  [unwired: 11 in]
              n716 = call "myRIO_BRig_RT_dataLC_ENL1_First_Block.vi"() -> ("output_ENL1_First_Block"=w1403:i32)  [unwired: 11 in]
              n717 = call "myRIO_BRig_RT_dataLC_ENL1_First_OnOff.vi"() -> ("output_ENL1_First_OnOff"=w1401:i32)  [unwired: 11 in]
              n718 = call "myRIO_BRig_RT_dataLC_ENL1_First_Probability.vi"() -> ("output_ENL1_First_Probability"=w1397:i32)  [unwired: 11 in]
              n719 = call "myRIO_BRig_RT_dataLC_ENL1_First_Tdelay.vi"() -> ("output_ENL1_First_Tdelay"=w1395:i32)  [unwired: 11 in]
              n720 = call "myRIO_BRig_RT_dataLC_ENL1_First_Count.vi"() -> ("output_ENL1_First_Count"=w1393:i32)  [unwired: 11 in]
              n721 = call "myRIO_BRig_RT_dataLC_ENL1_First_delayOpt.vi"() -> ("output_ENL1_First_delayOpt"=w1379:i32)  [unwired: 11 in]
              n722 = local read "LC_ENL1_First_delayOpt"() -> (w1380:bool)
              n723 = local read "LC_ENL1_First_Count"() -> (w1392:u16)
              n724 = local read "LC_ENL1_First_Probability"() -> (w1396:u16)
              n725 = local read "LC_ENL1_First_Block"() -> (w1402:u16)
              n726 = local read "LC_ENL1_First_Tdelay"() -> (w1394:u16)
              n727 = local read "LC_ENL1_First_OnOff"() -> (w1400:bool)
              n728 = local read "LC_ENL1_All_OnOff"() -> (w1373:bool)
              n729 = local read "LC_ENL1_All_Probability"() -> (w1371:u16)
              n730 = local read "LC_ENL1_All_delayOpt"() -> (w1368:bool)
              n731 = local read "LC_ENL1_All_Tdelay"() -> (w1370:u16)
              n732 = local read "LC_ENL1_All_Block"() -> (w1374:u16)
              n733 = local read "LC_ENL1_All_Count"() -> (w1369:u16)
              n734 = Boolean To (0,1)(Boolean=w1380) -> (0, 1=w1381:i16)
              n735 = Boolean To (0,1)(Boolean=w1400) -> (0, 1=w1399:i16)
              n736 = Boolean To (0,1)(Boolean=w1373) -> (0, 1=w1376:i16)
              n737 = To Unsigned Word Integer(number=w1381) -> (unsigned 16bit integer=w1378:u16)
              n738 = To Unsigned Word Integer(number=w1399) -> (unsigned 16bit integer=w1398:u16)
              n739 = Boolean To (0,1)(Boolean=w1368) -> (0, 1=w1375:i16)
              n740 = To Unsigned Word Integer(number=w1376) -> (unsigned 16bit integer=w1372:u16)
              n741 = To Unsigned Word Integer(number=w1375) -> (unsigned 16bit integer=w1367:u16)
              n742 = Replace Array Subset(array=w1404, new element #1=w1402, index #1=w1403, new element #2=w1398, index #2=w1401, new element #3=w1396, index #3=w1397, new element #4=w1394, index #4=w1395, new element #5=w1392, index #5=w1393, new element #6=w1378, index #6=w1379, new element #7=w1374, index #7=w1377, new element #8=w1372, index #8=w1366, new element #9=w1371, index #9=w1365, new element #10=w1370, index #10=w1364, new element #11=w1369, index #11=w1363, new element #12=w1367, index #12=w1362) -> (w1405:u16[])
            }
            frame "saveSettings5_LC_Cue" {
              # "delayOpt"
              # "Count"
              # "Tdelay"
              # "Probability"
              # "OnOff"
              # "Block"
              # "Cue1 All"
              # "delayOpt"
              # "Count"
              # "Tdelay"
              # "Probability"
              # "OnOff"
              # "Block"
              # "Cue1 First"
              n743 = call "myRIO_BRig_RT_dataLC_Cue1_First_delayOpt.vi"() -> ("output_Cue1_First_delayOpt"=w1432:i32)  [unwired: 11 in]
              n744 = call "myRIO_BRig_RT_dataLC_Cue1_First_Block.vi"() -> ("output_Cue1_First_Block"=w1455:i32)  [unwired: 11 in]
              n745 = call "myRIO_BRig_RT_dataLC_Cue1_First_OnOff.vi"() -> ("output_Cue1_First_OnOff"=w1453:i32)  [unwired: 11 in]
              n746 = call "myRIO_BRig_RT_dataLC_Cue1_First_Probability.vi"() -> ("output_Cue1_First_Probability"=w1449:i32)  [unwired: 11 in]
              n747 = call "myRIO_BRig_RT_dataLC_Cue1_First_Tdelay.vi"() -> ("output_Cue1_First_Tdelay"=w1447:i32)  [unwired: 11 in]
              n748 = call "myRIO_BRig_RT_dataLC_Cue1_First_Count.vi"() -> ("output_Cue1_First_Count"=w1445:i32)  [unwired: 11 in]
              n749 = call "myRIO_BRig_RT_dataLC_Cue1_All_Block.vi"() -> ("output_Cue1_All_Block"=w1429:i32)  [unwired: 11 in]
              n750 = call "myRIO_BRig_RT_dataLC_Cue1_All_OnOff.vi"() -> ("output_Cue1_All_OnOff"=w1428:i32)  [unwired: 11 in]
              n751 = call "myRIO_BRig_RT_dataLC_Cue1_All_Probability.vi"() -> ("output_Cue1_All_Probability"=w1427:i32)  [unwired: 11 in]
              n752 = call "myRIO_BRig_RT_dataLC_Cue1_All_Tdelay.vi"() -> ("output_Cue1_All_Tdelay"=w1426:i32)  [unwired: 11 in]
              n753 = call "myRIO_BRig_RT_dataLC_Cue1_All_Count.vi"() -> ("output_Cue1_All_Count"=w1425:i32)  [unwired: 11 in]
              n754 = call "myRIO_BRig_RT_dataLC_Cue1_All_delayOpt.vi"() -> ("output_Cue1_All_delayOpt"=w1424:i32)  [unwired: 11 in]
              n755 = local read "LC_Cue1_First_delayOpt"() -> (w1431:bool)
              n756 = local read "LC_Cue1_First_Count"() -> (w1444:u16)
              n757 = local read "LC_Cue1_First_Probability"() -> (w1448:u16)
              n758 = local read "LC_Cue1_First_Block"() -> (w1454:u16)
              n759 = local read "LC_Cue1_First_Tdelay"() -> (w1446:u16)
              n760 = local read "LC_Cue1_First_OnOff"() -> (w1452:bool)
              n761 = local read "LC_Cue1_All_OnOff"() -> (w1420:bool)
              n762 = local read "LC_Cue1_All_delayOpt"() -> (w1421:bool)
              n763 = local read "LC_Cue1_All_Probability"() -> (w1417:u16)
              n764 = local read "LC_Cue1_All_Tdelay"() -> (w1416:u16)
              n765 = local read "LC_Cue1_All_Count"() -> (w1415:u16)
              n766 = local read "LC_Cue1_All_Block"() -> (w1419:u16)
              n767 = Boolean To (0,1)(Boolean=w1431) -> (0, 1=w1433:i16)
              n768 = Boolean To (0,1)(Boolean=w1452) -> (0, 1=w1451:i16)
              n769 = Boolean To (0,1)(Boolean=w1420) -> (0, 1=w1423:i16)
              n770 = To Unsigned Word Integer(number=w1433) -> (unsigned 16bit integer=w1430:u16)
              n771 = To Unsigned Word Integer(number=w1451) -> (unsigned 16bit integer=w1450:u16)
              n772 = To Unsigned Word Integer(number=w1423) -> (unsigned 16bit integer=w1418:u16)
              n773 = Boolean To (0,1)(Boolean=w1421) -> (0, 1=w1422:i16)
              n774 = To Unsigned Word Integer(number=w1422) -> (unsigned 16bit integer=w1414:u16)
              n775 = Replace Array Subset(array=w1456, new element #1=w1454, index #1=w1455, new element #2=w1450, index #2=w1453, new element #3=w1448, index #3=w1449, new element #4=w1446, index #4=w1447, new element #5=w1444, index #5=w1445, new element #6=w1430, index #6=w1432, new element #7=w1419, index #7=w1429, new element #8=w1418, index #8=w1428, new element #9=w1417, index #9=w1427, new element #10=w1416, index #10=w1426, new element #11=w1415, index #11=w1425, new element #12=w1414, index #12=w1424) -> (w1457:u16[])
            }
            frame "saveSettings6_LC_Other" {
              # "Trial"
              # "Tdelay"
              # "Probability"
              # "OnOff"
              # "Block"
              # "Wrong"
              # "Trial"
              # "Tdelay"
              # "Probability"
              # "OnOff"
              # "Block"
              # "Reward"
              n776 = call "myRIO_BRig_RT_dataLC_Wrong_Block.vi"() -> ("output_Wrong_Block"=w1487:i32)  [unwired: 11 in]
              n777 = call "myRIO_BRig_RT_dataLC_Wrong_OnOff.vi"() -> ("output_Wrong_OnOff"=w1486:i32)  [unwired: 11 in]
              n778 = call "myRIO_BRig_RT_dataLC_Wrong_Probability.vi"() -> ("output_Wrong_Probability"=w1485:i32)  [unwired: 11 in]
              n779 = call "myRIO_BRig_RT_dataLC_Wrong_Tdelay.vi"() -> ("output_Wrong_Tdelay"=w1484:i32)  [unwired: 11 in]
              n780 = call "myRIO_BRig_RT_dataLC_Wrong_Trial.vi"() -> ("output_Wrong_Trial"=w1483:i32)  [unwired: 11 in]
              n781 = call "myRIO_BRig_RT_dataLC_Reward_Block.vi"() -> ("output_Reward_Block"=w1499:i32)  [unwired: 11 in]
              n782 = call "myRIO_BRig_RT_dataLC_Reward_OnOff.vi"() -> ("output_Reward_OnOff"=w1497:i32)  [unwired: 11 in]
              n783 = call "myRIO_BRig_RT_dataLC_Reward_Probability.vi"() -> ("output_Reward_Probability"=w1493:i32)  [unwired: 11 in]
              n784 = call "myRIO_BRig_RT_dataLC_Reward_Tdelay.vi"() -> ("output_Reward_Tdelay"=w1491:i32)  [unwired: 11 in]
              n785 = call "myRIO_BRig_RT_dataLC_Reward_Trial.vi"() -> ("output_Reward_Trial"=w1489:i32)  [unwired: 11 in]
              n786 = local read "LC_Wrong_OnOff"() -> (w1481:bool)
              n787 = local read "LC_Wrong_Probability"() -> (w1478:u16)
              n788 = local read "LC_Wrong_Block"() -> (w1480:u16)
              n789 = local read "LC_Wrong_Tdelay"() -> (w1477:u16)
              n790 = local read "LC_Wrong_Trial"() -> (w1476:u16)
              n791 = local read "LC_Reward_Probability"() -> (w1492:u16)
              n792 = local read "LC_Reward_Block"() -> (w1498:u16)
              n793 = local read "LC_Reward_Tdelay"() -> (w1490:u16)
              n794 = local read "LC_Reward_OnOff"() -> (w1496:bool)
              n795 = local read "LC_Reward_Trial"() -> (w1488:u16)
              n796 = Boolean To (0,1)(Boolean=w1481) -> (0, 1=w1482:i16)
              n797 = Boolean To (0,1)(Boolean=w1496) -> (0, 1=w1495:i16)
              n798 = To Unsigned Word Integer(number=w1482) -> (unsigned 16bit integer=w1479:u16)
              n799 = To Unsigned Word Integer(number=w1495) -> (unsigned 16bit integer=w1494:u16)
              n800 = Replace Array Subset(array=w1500, new element #1=w1498, index #1=w1499, new element #2=w1494, index #2=w1497, new element #3=w1492, index #3=w1493, new element #4=w1490, index #4=w1491, new element #5=w1488, index #5=w1489, new element #6=w1480, index #6=w1487, new element #7=w1479, index #7=w1486, new element #8=w1478, index #8=w1485, new element #9=w1477, index #9=w1484, new element #10=w1476, index #10=w1483) -> (w1501:u16[])
            }
            frame "setSettings_Audio" {
              # "amp_L"
              # "amp_R"
              # "freq_L"
              # "freq_R"
              n801 = call "myRIO_BRig_RT_dataExp_Audio_amp__L.vi"() -> ("output_Audio_amp__L"=w1526:i32)  [unwired: 11 in]
              n802 = call "myRIO_BRig_RT_dataExp_Audio_amp__R.vi"() -> ("output_Audio_amp__R"=w1525:i32)  [unwired: 11 in]
              n803 = call "myRIO_BRig_RT_dataExp_Audio_freq__L.vi"() -> ("output_Audio_freq__L"=w1524:i32)  [unwired: 11 in]
              n804 = call "myRIO_BRig_RT_dataExp_Audio_freq__R.vi"() -> ("output_Audio_freq__R"=w1523:i32)  [unwired: 11 in]
              n805 = Index Array(array=w1522, index #1=w1526, index #2=w1525, index #3=w1524, index #4=w1523) -> (element #1=w1521:u16, element #2=w1520:u16, element #3=w1513:u16, element #4=w1511:u16)
              n806 = To Unsigned Byte Integer(number=w1513) -> (unsigned 8bit integer=w1512:u8)
              n807 = To Unsigned Byte Integer(number=w1511) -> (unsigned 8bit integer=w1510:u8)
            }
            frame "setSettings_Laser" {
              (unwired) u32 0 ("tDelay_laser_rew")
              # "Wrong tDelay"
              # "Reward tDelay"
              n808 = call "myRIO_BRig_RT_dataLC_Reward_Tdelay.vi"() -> ("output_Reward_Tdelay"=w1553:i32)  [unwired: 11 in]
              n809 = call "myRIO_BRig_RT_dataLC_Wrong_Tdelay.vi"() -> ("output_Wrong_Tdelay"=w1554:i32)  [unwired: 11 in]
              n810 = Index Array(array=w1550, index #1=w1553, index #2=w1554) -> (element #1=w1552:u16, element #2=w1551:u16)
              n811 = call "myRIO_BRig_RT__calc_Tvalley.vi"("input_peakWidth"="laser_Tpeak", "input_freq"="laser_Freq") -> ("output_Tvalley"=w1560:dbl)  [unwired: 9 in]
              n812 = To Double Precision Float(number=w1552) -> (double precision float=w1547:dbl)
              n813 = To Double Precision Float(number=w1551) -> (double precision float=w1544:dbl)
              n814 = Multiply(x="f_millisec2count", y="laser_Tpeak") -> (x*y=w1569:dbl)
              n815 = Multiply(x="f_millisec2count", y=w1560) -> (x*y=w1566:dbl)
              n816 = Multiply(x="f_millisec2count", y="laser_Tshutter") -> (x*y=w1564:dbl)
              n817 = Round Toward +Infinity(x="laser_Tshutter") -> (ceil(x): smallest int >= x=w1555:dbl)
              n818 = Multiply(x="f_millisec2count", y=w1547) -> (x*y=w1548:dbl)
              n819 = Multiply(x="f_millisec2count", y=w1544) -> (x*y=w1545:dbl)
              n820 = To Unsigned Word Integer(number="f_millisec2count") -> (unsigned 16bit integer=w1535:u16)
              n821 = Round Toward +Infinity(x=w1569) -> (ceil(x): smallest int >= x=w1570:dbl)
              n822 = Round Toward +Infinity(x=w1566) -> (ceil(x): smallest int >= x=w1567:dbl)
              n823 = Round Toward +Infinity(x=w1564) -> (ceil(x): smallest int >= x=w1559:dbl)
              n824 = Round Toward +Infinity(x=w1548) -> (ceil(x): smallest int >= x=w1549:dbl)
              n825 = Round Toward +Infinity(x=w1545) -> (ceil(x): smallest int >= x=w1546:dbl)
              n826 = To Unsigned Long Integer(number=w1570) -> (unsigned 32bit integer=w1568:u32)
              n827 = To Unsigned Long Integer(number=w1567) -> (unsigned 32bit integer=w1565:u32)
              n828 = To Unsigned Long Integer(number=w1559) -> (unsigned 32bit integer=w1563:u32)
              n829 = To Unsigned Word Integer(number=w1555) -> (unsigned 16bit integer=w1558:u16)
              n830 = To Unsigned Long Integer(number=w1549) -> (unsigned 32bit integer=w1543:u32)
              n831 = To Unsigned Long Integer(number=w1546) -> (unsigned 32bit integer=w1542:u32)
              n832 = Add(x="laser_duration", y=w1558) -> (x+y=w1539:u16)
              n833 = To Double Precision Float(number=w1539) -> (double precision float=w1538:dbl)
              n834 = Multiply(x=w1538, y="f_millisec2count") -> (x*y=w1540:dbl)
              n835 = call "myRIO_BRig_RT_dataCurrent_LaserPulse_duration.vi"() -> ("output_LaserPulse_duration"=w1571:i32)  [unwired: 11 in]
              n836 = Round Toward +Infinity(x=w1540) -> (ceil(x): smallest int >= x=w1541:dbl)
              n837 = To Unsigned Long Integer(number=w1541) -> (unsigned 32bit integer=w1537:u32)
              n838 = xnode "Read/Write Control"("FPGA VI Reference In"=w1573, "error in"=w1574, "laser_Npeak"=w1568, "laser_Nvalley"=w1565, "laser_Nshutter"=w1563, "laser_selRew_Ndelay"=w1543, "laser_selWro_NDelay"=w1542, "laser_selRew_Ntotal"=w1537, "laser_selWro_Ntotal"=w1537, "k1__counter_per_ms"=w1535) -> ("error out"=→"error out":errorcluster)  [unwired: 1 out]
              n839 = Replace Array Subset(array=w1550, new element=w1539, index=w1571) -> (w1572:u16[])
            }
            frame "initBlock" {
              n840 = call "myRIO_Brig_RT__Case_Exp_State_initBlock.vi"("input_spout"=w1618, "input_dataExp"=w1616, "input_dataCurrent"=w1617) -> ("output_spout"=w1596:enum16{"Left", "Right"}, "output_state"=w1619:T2, "output_dataExp"=w1615:u16[], "output_dataCurrent"=w1601:u16[], "output_TpB_target"=→"TpB_target":u16)  [unwired: 4 in]
              "cSpout" <- w1596
              n841 = call "myRIO_BRig_RT_dataCurrent_iBlock.vi"() -> ("output_iBlock"=w1600:i32)  [unwired: 11 in]
              n842 = Index Array(array=w1601, index=w1600) -> (element=w1594:u16)
              "iBlock" <- w1594
            }
            frame "initBlock2" {
              n843 = local write "nRewards_cur"(u16 0 ("nRewards_cur")) -> ()
              n844 = call "myRIO_BRig_RT__Case_Exp_State_initBlock2.vi"("input_spout"=w1627, "input_dataBlock"=w1628, "input_dataCurrent"=w1626) -> ("idxDataBlock"=w1623:i32, "output_dataBlock"=w1625:u16[][])  [unwired: 7 in]
            }
            frame "initTrial" {
              n845 = call "myRIO_Brig_RT__Case_Exp_State_initTrial.vi"("input_spout"=w1646, "input_dataExp"=w1662, "input_dataCurrent"=w1663) -> ("output_state"=w1664:T2, "output_dataExp"=w1661:u16[], "output_dataCurrent"=w1651:u16[])  [unwired: 6 in]
              n846 = call "myRIO_BRig_RT_dataCurrent_iTrial.vi"() -> ("output_iTrial"=w1650:i32)  [unwired: 11 in]
              n847 = call "myRIO_BRig_RT_dataCurrent_SolenoidReward.vi"() -> ("output_SolenoidReward"=w1645:i32)  [unwired: 11 in]
              n848 = Index Array(array=w1651, index #1=w1650, index #2=w1645) -> (element #1=w1641:u16, element #2=w1644:u16)
              "iTrial" <- w1641
              n849 = Not Equal To 0?(x=w1644) -> (x != 0?=→"SolenoidReward":bool)
            }
            frame "initTrial2" {
              # "trialUntilReward"
              n850 = call "myRIO_BRig_RT__Case_Exp_subState_LC__initTrial.vi"("input_dataTrial"=w1671, "input_spout"=w1680, "input_dataCurrent"=w1669, "input_dataLC"=w1668) -> ("output_LC_Wrong"=w1681:bool, "output_LC_led_Wrong"=w1673:bool, "output_LC_Reward"=w1682:bool, "output_LC_led_Reward"=w1672:bool, "output_dataTrial"=w1670:u16[][])  [unwired: 2 in]
              n851 = Equal?(x=w1680, y=enum16{"Left", "Right"}."Right") -> (x = y?=w1678:bool)
              n852 = call "myRIO_BRig_RT_dataExp_ItrialUntilReward.vi"() -> ("output_I_trialUntilReward"=w1676:i32)  [unwired: 11 in]
              n853 = Index Array(array=w1677, index=w1676) -> (element=w1675:u16)
              n854 = Not Equal To 0?(x=w1675) -> (x != 0?=w1674:bool)
              n855 = xnode "Read/Write Control"("FPGA VI Reference In"=w1695, "error in"=w1694, "SelectionState"=FALSE, "laserResponse_reward"=w1682, "laserResponse_wrong"=w1681, "laserResponse_reward_LED"=w1672, "laserResponse_wrong_LED"=w1673, "Left(F)_or_Right(T)"=w1678, "ignoreWrong"=w1674) -> ("error out"=→"error_initTrial":errorcluster)  [unwired: 1 out]
            }
            frame "initTrial3" {
              n856 = call "myRIO_BRig_RT__Case_Exp_State_initTrial_dataTrial.vi"("input_spout"=w1710, "input_dataCurrent"=w1711, "input_dataExp"=w1709, "input_dataTrial"=w1713) -> ("output_dataTrial"=w1712:u16[][], "output_laserPower"=w1706:u16)  [unwired: 6 in]
              n857 = To Double Precision Float(number=w1706) -> (double precision float=w1708:dbl)
              n858 = Divide(x=w1708, y=100.0 ("x")) -> (x/y=w1702:dbl)
              "output_PortA" <- w1702
              n859 = call "myRIO__convert__Voltage_to_FPGAvalue.vi"("input_voltage"=w1702) -> ("output_PortA"=w1701:u16)  [unwired: 9 in, 1 out]
              n860 = xnode "Read/Write Control"("FPGA VI Reference In"=w1705, "error in"=w1704, "AnaOut_0"=w1701) -> ("error out"=→"error out 4":errorcluster)  [unwired: 1 out]
            }
            frame "initTrial4" {
              n861 = call "myRIO_BRig_RT_dataCurrent_idxDataTrial.vi"() -> ("output_idxDataTrial"=w1736:i32)  [unwired: 11 in]
              n862 = call "myRIO_BRig_RT_dataTrial_activeRecording.vi"() -> ("output_activeRecording"=w1733:i32)  [unwired: 11 in]
              n863 = Index Array(array=w1738, index=w1736) -> (element=w1735:u16)
              n864 = Boolean To (0,1)(Boolean="Recording") -> (0, 1=w1732:i16)
              n865 = To Long Integer(number=w1735) -> (32bit integer=w1734:i32)
              n866 = To Unsigned Word Integer(number=w1732) -> (unsigned 16bit integer=w1731:u16)
              n867 = Replace Array Subset(array=w1737, new element=w1731, index (row)=w1734, index (col)=w1733) -> (w1730:u16[][])
            }
            frame "initTrial_LC_ENL1" {
              w1760 = TRUE ("Recording")
              n868 = call "myRIO_BRig_RT__Case_Exp_State_initTrial_LC_ENL1__v2.vi"("input_dataTrial"=w1763, "input_spout"=w1768, "input_dataBlock"=w1761, "input_dataLC"=w1769, "input_dataCurrent"=w1765) -> ("output_LC__ENL1"=w1767:bool, "output_LC_led__ENL1"=w1766:bool, "output_dataTrial"=w1762:u16[][], "output_dataCurrent"=w1764:u16[])  [unwired: 3 in]
            }
            frame "initTrial_LC_Cue1" {
              n869 = local read "Recording"() -> (w1785:bool)
              n870 = call "myRIO_BRig_RT__Case_Exp_State_initTrial_LC_Cue1__v2.vi"("input_dataTrial"=w1792, "input_spout"=w1795, "input_dataBlock"=w1790, "input_dataLC"=w1796, "input_dataCurrent"=w1794) -> ("output_LC__Cue1"=w1788:bool, "output_LC_led__Cue1"=w1789:bool, "output_dataTrial"=w1791:u16[][], "output_dataCurrent"=w1793:u16[])  [unwired: 3 in]
            }
            frame "ENL1_pre" {
              # "ENL1_n"
              # "Tcycle"
              # "counter"
              n871 = call "myRIO_BRig_RT_dataCurrent_Tcycle_generic.vi"() -> ("output_Tcycle_generic"=w1842:i32)  [unwired: 11 in]
              n872 = call "myRIO_BRig_RT_dataCurrent_count_generic.vi"() -> ("output_count_generic"=w1844:i32)  [unwired: 11 in]
              n873 = call "myRIO_BRig_RT_dataCurrent_ENL.vi"() -> ("output_ENL"=w1841:i32)  [unwired: 11 in]
              n874 = call "myRIO_BRig_RT_dataCurrent_ENL1_n.vi"() -> ("output_ENL1_n"=w1813:i32)  [unwired: 11 in]
              n875 = Index Array(array=w1835, index #1=w1841, index #2=w1813) -> (element #1=w1840:u16, element #2=w1812:u16)
              n876 = Increment(x=w1812) -> (x+1=w1811:u16)
              n877 = Replace Array Subset(array=w1835, new element #1=u16 0 ("new element/subarray"), index #1=w1844, new element #2=w1840, index #2=w1842, new element #3=w1811, index #3=w1813) -> (w1839:u16[])
              n878 = Select(t=myRIO_BRig_RT__Case_Exp_stateList."ENL1Penalty_pre" ("Enum"), s=w1823, f=myRIO_BRig_RT__Case_Exp_stateList."ENL1" ("Enum")) -> (s? t:f=w1820:T2)
            }
            frame "ENL1" {
              n879 = call "myRIO_BRig_RT__Case_Exp_State_ENL1__v2.vi"("input_LC"=w1851, "I_lick"=w1855, "input_LC_led"=w1852, 9:w1847, "input_state"=w1861, "input_dataCurrent"=w1860) -> ("output_trigger_laser_led"=w1850:bool, "output_state"=w1858:T2, "output_dataCurrent"=w1859:u16[], "output_trigger_laser"=w1849:bool)  [unwired: 2 in]
              n880 = Or(x=w1850, y=w1847) -> (x .or. y?=w1853:bool)
            }
            frame "ENL1Penalty_pre" {
              # "Tcycle"
              # "counter"
              n881 = call "myRIO_BRig_RT_dataCurrent_Tcycle_generic.vi"() -> ("output_Tcycle_generic"=w1901:i32)  [unwired: 11 in]
              n882 = call "myRIO_BRig_RT_dataCurrent_count_generic.vi"() -> ("output_count_generic"=w1903:i32)  [unwired: 11 in]
              n883 = call "myRIO_BRig_RT_dataExp_ENL_penalty.vi"() -> ("output_ENL_penalty"=w1896:i32)  [unwired: 11 in]
              n884 = Index Array(array=w1897, index=w1896) -> (element=w1900:u16)
              n885 = Replace Array Subset(array=w1898, new element #1=u16 0 ("new element/subarray"), index #1=w1903, new element #2=w1900, index #2=w1901) -> (w1899:u16[])
            }
            frame "ENL1Penalty" {
              n886 = call "myRIO_BRig_RT__Case_Exp_State_ENL1Penalty.vi"("input_state"=w1926, "input_dataCurrent"=w1930) -> ("output_state"=w1927:T2, "output_dataCurrent"=w1929:u16[])  [unwired: 8 in]
            }
            frame "ENL2_pre" {
            }
            frame "ENL2" {
            }
            frame "ENL2Penalty_pre" {
            }
            frame "ENL2Penalty" {
            }
            frame "Cue1_pre" {
              # "Cue1_n"
              # "Tcycle_Cue1"
              # "0 = L, 1 = R, 2 = both"
              # "sp_R"
              # "sp_L"
              # "Tcycle"
              # "counter"
              n887 = Equal?(x=w2041, y=enum16{"Left", "Right"}."Left") -> (x = y?=w2040:bool)
              n888 = call "myRIO_BRig_RT_dataExp_Audio_sp__L.vi"() -> ("output_Audio_sp__L"=w2039:i32)  [unwired: 11 in]
              n889 = call "myRIO_BRig_RT_dataExp_Audio_sp__R.vi"() -> ("output_Audio_sp__R"=w2038:i32)  [unwired: 11 in]
              n890 = call "myRIO_BRig_RT_dataCurrent_Tcycle_generic.vi"() -> ("output_Tcycle_generic"=w2051:i32)  [unwired: 11 in]
              n891 = call "myRIO_BRig_RT_dataCurrent_count_generic.vi"() -> ("output_count_generic"=w2053:i32)  [unwired: 11 in]
              n892 = Select(t=w2039, s=w2040, f=w2038) -> (s? t:f=w2037:i32)
              n893 = call "myRIO_BRig_RT_dataCurrent_Cue1_n.vi"() -> ("output_Cue1_n"=w2015:i32)  [unwired: 11 in]
              n894 = call "myRIO_BRig_RT_dataCurrent_Tcycle_cue.vi"() -> ("output_Tcycle_cue"=w2024:i32)  [unwired: 11 in]
              n895 = Index Array(array=w2043, index=w2037) -> (element=w2035:u16)
              n896 = Index Array(array=w2025, index #1=w2024, index #2=w2015) -> (element #1=w2026:u16, element #2=w2017:u16)
              n897 = Increment(x=w2017) -> (x+1=w2016:u16)
              n898 = Not Equal To 0?(x=w2035) -> (x != 0?=w2033:bool)
              n899 = Not Equal?(x=w2035, y=u16 1) -> (x != y?=w2034:bool)
              n900 = Replace Array Subset(array=w2025, new element #1=u16 0 ("new element/subarray"), index #1=w2053, new element #2=w2026, index #2=w2051, new element #3=w2016, index #3=w2015) -> (w2050:u16[])
              n901 = Select(t=myRIO_BRig_RT__Case_Exp_stateList."Cue1Penalty_pre" ("Enum"), s=w2021, f=myRIO_BRig_RT__Case_Exp_stateList."Cue1" ("Enum")) -> (s? t:f=w2022:T2)
            }
            frame "Cue1" {
              n902 = call "myRIO_BRig_RT__Case_Exp_State_Cue1__v2.vi"("input_LC"=w2063, "I_lick"=w2066, "input_LC_led"=w2064, 9:w2058, "input_state"=w2068, "input_dataCurrent"=w2086) -> ("output_trigger_laser_led"=w2061:bool, "output_state"=w2067:T2, "output_dataCurrent"=w2085:u16[], "output_trigger_laser"=w2062:bool)  [unwired: 2 in]
              n903 = Or(x=w2061, y=w2058) -> (x .or. y?=w2060:bool)
              n904 = Equal?(x=myRIO_BRig_RT__Case_Exp_stateList."Selection_pre", y=w2067) -> (x = y?=w2071:bool)
              n905 = xnode "Read/Write Control"("FPGA VI Reference In"=w2070, "error in"=w2069, "SelectionState"=w2071) -> ()  [unwired: 2 out]
            }
            frame "Cue1Penalty_pre" {
              # "Tcycle"
              # "counter"
              n906 = call "myRIO_BRig_RT_dataCurrent_Tcycle_generic.vi"() -> ("output_Tcycle_generic"=w2117:i32)  [unwired: 11 in]
              n907 = call "myRIO_BRig_RT_dataCurrent_count_generic.vi"() -> ("output_count_generic"=w2119:i32)  [unwired: 11 in]
              n908 = call "myRIO_BRig_RT_dataExp_Tcycle_CuePenalty.vi"() -> ("output_Tcycle_CuePenalty"=w2116:i32)  [unwired: 11 in]
              n909 = Index Array(array=w2111, index=w2116) -> (element=w2115:u16)
              n910 = Replace Array Subset(array=w2113, new element #1=u16 0 ("new element/subarray"), index #1=w2119, new element #2=w2115, index #2=w2117) -> (w2112:u16[])
            }
            frame "Cue1Penalty" {
              # "reset laserOccurred"
              n911 = call "myRIO_BRig_RT__Case_Exp_State_Cue1Penalty.vi"("input_state"=w2143, "input_dataCurrent"=w2144) -> ("output_state"=w2141:T2, "output_dataCurrent"=w2142:u16[])  [unwired: 8 in]
            }
            frame "Cue2_pre" {
              n912 = call "myRIO_BRig_RT__Case_Exp_subState_LC__Cue2.vi"("input_spout"=w2161, "input_dataCurrent"=w2162, "input_dataLC"=w2160) -> ()  [unwired: 6 in, 2 out]
            }
            frame "Cue2" {
            }
            frame "Cue2Penalty_pre" {
            }
            frame "Cue2Penalty" {
            }
            frame "Selection_pre" {
              # "Tcycle"
              # "counter"
              n913 = xnode "Read/Write Control"("FPGA VI Reference In"=w2233, "error in"=w2234) -> ("error out"=→"error_Selection_pre":errorcluster, "SelectReward"=w2226:bool, "SelectWrong"=w2228:bool)  [unwired: 1 out]
              n914 = call "myRIO_BRig_RT_dataCurrent_Tcycle_generic.vi"() -> ("output_Tcycle_generic"=w2255:i32)  [unwired: 11 in]
              n915 = call "myRIO_BRig_RT_dataCurrent_count_generic.vi"() -> ("output_count_generic"=w2257:i32)  [unwired: 11 in]
              n916 = call "myRIO_BRig_RT_dataExp_Tcycle_Selection.vi"() -> ("output_Tcycle_Selection"=w2254:i32)  [unwired: 11 in]
              n917 = Index Array(array=w2251, index=w2254) -> (element=w2253:u16)
              n918 = Replace Array Subset(array=w2249, new element #1=u16 0 ("new element/subarray"), index #1=w2257, new element #2=w2253, index #2=w2255) -> (w2252:u16[])
              n919 = Or(x=w2226, y=w2228) -> (x .or. y?=w2227:bool)
              n920 = Select(t=myRIO_BRig_RT__Case_Exp_stateList."SelectReward_pre" ("Enum"), s=w2226, f=myRIO_BRig_RT__Case_Exp_stateList."SelectWrong_pre" ("Enum")) -> (s? t:f=w2232:T2)
              n921 = Select(t=w2232, s=w2227, f=myRIO_BRig_RT__Case_Exp_stateList."Selection" ("Enum")) -> (s? t:f=w2229:T2)
            }
            frame "Selection" {
              # "counter\nSelection"
              # "increment"
              # "get Tcycle"
              # "get count"
              n922 = xnode "Read/Write Control"("FPGA VI Reference In"=w2282, "error in"=w2281) -> ("error out"=→"error_Selection":errorcluster, "SelectReward"=w2278:bool, "SelectWrong"=w2279:bool)  [unwired: 1 out]
              n923 = call "myRIO_BRig_RT_dataCurrent_Tcycle_generic.vi"() -> ("output_Tcycle_generic"=w2275:i32)  [unwired: 11 in]
              n924 = call "myRIO_BRig_RT_dataCurrent_count_generic.vi"() -> ("output_count_generic"=w2268:i32)  [unwired: 11 in]
              n925 = Index Array(array=w2276, index #1=w2275, index #2=w2268) -> (element #1=w2267:u16, element #2=w2274:u16)
              n926 = call "myRIO_BRig_RT__increment_u16.vi"() -> ("output_increment__u16"=w2273:u16)  [unwired: 11 in]
              n927 = Add(x=w2274, y=w2273) -> (x+y=w2269:u16)
              n928 = Greater?(x=w2267, y=w2269) -> (0:w2261:bool)
              n929 = Select(t=w2272, s=w2261, f=myRIO_BRig_RT__Case_Exp_stateList."SelectTimeout_pre" ("Enum")) -> (s? t:f=w2262:T2)
              n930 = Select(t=w2269, s=w2261, f=w2267) -> (s? t:f=w2265:u16)
              n931 = call "myRIO_BRig_RT_dataCurrent_count_selection.vi"() -> ("output_count_generic"=w2266:i32)  [unwired: 11 in]
              n932 = Select(t=myRIO_BRig_RT__Case_Exp_stateList."SelectReward_pre" ("Enum"), s=w2278, f=myRIO_BRig_RT__Case_Exp_stateList."SelectWrong_pre" ("Enum")) -> (s? t:f=w2277:T2)
              n933 = Replace Array Subset(array=w2276, new element #1=w2265, index #1=w2268, new element #2=w2265, index #2=w2266) -> (w2271:u16[])
              n934 = Or(x=w2278, y=w2279) -> (x .or. y?=w2260:bool)
              n935 = Select(t=w2277, s=w2260, f=w2262) -> (s? t:f=w2280:T2)
            }
            frame "SelectReward_pre" {
              # "iState"
              # "Tcycle\nReward"
              # "nRewTrials"
              # "Tcycle\nGeneric"
              # "counter"
              n936 = call "myRIO_BRig_RT_dataCurrent_nRewTrials.vi"() -> ("output_nRewTrials"=w2314:i32)  [unwired: 11 in]
              n937 = Equal?(x=w2323, y=enum16{"Left", "Right"}."Left") -> (x = y?=w2324:bool)
              n938 = Index Array(array=w2315, index=w2314) -> (element=w2313:u16)
              n939 = call "myRIO_BRig_RT_dataExp_Tcycle_Reward__L.vi"() -> ("output_Tcycle_Reward__L"=w2327:i32)  [unwired: 11 in]
              n940 = call "myRIO_BRig_RT_dataExp_Tcycle_Reward__R.vi"() -> ("output_Tcycle_Reward__R"=w2328:i32)  [unwired: 11 in]
              n941 = Increment(x=w2313) -> (x+1=w2312:u16)
              n942 = Select(t=w2327, s=w2324, f=w2328) -> (s? t:f=w2326:i32)
              n943 = call "myRIO_BRig_RT__Case_Exp_subState_LC__Reward.vi"("input_spout"=w2323, "input_dataCurrent"=w2315, "input_dataLC"=w2322) -> ()  [unwired: 6 in, 2 out]
              n944 = call "myRIO_BRig_RT_dataCurrent_count_generic.vi"() -> ("output_count_generic"=w2317:i32)  [unwired: 11 in]
              n945 = call "myRIO_BRig_RT_dataCurrent_Tcycle_generic.vi"() -> ("output_Tcycle_generic"=w2318:i32)  [unwired: 11 in]
              n946 = Index Array(array=w2329, index=w2326) -> (element=w2319:u16)
              n947 = call "myRIO_BRig_RT_dataCurrent_iState.vi"() -> ("output_iState"=w2307:i32)  [unwired: 11 in]
              n948 = Replace Array Subset(array=w2315, new element #1=w2312, index #1=w2314, new element #2=u16 0 ("new element/subarray"), index #2=w2317, new element #3=w2319, index #3=w2318, new element #4=u16 1 ("new element/subarray"), index #4=w2307) -> (w2330:u16[])
            }
            frame "SelectReward" {
              n949 = call "myRIO_BRig_RT__Case_Exp_State_Reward.vi"("input_dataCurrent"=w2351, "input_state"=w2348, "input_spout"=w2346) -> ("output_dataCurrent"=w2350:u16[], "output_state"=w2349:T2, "output__L"=w2344:bool, "output__R"=w2345:bool)  [unwired: 9 in]
            }
            frame "SelectRewardPost_pre" {
              # "nRewards"
              # "nRewTrials"
              # "Tcycle"
              # "counter"
              n950 = call "myRIO_BRig_RT_dataBlock_nRewards__L.vi"() -> ("output_nRewards__L"=w2367:i32)  [unwired: 11 in]
              n951 = call "myRIO_BRig_RT_dataBlock_nRewards__R.vi"() -> ("output_nRewards__R"=w2366:i32)  [unwired: 11 in]
              n952 = call "myRIO_BRig_RT_dataCurrent_Tcycle_generic.vi"() -> ("output_Tcycle_generic"=w2386:i32)  [unwired: 11 in]
              n953 = call "myRIO_BRig_RT_dataCurrent_count_generic.vi"() -> ("output_count_generic"=w2388:i32)  [unwired: 11 in]
              n954 = case shown="\"Left\", Default" w2360 {
                tunnel: w2372 -> [w2393 w2397]
                tunnel: [w2392 w2397] -> w2371
                tunnel: [w2394 w2395] -> w2370
                tunnel: w2369 -> [w2394 w2396]
                frame "Left", Default {
                  n955 = Increment(x=w2393) -> (x+1=w2392:u16)
                }
                frame "Right" {
                  n956 = Increment(x=w2396) -> (x+1=w2395:u16)
                }
              }
              "nRewards_Left" <- w2371
              "nRewards_Right" <- w2370
              n957 = Equal?(x=w2360, y=enum16{"Left", "Right"}."Left") -> (x = y?=w2359:bool)
              n958 = Select(t=w2367, s=w2359, f=w2366) -> (s? t:f=w2365:i32)
              n959 = call "myRIO_BRig_RT_dataExp_Tcycle_RewardPost.vi"() -> ("output_Tcycle_RewardPost"=w2382:i32)  [unwired: 11 in]
              n960 = call "myRIO_BRig_RT_dataCurrent_nRewTrials.vi"() -> ("output_nRewTrials"=w2368:i32)  [unwired: 11 in]
              n961 = Index Array(array=w2383, index=w2382) -> (element=w2385:u16)
              n962 = Index Array(array=w2362, index=w2368) -> (element=w2357:u16)
              n963 = Replace Array Subset(array=w2362, new element #1=u16 0 ("new element/subarray"), index #1=w2388, new element #2=w2385, index #2=w2386) -> (w2384:u16[])
              n964 = Replace Array Subset(array=w2364, new element=w2357, index (row)=w2358, index (col)=w2365) -> (w2363:u16[][])
              n965 = local write "nRewards_cur"(w2357) -> ()
            }
            frame "SelectRewardPost" {
              n966 = call "myRIO_BRig_RT__Case_Exp_State_RewardPost.vi"("input_state"=w2412, "input_dataCurrent"=w2415) -> ("output_state"=w2413:T2, "output_dataCurrent"=w2414:u16[])  [unwired: 8 in]
            }
            frame "SelectWrong_pre" {
              # "iState"
              # "Tcycle"
              # "counter"
              n967 = call "myRIO_BRig_RT_dataCurrent_Tcycle_generic.vi"() -> ("output_Tcycle_generic"=w2440:i32)  [unwired: 11 in]
              n968 = call "myRIO_BRig_RT_dataCurrent_count_generic.vi"() -> ("output_count_generic"=w2442:i32)  [unwired: 11 in]
              n969 = call "myRIO_BRig_RT_dataExp_Tcycle_Wrong.vi"() -> ("output_Tcycle_Wrong"=w2438:i32)  [unwired: 11 in]
              n970 = call "myRIO_BRig_RT__Case_Exp_subState_LC__Wrong.vi"("input_spout"=w2434, "input_dataCurrent"=w2435, "input_dataLC"=w2432) -> ()  [unwired: 6 in, 2 out]
              n971 = Index Array(array=w2436, index=w2438) -> (element=w2439:u16)
              n972 = call "myRIO_BRig_RT_dataCurrent_iState.vi"() -> ("output_iState"=w2426:i32)  [unwired: 11 in]
              n973 = Replace Array Subset(array=w2435, new element #1=u16 0 ("new element/subarray"), index #1=w2442, new element #2=w2439, index #2=w2440, new element #3=u16 2 ("new element/subarray"), index #3=w2426) -> (w2437:u16[])
            }
            frame "SelectWrong" {
              n974 = call "myRIO_BRig_RT__Case_Exp_State_Wrong.vi"("input_state"=w2456, "input_dataCurrent"=w2465) -> ("output_state"=w2453:T2, "output_dataCurrent"=w2464:u16[])  [unwired: 8 in]
              n975 = Not Equal?(x=w2456, y=w2453) -> (x != y?=w2455:bool)
              n976 = Select(t=myRIO_BRig_RT__Case_Exp_stateList."SelectWrong_post" ("Enum"), s=w2455, f=w2453) -> (s? t:f=w2452:T2)
            }
            frame "SelectWrong_post" {
            }
            frame "SelectTimeout_pre" {
              # "iState"
              # "Tcycle"
              # "counter"
              n977 = xnode "Read/Write Control"("FPGA VI Reference In"=w2492, "error in"=w2491, "SelectionState"=FALSE) -> ("error out"=→"error out 3":errorcluster)  [unwired: 1 out]
              n978 = call "myRIO_BRig_RT_dataCurrent_Tcycle_generic.vi"() -> ("output_Tcycle_generic"=w2514:i32)  [unwired: 11 in]
              n979 = call "myRIO_BRig_RT_dataCurrent_count_generic.vi"() -> ("output_count_generic"=w2512:i32)  [unwired: 11 in]
              n980 = call "myRIO_BRig_RT_dataExp_Tcycle_Timeout.vi"() -> ("output_Tcycle_Timeout"=w2516:i32)  [unwired: 11 in]
              n981 = call "myRIO_BRig_RT__Case_Exp_subState_LC__Timeout.vi"("input_spout"=w2507, "input_dataCurrent"=w2508, "input_dataLC"=w2506) -> ()  [unwired: 6 in, 2 out]
              n982 = Index Array(array=w2510, index=w2516) -> (element=w2515:u16)
              n983 = call "myRIO_BRig_RT_dataCurrent_iState.vi"() -> ("output_iState"=w2500:i32)  [unwired: 11 in]
              n984 = Replace Array Subset(array=w2508, new element #1=u16 0 ("new element/subarray"), index #1=w2512, new element #2=w2515, index #2=w2514, new element #3=u16 3 ("new element/subarray"), index #3=w2500) -> (w2511:u16[])
            }
            frame "SelectTimeout" {
              n985 = call "myRIO_BRig_RT__Case_Exp_State_Timeout.vi"("input_dataLC"=w2535, "input_LC"=w2536, "input_state"=w2526, "input_dataCurrent"=w2541) -> ("output_state"=w2527:T2, "output_dataCurrent"=w2540:u16[])  [unwired: 5 in, 1 out]
              n986 = Not Equal?(x=w2526, y=w2527) -> (x != y?=w2530:bool)
              n987 = Select(t=myRIO_BRig_RT__Case_Exp_stateList."SelectTimeout_post" ("Enum"), s=w2530, f=w2527) -> (s? t:f=w2528:T2)
            }
            frame "SelectTimeout_post" {
            }
            frame "endTrial1" {
              # "Update dataBlock"
              n988 = call "myRIO_BRig_RT__Case_Exp_State_endTrial1.vi"("input_spout"=w2574, "input_dataBlock"=w2573, "input_dataCurrent"=w2571) -> ("output_dataBlock"=w2572:u16[][], "output_dataCurrent"=w2570:u16[])  [unwired: 7 in]
            }
            frame "endTrial2" {
              # "update dataTrial"
              n989 = call "myRIO_BRig_RT__Case_Exp_State_endTrial2.vi"("input_spout"=w2593, "input_dataTrial"=w2597, "input_dataCurrent"=w2595) -> ("output_dataTrial"=w2596:u16[][], "output_dataCurrent"=w2594:u16[])  [unwired: 7 in]
            }
            frame "endTrial3" {
              w2623 = myRIO_BRig_RT__Case_Exp_stateList."endBlock" ("Enum")
              # "nRewTrials"
              # "iTrial"
              # "I_blockUntilReward"
              # "TPB"
              # "end block?"
              n990 = local read "STOP_endTrial"() -> (w2621:bool)
              n991 = local read "STOP_abort"() -> (w2620:bool)
              n992 = xnode "Read/Write Control"("FPGA VI Reference In"=w2609, "error in"=w2608, "SelectionState"=FALSE) -> ("error out"=→"error out 2":errorcluster)  [unwired: 1 out]
              n993 = local read "START"() -> (w2618:bool)
              n994 = call "myRIO_BRig_RT_dataExp_IblockUntilReward.vi"() -> ("output_I_blockUntilReward"=w2630:i32)  [unwired: 11 in]
              n995 = Index Array(array=w2614, index=w2630) -> (element=w2610:u16)
              n996 = Not(x=w2618) -> (.not. x?=w2619:bool)
              n997 = Not Equal To 0?(x=w2610) -> (x != 0?=w2628:bool)
              n998 = Compound Arithmetic op=OR(w2621, w2619, w2620) -> (w2622:bool)
              n999 = call "myRIO_BRig_RT_dataCurrent_nRewTrials.vi"() -> ("output_nRewTrials"=w2626:i32)  [unwired: 11 in]
              n1000 = call "myRIO_BRig_RT_dataCurrent_iTrial.vi"() -> ("output_iTrial"=w2627:i32)  [unwired: 11 in]
              n1001 = Select(t=w2626, s=w2628, f=w2627) -> (s? t:f=w2625:i32)
              n1002 = call "myRIO_BRig_RT_dataCurrent_TpB.vi"() -> ("output_TpB"=w2629:i32)  [unwired: 11 in]
              n1003 = Index Array(array=w2615, index #1=w2629, index #2=w2625) -> (element #1=w2616:u16, element #2=w2617:u16)
              n1004 = Less Or Equal?(x=w2616, y=w2617) -> (x <= y?=w2613:bool)
              n1005 = Select(t=w2623, s=w2613, f=myRIO_BRig_RT__Case_Exp_stateList."empty_endTrial1" ("Enum")) -> (s? t:f=w2624:T2)
              n1006 = Select(t=w2623, s=w2622, f=w2624) -> (s? t:f=w2611:T2)
            }
            frame "endBlock" {
              # "R"
              # "L"
              # "idxDataBlock"
              n1007 = Equal?(x=w2654, y=enum16{"Left", "Right"}."Left") -> (x = y?=w2653:bool)
              n1008 = call "myRIO_BRig_RT_dataCurrent_idxDataBlockL.vi"() -> ("output_idxDataBlock__L"=w2657:i32)  [unwired: 11 in]
              n1009 = call "myRIO_BRig_RT_dataCurrent_idxDataBlockR.vi"() -> ("output_idxDataBlock__R"=w2656:i32)  [unwired: 11 in]
              n1010 = Increment(x=w2648) -> (x+1=w2647:i32)
              n1011 = Select(t=w2657, s=w2653, f=w2656) -> (s? t:f=w2651:i32)
              n1012 = To Unsigned Word Integer(number=w2647) -> (unsigned 16bit integer=w2649:u16)
              n1013 = local read "START"() -> (w2677:bool)
              n1014 = local read "STOP_endBlock"() -> (w2672:bool)
              n1015 = local read "STOP_endTrial"() -> (w2675:bool)
              n1016 = local read "STOP_abort"() -> (w2674:bool)
              n1017 = Replace Array Subset(array=w2652, new element=w2649, index=w2651) -> (w2650:u16[])
              n1018 = Not(x=w2677) -> (.not. x?=w2676:bool)
              n1019 = Compound Arithmetic op=OR(w2676, w2672, w2675, w2674) -> (w2673:bool)
              n1020 = Select(t=myRIO_BRig_RT__Case_Exp_stateList."endExp" ("Enum"), s=w2673, f=myRIO_BRig_RT__Case_Exp_stateList."empty_endBlock1" ("Enum")) -> (s? t:f=w2681:T2)
            }
            frame "endExp" {
            }
            frame "commConnect" {
              n1021 = call "myRIO_BRig_RT_comm_webdav_connect.vi"("input_password"="Host Password", "input_username"="Host UserName") -> ("output_Iconnected"=w2702:bool, "output_hSession"=w2720:T6)  [unwired: 7 in, 1 out]
              "Connected To Host?" <- w2702
              n1022 = case shown="False" w2702 {
                frame False {
                  n1023 = One Button Dialog(message="Connection Failed!\nData not being saved!") -> ()  [unwired: 1 in, 1 out]
                }
                frame True {
                }
              }
            }
            frame "commUpload_pre" {
              n1024 = Select(t=myRIO_BRig_RT__Case_Exp_stateList."commUpload_dataBlock" ("Enum"), s=w2727, f=myRIO_BRig_RT__Case_Exp_stateList."endTrial3") -> (s? t:f=w2725:T2)
            }
            frame "commUpload_dataBlock" {
              n1025 = call "myRIO_BRig_RT_comm_webdav_uploadFile__data.vi"("input_fileName_prefix"=w2748, "input_fileName"="dataBlock" ("input_filename"), "input_hSession"=w2750) -> ()  [unwired: 8 in, 1 out]
            }
            frame "commUpload_dataCurrent" {
              n1026 = call "myRIO_BRig_RT_comm_webdav_uploadFile__data.vi"("input_fileName_prefix"=w2769, "input_fileName"="dataCurrent" ("input_filename"), "input_hSession"=w2771) -> ()  [unwired: 8 in, 1 out]
            }
            frame "commUpload_dataExp" {
              n1027 = call "myRIO_BRig_RT_comm_webdav_uploadFile__data.vi"("input_fileName_prefix"=w2790, "input_fileName"="dataExp" ("input_filename"), "input_hSession"=w2792) -> ()  [unwired: 8 in, 1 out]
            }
            frame "commUpload_dataLC" {
              n1028 = call "myRIO_BRig_RT_comm_webdav_uploadFile__data.vi"("input_fileName_prefix"=w2811, "input_fileName"="dataLC" ("input_filename"), "input_hSession"=w2813) -> ()  [unwired: 8 in, 1 out]
            }
            frame "commUpload_dataTrial" {
              n1029 = call "myRIO_BRig_RT_comm_webdav_uploadFile__data.vi"("input_fileName_prefix"=w2835, "input_fileName"="dataTrial" ("input_filename"), "input_hSession"=w2837) -> ()  [unwired: 8 in, 1 out]
            }
            frame "saveData_dataBlock" {
              # "idxDataBlockR"
              # "idxDataBlockL"
              n1030 = call "myRIO_BRig_RT_dataCurrent_idxDataBlockL.vi"() -> ("output_idxDataBlock__L"=w2861:i32)  [unwired: 11 in]
              n1031 = call "myRIO_BRig_RT_dataCurrent_idxDataBlockR.vi"() -> ("output_idxDataBlock__R"=w2862:i32)  [unwired: 11 in]
              n1032 = Index Array(array=w2863, index #1=w2861, index #2=w2862) -> (element #1=w2860:u16, element #2=w2859:u16)
              n1033 = Greater?(x=w2860, y=w2859) -> (0:w2858:bool)
              n1034 = Select(t=w2860, s=w2858, f=w2859) -> (s? t:f=w2856:u16)
              n1035 = Increment(x=w2856) -> (x+1=w2855:u16)
              n1036 = To Long Integer(number=w2855) -> (32bit integer=w2854:i32)
              n1037 = Array Subset(array=w2857, length (row)=w2854) -> (w2853:u16[][])  [unwired: 3 in]
              n1038 = call "myRIO_BRig_RT_comm_webdav_saveArrayToFile__2D_u16.vi"("Array"=w2853, "input_filename"="dataBlock") -> ()  [unwired: 10 in]
            }
            frame "saveData_dataCurrent" {
              n1039 = call "myRIO_BRig_RT_comm_webdav_saveArrayToFile__1D_u16.vi"("Array"=w2882, "input_filename"="dataCurrent") -> ()  [unwired: 10 in]
            }
            frame "saveData_dataExp" {
              # "runTime"
              n1040 = Get Date/Time In Seconds() -> (seconds since 1Jan1904=w2910:timestamp)
              n1041 = To Double Precision Float(number=w2910) -> (double precision float=w2909:dbl)
              n1042 = call "myRIO_BRig_RT_dataExp_runTime_seconds.vi"() -> ("output_RunTime_minutes"=w2908:i32)  [unwired: 11 in]
              n1043 = Subtract(x=w2909, y=w2907) -> (x-y=w2904:dbl)
              n1044 = To Unsigned Word Integer(number=w2904) -> (unsigned 16bit integer=w2903:u16)
              n1045 = Replace Array Subset(array=w2902, new element=w2903, index=w2908) -> (w2905:u16[])
              n1046 = call "myRIO_BRig_RT_comm_webdav_saveArrayToFile__1D_u16.vi"("Array"=w2905, "input_filename"="dataExp") -> ()  [unwired: 10 in]
            }
            frame "saveData_dataLC" {
              n1047 = call "myRIO_BRig_RT_comm_webdav_saveArrayToFile__1D_u16.vi"("Array"=w2929, "input_filename"="dataLC") -> ()  [unwired: 10 in]
            }
            frame "saveData_dataTrial" {
              # "idxTrial"
              n1048 = call "myRIO_BRig_RT_dataCurrent_idxDataTrial.vi"() -> ("output_idxDataTrial"=w2954:i32)  [unwired: 11 in]
              n1049 = Index Array(array=w2955, index=w2954) -> (element=w2951:u16)
              n1050 = Increment(x=w2951) -> (x+1=w2950:u16)
              n1051 = To Long Integer(number=w2950) -> (32bit integer=w2949:i32)
              n1052 = Array Subset(array=w2952, length (row)=w2949) -> (w2953:u16[][])  [unwired: 3 in]
              n1053 = call "myRIO_BRig_RT_comm_webdav_saveArrayToFile__2D_u16.vi"("Array"=w2953, "input_filename"="dataTrial") -> ()  [unwired: 10 in]
            }
            frame "empty_endBlock1" {
            }
            frame "empty_endBlock2" {
            }
            frame "empty_endTrial1" {
            }
            frame "empty_endTrial2" {
            }
            frame "empty_endTrial3" {
            }
            frame "empty_endTrial4" {
            }
            frame "empty_endTrial5" {
            }
          }
          n1054 = Select(t=w1022, s=w1025, f=w1023) -> (s? t:f=w1024:bool)
          n1055 = case shown="True" w1099 {
            tunnel: w1096 -> [w1122 w1130]
            tunnel: w1098 -> [_ w1126]
            tunnel: w1097 -> [_ w1125]
            tunnel: w1013 -> [_ w1124]
            tunnel: w1066 -> [_ w1123]
            tunnel: [w1122 w1129] -> w1095
            tunnel: w1094 -> [w1121 w1128]
            tunnel: [w1121 w1127] -> w1093
            frame False {
            }
            frame True {
              n1056 = call "myRIO_BRig_RT__Case_Exp__recordLick.vi"("intput_state__trialEnd"=w1123, "intput_state__trialStart"=w1124, "input_lick__R"=w1125, "input_lick__L"=w1126, "input_dataCurrent"=w1128, "input_dataLick"=w1130) -> ("output_dataCurrent"=w1127:u16[], "output_dataLick"=w1129:u16[][])  [unwired: 4 in]
            }
          }
          n1057 = Or(x=w1068, y=w1069) -> (x .or. y?=w1055:bool)
          n1058 = Or(x=w1072, y=w1052) -> (x .or. y?=w1041:bool)
          n1059 = Or(x=w1051, y=w1073) -> (x .or. y?=w1067:bool)
          n1060 = Or(x=w1071, y=w1070) -> (x .or. y?=w1056:bool)
          n1061 = Or(x=w1100, y="STOP_abort") -> (x .or. y?=w1102:bool)
          n1062 = Or(x=w1030, y=w1031) -> (x .or. y?=w1028:bool)
          n1063 = Or(x=w1032, y=w1031) -> (x .or. y?=w1029:bool)
          n1064 = Select(t=w1008, s=w1009, f=w1007) -> (s? t:f=w1005:u16)
          n1065 = Select(t=w1010, s=w1012, f=w1011) -> (s? t:f=w1006:u16)
          n1066 = Select(t=u16 0, s=w1016, f=w1015) -> (s? t:f=w1003:u16)
          n1067 = xnode "Read/Write Control"("FPGA VI Reference In"=w1043, "error in"=w1042, "A1_SR"=w1056, "A3_SL"=w1055, "A6_Act"=w1024, "audioTrigger_L"=w1041, "audioAmp_L"=w1082, "audioFreq_L_kHz"=w1050, "audioTrigger_R"=w1067, "audioAmp_R"=w1083, "audioFreq_R_kHz"=w1084, "laserledMTrig"=w1028, "laserMTrig"=w1029) -> ("FPGA VI Reference Out"=w1092:refnum<k20>, "error out"=w1091:errorcluster, "AnaIn_0"=w1004:u16, "AnaIn_1"=w1019:u16)
          n1068 = local write "tempAI0"(w1004) -> ()
          n1069 = call "myRIO_BRig_RT_dataAnalog_enterData__PortA.vi"("input_iState"=w1013, "input_AI0"=w1004, "input_iEvent"=w1003, "input_AI1"=w1019, "input_iTrial"=w1005, "input_iBlock"=w1006, "input_index"=w1017, "input_dataAnalog"=w1021) -> ("output_dataAnalog"=w1020:u16[][])  [unwired: 3 in]
          n1070 = node-c288() -> ()  [unwired: 1 in, 1 out]
          n1071 = Increment(x=w1003) -> (x+1=w1002:u16)
          n1072 = Increment(x=w1017) -> (x+1=w1018:i32)
          "cState" <- w1013
        }
        n1073 = node-c288(w959) -> ()  [unwired: 1 out]
        n1074 = flat-sequence {
          tunnel: w955 -> [w997]
          tunnel: w954 -> [w996]
          tunnel: [w995] -> w947
          tunnel: [w994] -> w946
          tunnel: [w1000] -> w948
          tunnel: [w1001] -> w953
          tunnel: w947 -> [w1001]
          tunnel: w946 -> [w1000]
          frame #0 {
            w991 = u8 0
            w992 = u16 0 ("AudioLeft_phase_inc")
            w993 = FALSE
            n1075 = xnode "Read/Write Control"("FPGA VI Reference In"=w997, "error in"=w996, "Counts_Reset"=TRUE, "audioTrigger_L"=w993, "audioFreq_L_kHz"=w991, "audioAmp_L"=w992, "audioTrigger_R"=w993, "audioFreq_R_kHz"=w991, "audioAmp_R"=w992, "A3_SL"=w993, "A1_SR"=w993, "A6_Act"=w993) -> ("FPGA VI Reference Out"=w995:refnum<k20>, "error out"=w994:errorcluster)
          }
          frame #1 {
            w999 = FALSE ("START")
            n1076 = local write "START"(w999) -> ()
            n1077 = local write "STOP_endTrial"(w999) -> ()
            n1078 = local write "STOP_endBlock"(w999) -> ()
          }
        }
        n1079 = stacked-sequence {
          tunnel: w931 -> [w971 _]
          tunnel: w929 -> [w972 _]
          tunnel: w928 -> [_ w977]
          tunnel: w927 -> [_ w976]
          tunnel: w926 -> [_ w975]
          tunnel: w925 -> [w965 _]
          tunnel: w898 -> [w962 _]
          tunnel: w897 -> [w961 _]
          frame #0 {
            n1080 = call "myRIO_BRig_RT_dataCurrent_idxDataLick.vi"() -> ("output_idxDataLick"=w966:i32)  [unwired: 11 in]
            n1081 = Index Array(array=w965, index=w966) -> (element=w968:u16)
            n1082 = Array Subset(array=w962, length (row)=w961) -> (w963:u16[][])  [unwired: 3 in]
            n1083 = Increment(x=w968) -> (x+1=w969:u16)
            n1084 = call "myRIO_BRig_RT_comm_webdav_saveArrayToFile__1D_u16.vi"("Array"=w972, "input_filename"="dataMTrig") -> ()  [unwired: 10 in]
            n1085 = To Long Integer(number=w969) -> (32bit integer=w967:i32)
            n1086 = Array Subset(array=w971, length (row)=w967) -> (w970:u16[][])  [unwired: 3 in]
            n1087 = call "myRIO_BRig_RT_comm_webdav_saveArrayToFile__2D_u16.vi"("Array"=w970, "input_filename"="dataLick") -> ()  [unwired: 10 in]
            n1088 = call "myRIO_BRig_RT_comm_webdav_saveArrayToFile__2D_u16.vi"("Array"=w963, "input_filename"="dataAnalog") -> ()  [unwired: 10 in]
          }
          frame #1 {
            n1089 = case shown="True" w977 {
              tunnel: w976 -> [_ w979]
              tunnel: w975 -> [_ w978]
              frame False {
              }
              frame True {
                n1090 = stacked-sequence {
                  tunnel: w979 -> [w981 w988 w990]
                  tunnel: w978 -> [w982 w987 _]
                  frame #0 {
                    n1091 = call "myRIO_BRig_RT_comm_webdav_uploadFile__announce.vi"("input_addText"=TRUE, "input_fileName_prefix"=w982, "intput_fileName"="curExp_end", "intput_hSession"=w981) -> ("output_Isuccess"=w980:bool)  [unwired: 6 in, 1 out]
                    n1092 = case shown="True" w980 {
                      frame False {
                        n1093 = One Button Dialog(message="!!! Warning !!! Your data is located at C:\\BehaviorRig\\commTransfer") -> ()  [unwired: 1 in, 1 out]
                      }
                      frame True {
                        n1094 = Wait (ms)(milliseconds to wait=u32 20) -> ()  [unwired: 1 out]
                      }
                    }
                  }
                  frame #1 {
                    n1095 = call "myRIO_BRig_RT__endExp_sendData.vi"("input_fileName_prefix"=w987, "input_hSession"=w988) -> ()  [unwired: 8 in, 2 out]
                  }
                  frame #2 {
                    n1096 = local write "Connected To Host?"(FALSE ("Connected To Host?")) -> ()
                    n1097 = call <vilib>:"Close Session.vi"("session handle"=w990) -> ()  [unwired: 14 in, 1 out]
                  }
                }
              }
            }
          }
        }
      }
    }
    n1098 = local read "STOP_abort"() -> (w30:bool)
  }
  n1099 = xnode "Read/Write Control"("FPGA VI Reference In"=w8, "error in"=w7, "FPGA_Stop"=TRUE) -> ("FPGA VI Reference Out"=w13:refnum<k20>, "error out"=w14:errorcluster)
  n1100 = xnode "Close FPGA VI Reference"("FPGA VI Reference In"=w13, "error in"=w14) -> ("error out"=w12:errorcluster)
  n1101 = call <vilib>:"Reset myRIO.vi"("error in (no error)"=w12) -> ()  [unwired: 10 in, 1 out]
